vi "TelemetryPRO.vi"() -> ()   [LabVIEW 2017]
uses:
  <vilib>/nican/nican.llb/ncNetAttr.ctl
  <vilib>/Utility/file.llb/Read From Spreadsheet File (string).vi
  <vilib>/Utility/file.llb/Write To Spreadsheet File (string).vi
panel:
  out "Fz Estimation":cluster{i32, i32, i32, i32}(graph)
  out "Array":u8[](array[numeric])
  out "Numeric 2":u8
  out "SlipControl_Enabled":bool
  out "AMK_AV":bool
  out "Torque 2":bool
  out "Offset":i16
  out "Rear Reduction":dbl
  out "BreakPoint":u8
  out "Slope":u16
  out "Damper Travel FR [mm]":dbl
  out "Damper Travel RR [mm]":dbl
  out "Damper Travel FL [mm]":dbl
  in  "Wheel Travel FR":dbl=1000.0
  in  "Wheel Travel FL Offset":dbl=1000.0
  in  "Wheel Travel RR Offset":dbl=1000.0
  out "Damper Travel RL [mm]":dbl
  in  "Wheel Travel RL Offset":dbl=1000.0
  out "HV Cell Voltage":u16(graph)
  out "accY 2":dbl
  out "accZ 2":dbl
  out "TorqRaw 2":u16
  in  "Brake Min 3":dbl=426.0
  out "BPRV":bool
  out "BPFV":bool
  out "BPPS1V":bool
  out "BPPS2V":bool
  out "STA2":bool
  out "STA1":bool
  out "TPS2V":bool
  out "TPS1V":bool
  out "Apps2":dbl
  out "Apps1":dbl
  out "APPS1":u8(slide) scale=0.0..100.0
  out "APPS2":u8(slide) scale=0.0..100.0
  out "brake2":dbl
  out "brake1":dbl
  out "Brake1":u8(slide) scale=0.0..100.0
  out "Brake2":u8(slide) scale=0.0..100.0
  out "Status LEDs Red":bool[](array[boolean])
  out "Status LEDs Green":bool[](array[boolean])
  out "Numeric":dbl
  out "TCU speed":cluster{dbl, "AccelXRaw":dbl, dbl}(graph)
  out "AccelYRaw":dbl
  out "AccelXRaw":dbl
  in  "Acc Y offset":dbl
  in  "Acc X offset 2":dbl
  in  "OffsetFilter":dbl=0.01
  out "IsStopped":bool
  out "Acc Z 2":dbl
  out "Acc X 2":dbl
  out "Roll 2":dbl
  out "Acc Y 2":dbl
  out "Yaw 2":dbl
  in  "Acc Z offset":dbl
  out "Vel_acc":dbl=-0.0098098
  in  "New Lap":bool
  out "Energy":dbl[](array[numeric])
  out "Wheel Travel FL":u16
  out "Wheel Travel FR":u16
  out "Wheel Travel RL":u16
  out "Wheel Travel RR":u16
  out "Acc X":dbl
  out "Roll":dbl
  out "Yaw":dbl
  out "Acc Y":dbl
  out "Acc Z":dbl
  out "accY":dbl
  out "accZ":dbl
  out "Intensity Graph":dbl[][](graph)
  in  "Rollrate offset":dbl
  out "XY Graph 2":cluster{dbl[], dbl[]}(graph)
  out "Derate":bool[](array[boolean])
  out "Torq_sum":dbl
  in  "Play":bool
  in  "Timestep":u32
  in  "stop":bool
  in  "start":bool
  in  "pause":bool
  in  "Progress":i32(slide) min=0 step=60 scale=-1.0..61354011.0 scale format="%.0p"
  out "Time Stamp":string="2\r\n60"
  out "Charge Voltage":dbl
  out "Charge Curr":dbl
  in  "Tab Control":T1(tab)
  in  "Rows to read":i32=60
  in  "Data Path":path=path "D:/__BME-FRT/2016/2016-05-19/2016_05_19_tokol_endurance_00005_00001.csv"
  in  "CAN1 Enable":bool
  in  "CAN0 Enable":bool
  in  "Data Source":u16(ring) items=["Wi-Fi", "CAN-USB", "Log Analysis"]
  in  "Port":u16=8998
  in  "Exit":bool
  in  "Log Path":path=path "D:/__BME-FRT/2016/test.txt"
  in  "Log Enable":bool
  out "WiFi Error":errorcluster
  in  "Length":u16=10
  out "CAN0 Error":errorcluster
  out "CAN1 Error":errorcluster
  out "Log Error":errorcluster
  out "CAN Message":u8[][](array[numeric])=[[2, 1, 128, 63, 0, 0, 129, 162, 129, 155], [2, 17, 23, 61, 0, 1, 0, 0, 0, 0], [3, 64, 252, 0, 0, 0, 27, 55, 27, 0], [2, 16, 115, 16, 37, 0, 203, 0, 0, 0], [4, 17, 23, 61, 0, 1, 0, 0, 0, 0], [2, 0, 128, 44, 0, 0, 136, 1, 7, 207], [2, 1, 128, 63, 0, 0, 129, 162, 129, 155], [2, 17, 23, 61, 0, 1, 0, 0, 0, 0], [4, 34, 0, 33, 0, 30, 0, 0, 0, 0], [4, 80, 148, 60, 128, 0, 0, 0, 0, 0], [1, 116, 84, 128, 0, 0, 190, 127, 8, 37], [2, 16, 116, 15, 111, 0, 203, 0, 0, 0], [1, 120, 211, 127, 0, 0, 193, 158, 8, 215], [1, 180, 84, 128, 0, 0, 223, 126, 2, 100], [1, 124, 0, 0, 0, 0, 189, 126, 8, 75], [1, 184, 62, 128, 2, 15, 59, 127, 2, 219], [4, 17, 23, 61, 0, 1, 0, 0, 0, 0], [1, 188, 0, 0, 0, 0, 136, 158, 2, 110], [2, 0, 128, 44, 0, 0, 136, 1, 7, 207], [2, 1, 128, 63, 0, 0, 129, 162, 129, 155], [2, 17, 23, 61, 0, 1, 0, 0, 0, 0], [3, 64, 252, 0, 0, 0, 27, 55, 27, 0], [4, 48, 10, 15, 219, 0, 96, 0, 0, 0], [3, 49, 128, 255, 0, 0, 0, 0, 0, 0], [2, 16, 117, 0, 0, 0, 203, 0, 0, 0], [4, 17, 23, 61, 0, 1, 0, 0, 0, 0], [2, 0, 128, 44, 0, 0, 136, 1, 7, 207], [2, 1, 128, 63, 0, 0, 129, 162, 129, 155], [2, 17, 23, 61, 0, 1, 0, 0, 0, 0], [3, 32, 112, 255, 0, 0, 0, 0, 0, 0], [4, 34, 0, 30, 0, 31, 0, 0, 0, 0], [1, 116, 87, 128, 0, 0, 184, 127, 9, 218], [1, 120, 203, 127, 1, 37, 194, 158, 9, 222], [2, 16, 118, 0, 0, 0, 205, 0, 0, 0], [1, 124, 0, 0, 0, 0, 176, 126, 9, 211], [1, 180, 90, 128, 0, 0, 215, 126, 3, 116], [1, 184, 50, 128, 3, 19, 44, 127, 3, 114], [4, 17, 23, 61, 0, 1, 0, 0, 0, 0], [1, 188, 0, 0, 0, 0, 147, 158, 3, 235], [2, 0, 128, 43, 0, 0, 136, 1, 7, 207], [2, 1, 128, 63, 0, 0, 129, 162, 129, 155], [2, 17, 23, 61, 0, 1, 0, 0, 0, 0], [3, 64, 252, 0, 0, 0, 38, 55, 38, 0], [2, 16, 119, 0, 0, 0, 202, 0, 0, 0], [4, 17, 23, 61, 0, 1, 0, 0, 0, 0], [2, 0, 128, 43, 0, 0, 136, 2, 7, 207], [2, 1, 128, 63, 0, 0, 129, 162, 129, 155], [2, 17, 23, 61, 0, 1, 0, 0, 0, 0], [4, 34, 0, 20, 0, 26, 0, 0, 0, 0], [1, 116, 78, 128, 0, 0, 179, 127, 10, 75], [1, 120, 206, 127, 2, 57, 194, 158, 10, 132], [2, 16, 120, 16, 37, 0, 200, 0, 210, 0], [1, 180, 90, 128, 0, 0, 206, 126, 4, 188], [1, 124, 0, 0, 0, 0, 157, 126, 10, 65], [1, 184, 39, 128, 4, 3, 33, 127, 4, 7], [4, 17, 23, 61, 0, 1, 0, 0, 0, 0], [1, 188, 0, 0, 0, 0, 153, 158, 4, 183], [2, 0, 128, 43, 0, 0, 136, 2, 7, 207], [2, 1, 128, 63, 0, 0, 129, 162, 129, 155], [2, 17, 23, 61, 0, 1, 0, 0, 0, 0]] format="%02x"
  out "CAN ID":u16[](array[numeric])=[513, 529, 832, 528, 1041, 512, 513, 529, 1058, 1104, 372, 528, 376, 436, 380, 440, 1041, 444, 512, 513, 529, 832, 1072, 817, 528, 1041, 512, 513, 529, 800, 1058, 372, 376, 528, 380, 436, 440, 1041, 444, 512, 513, 529, 832, 528, 1041, 512, 513, 529, 1058, 372, 376, 528, 436, 380, 440, 1041, 444, 512, 513, 529] format="%x"
  out "CAN Message 2":u8[][](array[numeric])=[[2, 1, 128, 63, 0, 0, 129, 162, 129, 155], [2, 17, 23, 61, 0, 1, 0, 0, 0, 0], [3, 64, 252, 0, 0, 0, 27, 55, 27, 0], [2, 16, 115, 16, 37, 0, 203, 0, 0, 0], [4, 17, 23, 61, 0, 1, 0, 0, 0, 0], [2, 0, 128, 44, 0, 0, 136, 1, 7, 207], [2, 1, 128, 63, 0, 0, 129, 162, 129, 155], [2, 17, 23, 61, 0, 1, 0, 0, 0, 0], [4, 34, 0, 33, 0, 30, 0, 0, 0, 0], [4, 80, 148, 60, 128, 0, 0, 0, 0, 0], [1, 116, 84, 128, 0, 0, 190, 127, 8, 37], [2, 16, 116, 15, 111, 0, 203, 0, 0, 0], [1, 120, 211, 127, 0, 0, 193, 158, 8, 215], [1, 180, 84, 128, 0, 0, 223, 126, 2, 100], [1, 124, 0, 0, 0, 0, 189, 126, 8, 75], [1, 184, 62, 128, 2, 15, 59, 127, 2, 219], [4, 17, 23, 61, 0, 1, 0, 0, 0, 0], [1, 188, 0, 0, 0, 0, 136, 158, 2, 110], [2, 0, 128, 44, 0, 0, 136, 1, 7, 207], [2, 1, 128, 63, 0, 0, 129, 162, 129, 155], [2, 17, 23, 61, 0, 1, 0, 0, 0, 0], [3, 64, 252, 0, 0, 0, 27, 55, 27, 0], [4, 48, 10, 15, 219, 0, 96, 0, 0, 0], [3, 49, 128, 255, 0, 0, 0, 0, 0, 0], [2, 16, 117, 0, 0, 0, 203, 0, 0, 0], [4, 17, 23, 61, 0, 1, 0, 0, 0, 0], [2, 0, 128, 44, 0, 0, 136, 1, 7, 207], [2, 1, 128, 63, 0, 0, 129, 162, 129, 155], [2, 17, 23, 61, 0, 1, 0, 0, 0, 0], [3, 32, 112, 255, 0, 0, 0, 0, 0, 0], [4, 34, 0, 30, 0, 31, 0, 0, 0, 0], [1, 116, 87, 128, 0, 0, 184, 127, 9, 218], [1, 120, 203, 127, 1, 37, 194, 158, 9, 222], [2, 16, 118, 0, 0, 0, 205, 0, 0, 0], [1, 124, 0, 0, 0, 0, 176, 126, 9, 211], [1, 180, 90, 128, 0, 0, 215, 126, 3, 116], [1, 184, 50, 128, 3, 19, 44, 127, 3, 114], [4, 17, 23, 61, 0, 1, 0, 0, 0, 0], [1, 188, 0, 0, 0, 0, 147, 158, 3, 235], [2, 0, 128, 43, 0, 0, 136, 1, 7, 207], [2, 1, 128, 63, 0, 0, 129, 162, 129, 155], [2, 17, 23, 61, 0, 1, 0, 0, 0, 0], [3, 64, 252, 0, 0, 0, 38, 55, 38, 0], [2, 16, 119, 0, 0, 0, 202, 0, 0, 0], [4, 17, 23, 61, 0, 1, 0, 0, 0, 0], [2, 0, 128, 43, 0, 0, 136, 2, 7, 207], [2, 1, 128, 63, 0, 0, 129, 162, 129, 155], [2, 17, 23, 61, 0, 1, 0, 0, 0, 0], [4, 34, 0, 20, 0, 26, 0, 0, 0, 0], [1, 116, 78, 128, 0, 0, 179, 127, 10, 75], [1, 120, 206, 127, 2, 57, 194, 158, 10, 132], [2, 16, 120, 16, 37, 0, 200, 0, 210, 0], [1, 180, 90, 128, 0, 0, 206, 126, 4, 188], [1, 124, 0, 0, 0, 0, 157, 126, 10, 65], [1, 184, 39, 128, 4, 3, 33, 127, 4, 7], [4, 17, 23, 61, 0, 1, 0, 0, 0, 0], [1, 188, 0, 0, 0, 0, 153, 158, 4, 183], [2, 0, 128, 43, 0, 0, 136, 2, 7, 207], [2, 1, 128, 63, 0, 0, 129, 162, 129, 155], [2, 17, 23, 61, 0, 1, 0, 0, 0, 0]] format="%02x"
  out "CAN ID 2":u16[](array[numeric])=[513, 529, 832, 528, 1041, 512, 513, 529, 1058, 1104, 372, 528, 376, 436, 380, 440, 1041, 444, 512, 513, 529, 832, 1072, 817, 528, 1041, 512, 513, 529, 800, 1058, 372, 376, 528, 380, 436, 440, 1041, 444, 512, 513, 529, 832, 528, 1041, 512, 513, 529, 1058, 372, 376, 528, 436, 380, 440, 1041, 444, 512, 513, 529] format="%x"
  out "CAN Message 3":u8[][](array[numeric])=[[2, 1, 128, 63, 0, 0, 129, 162, 129, 155], [2, 17, 23, 61, 0, 1, 0, 0, 0, 0], [3, 64, 252, 0, 0, 0, 27, 55, 27, 0], [2, 16, 115, 16, 37, 0, 203, 0, 0, 0], [4, 17, 23, 61, 0, 1, 0, 0, 0, 0], [2, 0, 128, 44, 0, 0, 136, 1, 7, 207], [2, 1, 128, 63, 0, 0, 129, 162, 129, 155], [2, 17, 23, 61, 0, 1, 0, 0, 0, 0], [4, 34, 0, 33, 0, 30, 0, 0, 0, 0], [4, 80, 148, 60, 128, 0, 0, 0, 0, 0], [1, 116, 84, 128, 0, 0, 190, 127, 8, 37], [2, 16, 116, 15, 111, 0, 203, 0, 0, 0], [1, 120, 211, 127, 0, 0, 193, 158, 8, 215], [1, 180, 84, 128, 0, 0, 223, 126, 2, 100], [1, 124, 0, 0, 0, 0, 189, 126, 8, 75], [1, 184, 62, 128, 2, 15, 59, 127, 2, 219], [4, 17, 23, 61, 0, 1, 0, 0, 0, 0], [1, 188, 0, 0, 0, 0, 136, 158, 2, 110], [2, 0, 128, 44, 0, 0, 136, 1, 7, 207], [2, 1, 128, 63, 0, 0, 129, 162, 129, 155], [2, 17, 23, 61, 0, 1, 0, 0, 0, 0], [3, 64, 252, 0, 0, 0, 27, 55, 27, 0], [4, 48, 10, 15, 219, 0, 96, 0, 0, 0], [3, 49, 128, 255, 0, 0, 0, 0, 0, 0], [2, 16, 117, 0, 0, 0, 203, 0, 0, 0], [4, 17, 23, 61, 0, 1, 0, 0, 0, 0], [2, 0, 128, 44, 0, 0, 136, 1, 7, 207], [2, 1, 128, 63, 0, 0, 129, 162, 129, 155], [2, 17, 23, 61, 0, 1, 0, 0, 0, 0], [3, 32, 112, 255, 0, 0, 0, 0, 0, 0], [4, 34, 0, 30, 0, 31, 0, 0, 0, 0], [1, 116, 87, 128, 0, 0, 184, 127, 9, 218], [1, 120, 203, 127, 1, 37, 194, 158, 9, 222], [2, 16, 118, 0, 0, 0, 205, 0, 0, 0], [1, 124, 0, 0, 0, 0, 176, 126, 9, 211], [1, 180, 90, 128, 0, 0, 215, 126, 3, 116], [1, 184, 50, 128, 3, 19, 44, 127, 3, 114], [4, 17, 23, 61, 0, 1, 0, 0, 0, 0], [1, 188, 0, 0, 0, 0, 147, 158, 3, 235], [2, 0, 128, 43, 0, 0, 136, 1, 7, 207], [2, 1, 128, 63, 0, 0, 129, 162, 129, 155], [2, 17, 23, 61, 0, 1, 0, 0, 0, 0], [3, 64, 252, 0, 0, 0, 38, 55, 38, 0], [2, 16, 119, 0, 0, 0, 202, 0, 0, 0], [4, 17, 23, 61, 0, 1, 0, 0, 0, 0], [2, 0, 128, 43, 0, 0, 136, 2, 7, 207], [2, 1, 128, 63, 0, 0, 129, 162, 129, 155], [2, 17, 23, 61, 0, 1, 0, 0, 0, 0], [4, 34, 0, 20, 0, 26, 0, 0, 0, 0], [1, 116, 78, 128, 0, 0, 179, 127, 10, 75], [1, 120, 206, 127, 2, 57, 194, 158, 10, 132], [2, 16, 120, 16, 37, 0, 200, 0, 210, 0], [1, 180, 90, 128, 0, 0, 206, 126, 4, 188], [1, 124, 0, 0, 0, 0, 157, 126, 10, 65], [1, 184, 39, 128, 4, 3, 33, 127, 4, 7], [4, 17, 23, 61, 0, 1, 0, 0, 0, 0], [1, 188, 0, 0, 0, 0, 153, 158, 4, 183], [2, 0, 128, 43, 0, 0, 136, 2, 7, 207], [2, 1, 128, 63, 0, 0, 129, 162, 129, 155], [2, 17, 23, 61, 0, 1, 0, 0, 0, 0]] format="%02x"
  out "CAN ID 3":u16[](array[numeric])=[513, 529, 832, 528, 1041, 512, 513, 529, 1058, 1104, 372, 528, 376, 436, 380, 440, 1041, 444, 512, 513, 529, 832, 1072, 817, 528, 1041, 512, 513, 529, 800, 1058, 372, 376, 528, 380, 436, 440, 1041, 444, 512, 513, 529, 832, 528, 1041, 512, 513, 529, 1058, 372, 376, 528, 436, 380, 440, 1041, 444, 512, 513, 529] format="%x"
  out "STA2":i16
  out "STA1":i16
  out "Max Power":u8
  out "TPS1_Raw":u16
  out "BPS1_Raw":u16
  out "K_Brake":dbl
  out "PD Error Info":u8
  out "Velocity [km/h]":dbl(knob) scale=0.0..120.0
  out "CAN Missing Message":u8[](array[numeric])
  out "Rear 2":dbl
  out "Front 2":dbl
  out "TCU FR":dbl(graph)
  out "TCU RR":dbl(graph)
  out "TCU FL":dbl(graph)
  out "Rear":dbl
  out "Front":dbl
  out "Torque":dbl(slide) scale=0.0..100.0
  out "Brake Encoder":dbl(slide) scale=0.0..100.0
  out "FL":dbl(slide) scale=0.0..2330.0
  in  "Torque Min":dbl
  in  "Torque Max":dbl=1000.0
  in  "Brake Min":dbl
  in  "Brake Max":dbl=1000.0
  out "FL 2":dbl(slide)
  out "FR":dbl(slide) scale=0.0..2330.0
  out "FR 2":dbl(slide)
  out "RL":dbl(slide) scale=0.0..2330.0
  out "RL 2":dbl(slide)
  out "RR":dbl(slide) scale=0.0..2330.0
  out "RR 2":dbl(slide)
  out "Sensor Check":bool[](array[boolean])
  out "Brake Front":dbl(slide)=-0.5082592121982211 scale=0.0..100.0
  out "Brake Rear":dbl(slide)=-0.9529860228716646 scale=0.0..100.0
  in  "Brake Min 2":dbl=350.0
  in  "Brake Max 2":dbl=2000.0
  out "TorqRaw":u16
  out "BrakeRaw":u16
  out "BrakeRaw 2":u16
  out "Boolean":bool
  out "Boolean 2":bool
  out "Boolean 3":bool
  out "Boolean 4":bool
  out "Dial":dbl(knob)=3.0 scale=1.0..12.0
  out "Dial 2":dbl(knob)=11.0 scale=1.0..12.0
  out "Dial 3":dbl(knob)=9.0 scale=1.0..12.0
  out "Dial 4":dbl(knob)=1.0 scale=1.0..12.0
  out "Dial 5":dbl(knob)=1.0 scale=1.0..12.0
  out "Selector":u8
  out "Torque %":u8
  out "Speed RPM":i16
  out "LR Bias":dbl
  out "Regen %":u8
  out "BTC":u8
  out "TCU RR Status":bool[](array[boolean])
  out "TCU RL Status":bool[](array[boolean])
  out "TCU FR Status":bool[](array[boolean])
  out "TCU FL Status":bool[](array[boolean])
  out "Torque [Nm]":dbl(knob) scale=-500.0..1250.0
  out "XY Graph":cluster{dbl[], dbl[]}[](graph)
  out "TCU RL":dbl(graph)
  out "K_Throttle":dbl
  out "BPS2_Raw":u16
  out "BPF_Raw":u16
  out "BPR_Raw":u16
  out "TPS2_Raw":u16
  out "STA2_Raw":u16
  out "STA1_Raw":u16
  out "OFF":bool=TRUE
  out "START":bool
  out "ON":bool
  out "Logging":bool
  in  "Steering Null":dbl=1919.0
  in  "Steering Min":dbl=174.0
  in  "Steering Max":dbl=3565.0
  out "Steering Angle":dbl(slide)=-0.10285714285714287 scale=90.0..-90.0
  out "SteeringRaw":u16
  out "TCU Version":u16
  out "Safety Mode Enabled":bool
  out "Keylock Enable":bool
  out "Slip_TCU":cluster{dbl, dbl, dbl, dbl}(graph)
  out "TCU_acc":cluster{dbl[], dbl[]}[](graph)
  out "Slip":cluster{dbl, dbl, dbl, dbl}(graph)
  out "TCU_ay":dbl
  out "TCU_v":dbl
  out "TCU_ax":dbl
  out "TCU_yaw":dbl
  out "TCU_slipFL":dbl
  out "TCU_slipFR":dbl
  out "TCU_slipRL":dbl
  out "TCU_slipRR":dbl
  out "FL Velocity":dbl
  out "FL Torque Pos":dbl
  out "FL Torque Neg":dbl
  out "FR Velocity":dbl
  out "FR Torque Pos":dbl
  out "FR Torque Neg":dbl
  out "RL Velocity":dbl
  out "RL Torque Pos":dbl
  out "RL Torque Neg":dbl
  out "RR Velocity":dbl
  out "RR Torque Pos":dbl
  out "RR Torque Neg":dbl
  out "MCU RR":cluster{dbl, dbl}(graph)={-0.487060546875, 0.57037353515625}
  out "MCU RL":cluster{dbl, dbl}(graph)={0.743408203125, -0.384521484375}
  out "MCU FR":cluster{dbl, dbl}(graph)={-0.25634765625, -0.205078125}
  out "MCU FL":cluster{dbl, dbl}(graph)={-0.16021728515625, 0.50628662109375}
  out "Actual Velocity\nFL [RPM]":i16
  out "Id FL [A]":dbl
  out "Iq FL [A]":dbl
  out "T Motor FL [°C]":dbl
  out "Error Info FL":u16
  out "Actual Velocity\nFR [RPM]":i16
  out "Id FR [A]":dbl
  out "Iq FR [A]":dbl
  out "Actual Velocity\nRL [RPM]":i16
  out "Id RL [A]":dbl
  out "Iq RL [A]":dbl
  out "Actual Velocity \nRR [RPM]":i16
  out "Id RR [A]":dbl
  out "Iq RR [A]":dbl
  out "Error Info FR":u16
  out "T Motor FR [°C]":dbl
  out "Error Info RL":u16
  out "T Motor RL [°C]":dbl
  out "Error Info RR":u16
  out "T Motor RR [°C]":dbl
  out "Status FL":bool[](array[boolean])
  out "Status FR":bool[](array[boolean])
  out "Status RL":bool[](array[boolean])
  out "Status RR":bool[](array[boolean])
  out "T Inv. FL [°C]":dbl
  out "T Inv. FR [°C]":dbl
  out "T Inv. RR [°C]":dbl
  out "T Inv. RL [°C]":dbl
  out "MCU SC Endline":bool
  out "HVD Interlock":bool
  out "Motor4 Interlock":bool
  out "Motor3 Interlock":bool
  out "Motor2 Interlock":bool
  out "Motor1 Interlock":bool
  out "SC LKS":bool
  out "SC RKS":bool
  out "SC MCU":bool
  out "SC 12V":bool
  out "SC BSPD":bool
  out "SC IMD":bool
  out "SC AMS":bool
  out "SC AIR-":bool
  out "SC AIR+":bool
  out "SC BOTS &\nINS & CKS":bool
  out "SC Motor 3":bool
  out "SC Motor 1":bool
  out "SC Motor 4":bool
  out "SC Motor 2":bool
  out "HVDet":bool
  out "AIR-":bool
  out "AIR+":bool
  out "BOTS & INS & CKS":bool
  out "MCU Interlocks":bool
  out "LKS & RKS":bool
  out "BSPD 5kW":bool
  out "AMS Relay":bool
  out "IMD Relay":bool
  out "BSPD Relay":bool
  out "BSPD Brake":bool
  out "SC Endline":bool
  out "Radiator Cooling":bool
  out "Battery Low":bool
  out "BMS IC Wake":bool
  out "BMS IC Fault":bool
  out "Battery Full":bool
  out "LV Undervoltage":bool
  out "LV Overtemp":bool
  out "SC State":bool
  out "Main Switch":bool
  out "MP Switch":bool
  out "Discharge":bool[](array[boolean])
  out "LV Temp":dbl[](array[numeric])
  out "LV Battery":cluster{"CellSlide":u16, "CellVoltage":u16}[](array[cluster])=[{"CellSlide"=0, "CellVoltage"=0}, {"CellSlide"=0, "CellVoltage"=0}, {"CellSlide"=0, "CellVoltage"=0}, {"CellSlide"=0, "CellVoltage"=0}, {"CellSlide"=0, "CellVoltage"=0}, {"CellSlide"=0, "CellVoltage"=0}, {"CellSlide"=0, "CellVoltage"=0}, {"CellSlide"=0, "CellVoltage"=0}, {"CellSlide"=0, "CellVoltage"=0}, {"CellSlide"=2800, "CellVoltage"=0}, {"CellSlide"=0, "CellVoltage"=0}, {"CellSlide"=0, "CellVoltage"=0}, {"CellSlide"=0, "CellVoltage"=0}, {"CellSlide"=0, "CellVoltage"=0}] {"CellSlide" scale=2800.0..4200.0}
  out "LV Temp":dbl
  out "LV Max":u16
  out "LV Min":u16
  out "LV Cell Voltages":T2(graph)
  out "Overtemp Errors":u16
  out "Undervoltage Errrors":u16
  out "LV Current":cluster{dbl, dbl}(graph)
  out "LV Voltage [V]":dbl format="%#.2g"
  out "12V Current [A]":dbl format="%#.1g"
  out "48V Current [A]":dbl format="%#.1g"
  out "48V system":bool[](array[boolean])
  out "12V system":bool[](array[boolean])
  out "Temp Max 2":dbl
  out "Cell Min 2":u16
  out "BSPD 5kW":bool
  out "BSPD Brake":bool
  out "HVDet":bool
  out "Stack 1":cluster{"CellSlide":u16, "CellVoltage":u16}[](array[cluster]) {"CellSlide" scale=2800.0..4200.0}
  out "Temp 1":dbl[](array[numeric])
  out "Cell Min":u16
  out "Cell Max":u16
  out "Temp Max":dbl
  out "HV Before":dbl
  out "HV After":dbl
  out "HV Current":dbl
  out "SoC [mAh]":dbl
  out "Stack 2":cluster{"CellSlide":u16, "CellVoltage":u16}[](array[cluster]) {"CellSlide" scale=2800.0..4200.0}
  out "Stack 3":cluster{"CellSlide":u16, "CellVoltage":u16}[](array[cluster]) {"CellSlide" scale=2800.0..4200.0}
  out "Stack 4":cluster{"CellSlide":u16, "CellVoltage":u16}[](array[cluster])=[{"CellSlide"=0, "CellVoltage"=0}, {"CellSlide"=0, "CellVoltage"=0}, {"CellSlide"=0, "CellVoltage"=0}, {"CellSlide"=0, "CellVoltage"=0}, {"CellSlide"=0, "CellVoltage"=0}, {"CellSlide"=0, "CellVoltage"=0}, {"CellSlide"=0, "CellVoltage"=0}, {"CellSlide"=0, "CellVoltage"=0}, {"CellSlide"=0, "CellVoltage"=0}, {"CellSlide"=0, "CellVoltage"=0}, {"CellSlide"=0, "CellVoltage"=0}, {"CellSlide"=0, "CellVoltage"=0}, {"CellSlide"=0, "CellVoltage"=0}, {"CellSlide"=0, "CellVoltage"=0}, {"CellSlide"=0, "CellVoltage"=0}, {"CellSlide"=0, "CellVoltage"=0}, {"CellSlide"=0, "CellVoltage"=0}, {"CellSlide"=0, "CellVoltage"=0}, {"CellSlide"=0, "CellVoltage"=0}, {"CellSlide"=0, "CellVoltage"=0}, {"CellSlide"=0, "CellVoltage"=0}, {"CellSlide"=0, "CellVoltage"=0}, {"CellSlide"=2800, "CellVoltage"=0}, {"CellSlide"=2800, "CellVoltage"=0}] {"CellSlide" scale=2800.0..4200.0}
  out "Stack 5":cluster{"CellSlide":u16, "CellVoltage":u16}[](array[cluster])=[{"CellSlide"=2800, "CellVoltage"=0}, {"CellSlide"=0, "CellVoltage"=0}, {"CellSlide"=0, "CellVoltage"=0}, {"CellSlide"=0, "CellVoltage"=0}, {"CellSlide"=0, "CellVoltage"=0}, {"CellSlide"=0, "CellVoltage"=0}, {"CellSlide"=0, "CellVoltage"=0}, {"CellSlide"=0, "CellVoltage"=0}, {"CellSlide"=0, "CellVoltage"=0}, {"CellSlide"=0, "CellVoltage"=0}, {"CellSlide"=0, "CellVoltage"=0}, {"CellSlide"=0, "CellVoltage"=0}, {"CellSlide"=0, "CellVoltage"=0}, {"CellSlide"=0, "CellVoltage"=0}, {"CellSlide"=0, "CellVoltage"=0}, {"CellSlide"=0, "CellVoltage"=0}, {"CellSlide"=0, "CellVoltage"=0}, {"CellSlide"=0, "CellVoltage"=0}, {"CellSlide"=0, "CellVoltage"=0}, {"CellSlide"=0, "CellVoltage"=0}, {"CellSlide"=0, "CellVoltage"=0}, {"CellSlide"=0, "CellVoltage"=0}, {"CellSlide"=0, "CellVoltage"=0}, {"CellSlide"=0, "CellVoltage"=0}] {"CellSlide" scale=2800.0..4200.0}
  out "Stack 6":cluster{"CellSlide":u16, "CellVoltage":u16}[](array[cluster]) {"CellSlide" scale=2800.0..4200.0}
  out "Temp 2":dbl[](array[numeric])
  out "Temp 3":dbl[](array[numeric])
  out "Temp 4":dbl[](array[numeric])
  out "Temp 5":dbl[](array[numeric])
  out "Temp 6":dbl[](array[numeric])
  out "TSAL State":bool
  out "PC State":bool
  out "12V State":bool
  out "AMS error":bool
  out "IMD error":bool
  out "AMS Relay 2":bool
  out "IMD Relay":bool
  out "AIR+":bool
  out "AIR-":bool
  out "BSPD Relay":bool
  out "UV":bool
  out "OV":bool
  out "OT":bool
  out "TS-OV":bool
  out "Place of Error":u16
  out "Value":u16
  out "?":T3(graph)
  out "Angular Speed":T4(graph)
  out "Pedal Signals":cluster{u16, "BrakeRaw":u16}(graph)
  out "Brake Pressure":cluster{dbl, dbl}(graph)={-0.28368794326241137, -0.5319148936170213}
  out "XY Graph 3":cluster{dbl[], dbl[]}[](graph)
  out "HV Cell":cluster{"Cell Max":u16, "Cell Min":u16}(graph)
  out "Current":dbl(graph)
  out "Electric Power":cluster{dbl, dbl}(graph)
  out "HV Voltage":cluster{"HV Before":dbl, "HV After":dbl}(graph)={"HV Before"=594.9, "HV After"=0.1}
  out "HV Cell Temperature":cluster{dbl, dbl}(graph)
  out "Motor Temperature":cluster{dbl, dbl, dbl, dbl}(graph)={1.3, 1.3, 1.6, 1.5}
  out "Inverter Temperature":cluster{dbl, dbl, dbl, dbl}(graph)={1.3, 1.3, 1.6, 1.5}
  out "Radiator Temperature":T5(graph)
  out "S Radiator Left IN":dbl
  out "S Radiator Right OUT":dbl
  out "S Radiator Right IN":dbl
  out "S Radiator Left OUT":dbl
  out "Car standing":bool
  out "SC State":bool
  out "Overvoltage":bool
  out "MODE":bool
  out "XLAT":bool
  out "BLANK":bool
  out "MCU S SC Endl":u16
  out "TSAL":bool
  out "Telemetry":bool
  out "OFF":bool
  out "START":bool
  out "24V rear DC/DC":bool
  out "OFF Button":bool
  out "START Button":bool
  out "ON Button":bool
  out "Power B Current":u32
  out "Power A Current":u32
  out "CAN2 Term.":bool
  out "CAN1 Term.":bool
  out "MCU TSAL":bool
  out "MCU SC Endline 2":bool
  out "MCU FL 4":bool
  out "MCU FL 3":bool
  out "MCU FL 2":bool
  out "Brake Pausability":bool
  out "MCU RF 4":bool
  out "MCU RF 3":bool
  out "MCU RF 2":bool
  out "MCU RF 1":bool
  out "MCU EF2 B":bool
  out "MCU EF2 A":bool
  out "MCU EF B":bool
  out "MCU EF A":bool
  out "24V Power B":bool
  out "Braking":bool
  out "STA2 ADC Null":u16
  out "STA1 ADC Null":u16
  out "Battery Low":bool
  out "BMS IC Awake":bool
  out "BMS IC Error":bool
  out "Battery Full":bool
  out "48V Out 3":bool
  out "LV Undervoltage":bool
  out "LV Overtemp":bool
  out "12V Out 2":bool
  out "12V Out 3":bool
  out "SC State":bool
  out "12V Out 1":bool
  out "Main Switch":bool
  out "MP Switch":bool
  out "12V Out 5":bool
  out "12V Out 4":bool
  out "48V Out 2":bool
  out "48V Out 1":bool
  out "ON":bool
  out "24V front DC/DC":bool
  out "MCU Interlock":bool
  out "TCU Power":bool
  out "RTDS":bool
  out "LKS & RKS":bool
  out "Brake Light":bool
  out "STA2 ADC 90":u16
  out "STA1 ADC 90":u16
  out "BSE2 ADC Max":u16
  out "BSE2 ADC Min":u16
  out "BSE1 ADC Max":u16
  out "BSE1 ADC Min":u16
  out "APPS2 ADC Max":u16
  out "APPS2 ADC Min":u16
  out "APPS1 ADC Max":u16
  out "APPS1 ADC Min":u16
  out "MCU EF":bool
  out "MCU RF":bool
  out "MCU Radiator Left IN":dbl
  out "MCU Radiator Right OUT":dbl
  out "MCU Radiator Right IN":dbl
  out "MCU Radiator Left OUT":dbl
  out "TSAL State 2":bool
  out "PC State 2":bool
  out "Driver Protection":bool
  out "12V Current [mA]":dbl
  out "48V Current [mA]":dbl
  out "Message Arrived 14":bool
  out "Message Arrived 13":bool
  out "Message Arrived 12":bool
  out "Message Arrived 11":bool
  out "Other messages arrived":bool
  out "Message Arrived 2":bool
  out "Message Arrived":bool
  out "RR TargetVelo OverTresh":bool
  out "RR TorqueLimNeg UnderTresh":bool
  out "RR TorqueLimNeg OverTresh":bool
  out "RR TorqueLimPos UnderTresh":bool
  out "RR TorqueLimPos OverTresh":bool
  out "RR TargetVelo UnderTresh":bool
  out "RL TargetVelo OverTresh":bool
  out "RL TorqueLimNeg UnderTresh":bool
  out "RL TorqueLimNeg OverTresh":bool
  out "RL TorqueLimPos UnderTresh":bool
  out "RL TorqueLimPos OverTresh":bool
  out "RL TargetVelo UnderTresh":bool
  out "FR TargetVelo OverTresh":bool
  out "FR TorqueLimNeg UnderTresh":bool
  out "FR TorqueLimNeg OverTresh":bool
  out "FR TorqueLimPos UnderTresh":bool
  out "FR TorqueLimPos OverTresh":bool
  out "FR TargetVelo UnderTresh":bool
  out "FL TargetVelo OverTresh":bool
  out "FL TorqueLimNeg UnderTresh":bool
  out "FL TorqueLimNeg OverTresh":bool
  out "FL TorqueLimPos UnderTresh":bool
  out "FL TorqueLimPos OverTresh":bool
  out "FL TargetVelo UnderTresh":bool
  out "Error Throttle Plausability":bool
  out "Error Throttle Validity 2":bool
  out "Error Throttle Validity 1":bool
  out "Error Throttle Position 2":bool
  out "Error Throttle Position 1":bool
  out "Error Rot Switch 5":bool
  out "Error Rot Switch 4":bool
  out "Error Rot Switch 3":bool
  out "Error Rot Switch 2":bool
  out "Error Rot Switch 1":bool
  out "Error Pedalbox Heartbeat":bool
  out "Error Steering Heartbeat":bool
  out "Error Brake Plausability":bool
  out "Error Brake Validity 2":bool
  out "Error Brake Validity  1":bool
  out "Error Brake Position 2":bool
  out "Error Brake Position 1":bool
  out "Error_Button_4":bool
  out "Error_Button_3":bool
  out "Error_Button_2":bool
  out "Error_Button_1":bool
  out "Error Steering Plausability":bool
  out "Error Steering Validity 2":bool
  out "Error Steering Validity 1":bool
  out "Error Steering Angle 2":bool
  out "Error Steering Angle 1":bool
  out "Error Cell Temperature":bool
  out "Error Cell Voltage Sensor":bool
  out "Error Cell Voltage":bool
  out "Error HV Accu. Current":bool
  out "Error HV Accu. Voltage":bool
  out "Error Actual Velocity RR":bool
  out "Error Actual Velocity RL":bool
  out "Error Actual Velocity FR":bool
  out "Error Actual Velocity FL":bool
  out "Error_SteeringControl_Heartbeat_raw":bool
  out "Error_Pedalbox_Heartbeat_raw":bool
  out "Error_SteeringAngleValidity_2_raw":bool
  out "Error_SteeringAngleValidity_1_raw":bool
  out "Error_ThrottleValidity_2_raw":bool
  out "Error_ThrottleValidity_1_raw":bool
  out "Error_BrakeValidity_2_raw":bool
  out "Error_BrakeValidity_1_raw":bool
  out "Error_LVCellTemperature":bool
  out "Error_LVCellVoltage":bool
  out "Error BrPressure Rear Validity_raw":bool
  out "Error BrPressure Front Validity_raw":bool
  out "Error BrPressure Rear 2":bool
  out "Error BrPressure Front":bool
  out "Error BrPressure Rear Validity":bool
  out "Error BrPressure Front Validity":bool
  out "CriticalHVCell Heartbeat":bool
  out "CriticalHVCell Heartbeat raw":bool
  out "Error_BrakeValidity_1_raw  2":bool
  out "Error_BrakeValidity_2_raw 2":bool
  out "Error_ThrottleValidity_1_raw 2":bool
  out "Error_ThrottleValidity_2_raw 2":bool
  out "Error_SteeringAngleValidity_1_raw 2":bool
  out "Error_SteeringAngleValidity_2_raw 2":bool
  out "SensorBox_Rear_RangeCheck":bool
  out "Sensorbox_Plausibility_Check":bool
  out "SensorBox_Front_RangeCheck":bool
  out "Hardcore Time":dbl
  out "PowerLimiter Approx":dbl
  out "Hardcoremode ON":bool
  out "Smooth_Transition_Enabled":bool
  out "Drop":dbl
  out "Torque_Derate":bool
  out "Torque_Coeff":bool
  out "Throttle_Constant":bool
  out "Power Limiter Enabled":bool
  out "Yaw Rear":dbl(graph)
  out "Yaw Front":dbl(graph)
  out "Slip":dbl(graph)
  out "Characteristics Approx":u8
  out "Tune":dbl
  out "Wheel Travel":cluster{"y_":dbl, "y_":dbl, "y_":dbl, "y_":dbl}(graph)
  out "Fz_FR":i32
  out "Fz_RL":i32
  out "Fz_FL":i32
  out "Fz_RR":i32
  out "YawControlSelector":i32
  out "Weight":i32
  out "Efficiency":dbl
  out "Yaw_Control_ON":bool
  out "Fx_Divide_ON":bool
  out "Eff_PowLim":bool
  out "DesiredSlipRate":dbl format="%.2f"
  out "Voltage Limit":dbl
  out "Current Limit":dbl
  # "SlipControl"
  # "HV    LV BPSD IMD AMS  FL    FR    RL   RR"
  # "SystemReady : 1 ha van 24V és felállt a belsõ rendszer\nError : 1 ha valamilyen error van\nWarn : 1 ha warning van\nQuitDcOn : DcOn visszajelzõje, hogy ténylegesen engedélyezte-e a HV-t, és hogy van is HV\nDcOn : TCU küldi CAN-en, hogy engedélyezze a HV bemenetet, CAN-en beolvasott értéket írja itt ki\nQuitInverterOn : az inverterek tényleges állapota, 1 ha aktívak, azaz a fizikai engedélyezõ jelek is aktívak\nInverterOn : TCU küldi, inverter engedélyezõ jel, azt küldi amit CAN-rõl beolvasott\nDerating : valamilyen derating állapotban van"
  # "Wi-Fi"
  # "CAN-USB"
  # "Log Analysis"
  # "TPS1"
  # "STA1"
  # "TPS2"
  # "STA1"
  # "STA2"
  # "STA2"
  # "BPS1"
  # "Throttle Bias"
  # "STA1 raw"
  # "BPS2"
  # "BPF"
  # "Regen Bias"
  # "STA2 raw"
  # "BPR"
  # "InverterOn"
  # "InverterOn"
  # "InverterOn"
  # "InverterOn"
  # "DcOn"
  # "DcOn"
  # "DcOn"
  # "DcOn"
  # "Enable"
  # "Enable"
  # "Enable"
  # "Enable"
  # "ErrorReset"
  # "ErrorReset"
  # "ErrorReset"
  # "ErrorReset"
  # "SysReady"
  # "SysReady"
  # "SysReady"
  # "SysReady"
  # "Error"
  # "Error"
  # "Error"
  # "Error"
  # "Warn"
  # "Warn"
  # "Warn"
  # "Warn"
  # "QuitDcOn"
  # "QuitDcOn"
  # "QuitDcOn"
  # "QuitDcOn"
  # "DcOn"
  # "DcOn"
  # "DcOn"
  # "DcOn"
  # "QuitInvOn"
  # "QuitInvOn"
  # "QuitInvOn"
  # "QuitInvOn"
  # "InverterOn"
  # "InverterOn"
  # "InverterOn"
  # "InverterOn"
  # "Derating"
  # "Derating"
  # "Derating"
  # "Derating"
  # "HV Accumulator ECU"
  # "Pedalbox"
  # "LV Sys ECU"
  # "MCU Power ECU"
  # "MCU Support ECU"
  # "Dashboard"
  # "APPS Error"
  # "BPPS Error"
  # "Steering Error"
  # "HV Accumulator Error"
  # "Rotary Switch Error"
  # "MCU Error"
  # "Button Error"
  # "Noheartbeat Error"
  # "FR AMK Error"
  # "RL AMK Error"
  # "FL AMK Error"
  # "RR AMK Error"
  # "Sensorbox Error"
  # "LV Accumulator Error"
  # "Brake Pressure Error"
  # "Powerlimiter"
  # "Characteristics Approx"
  # "Smooth Transition"
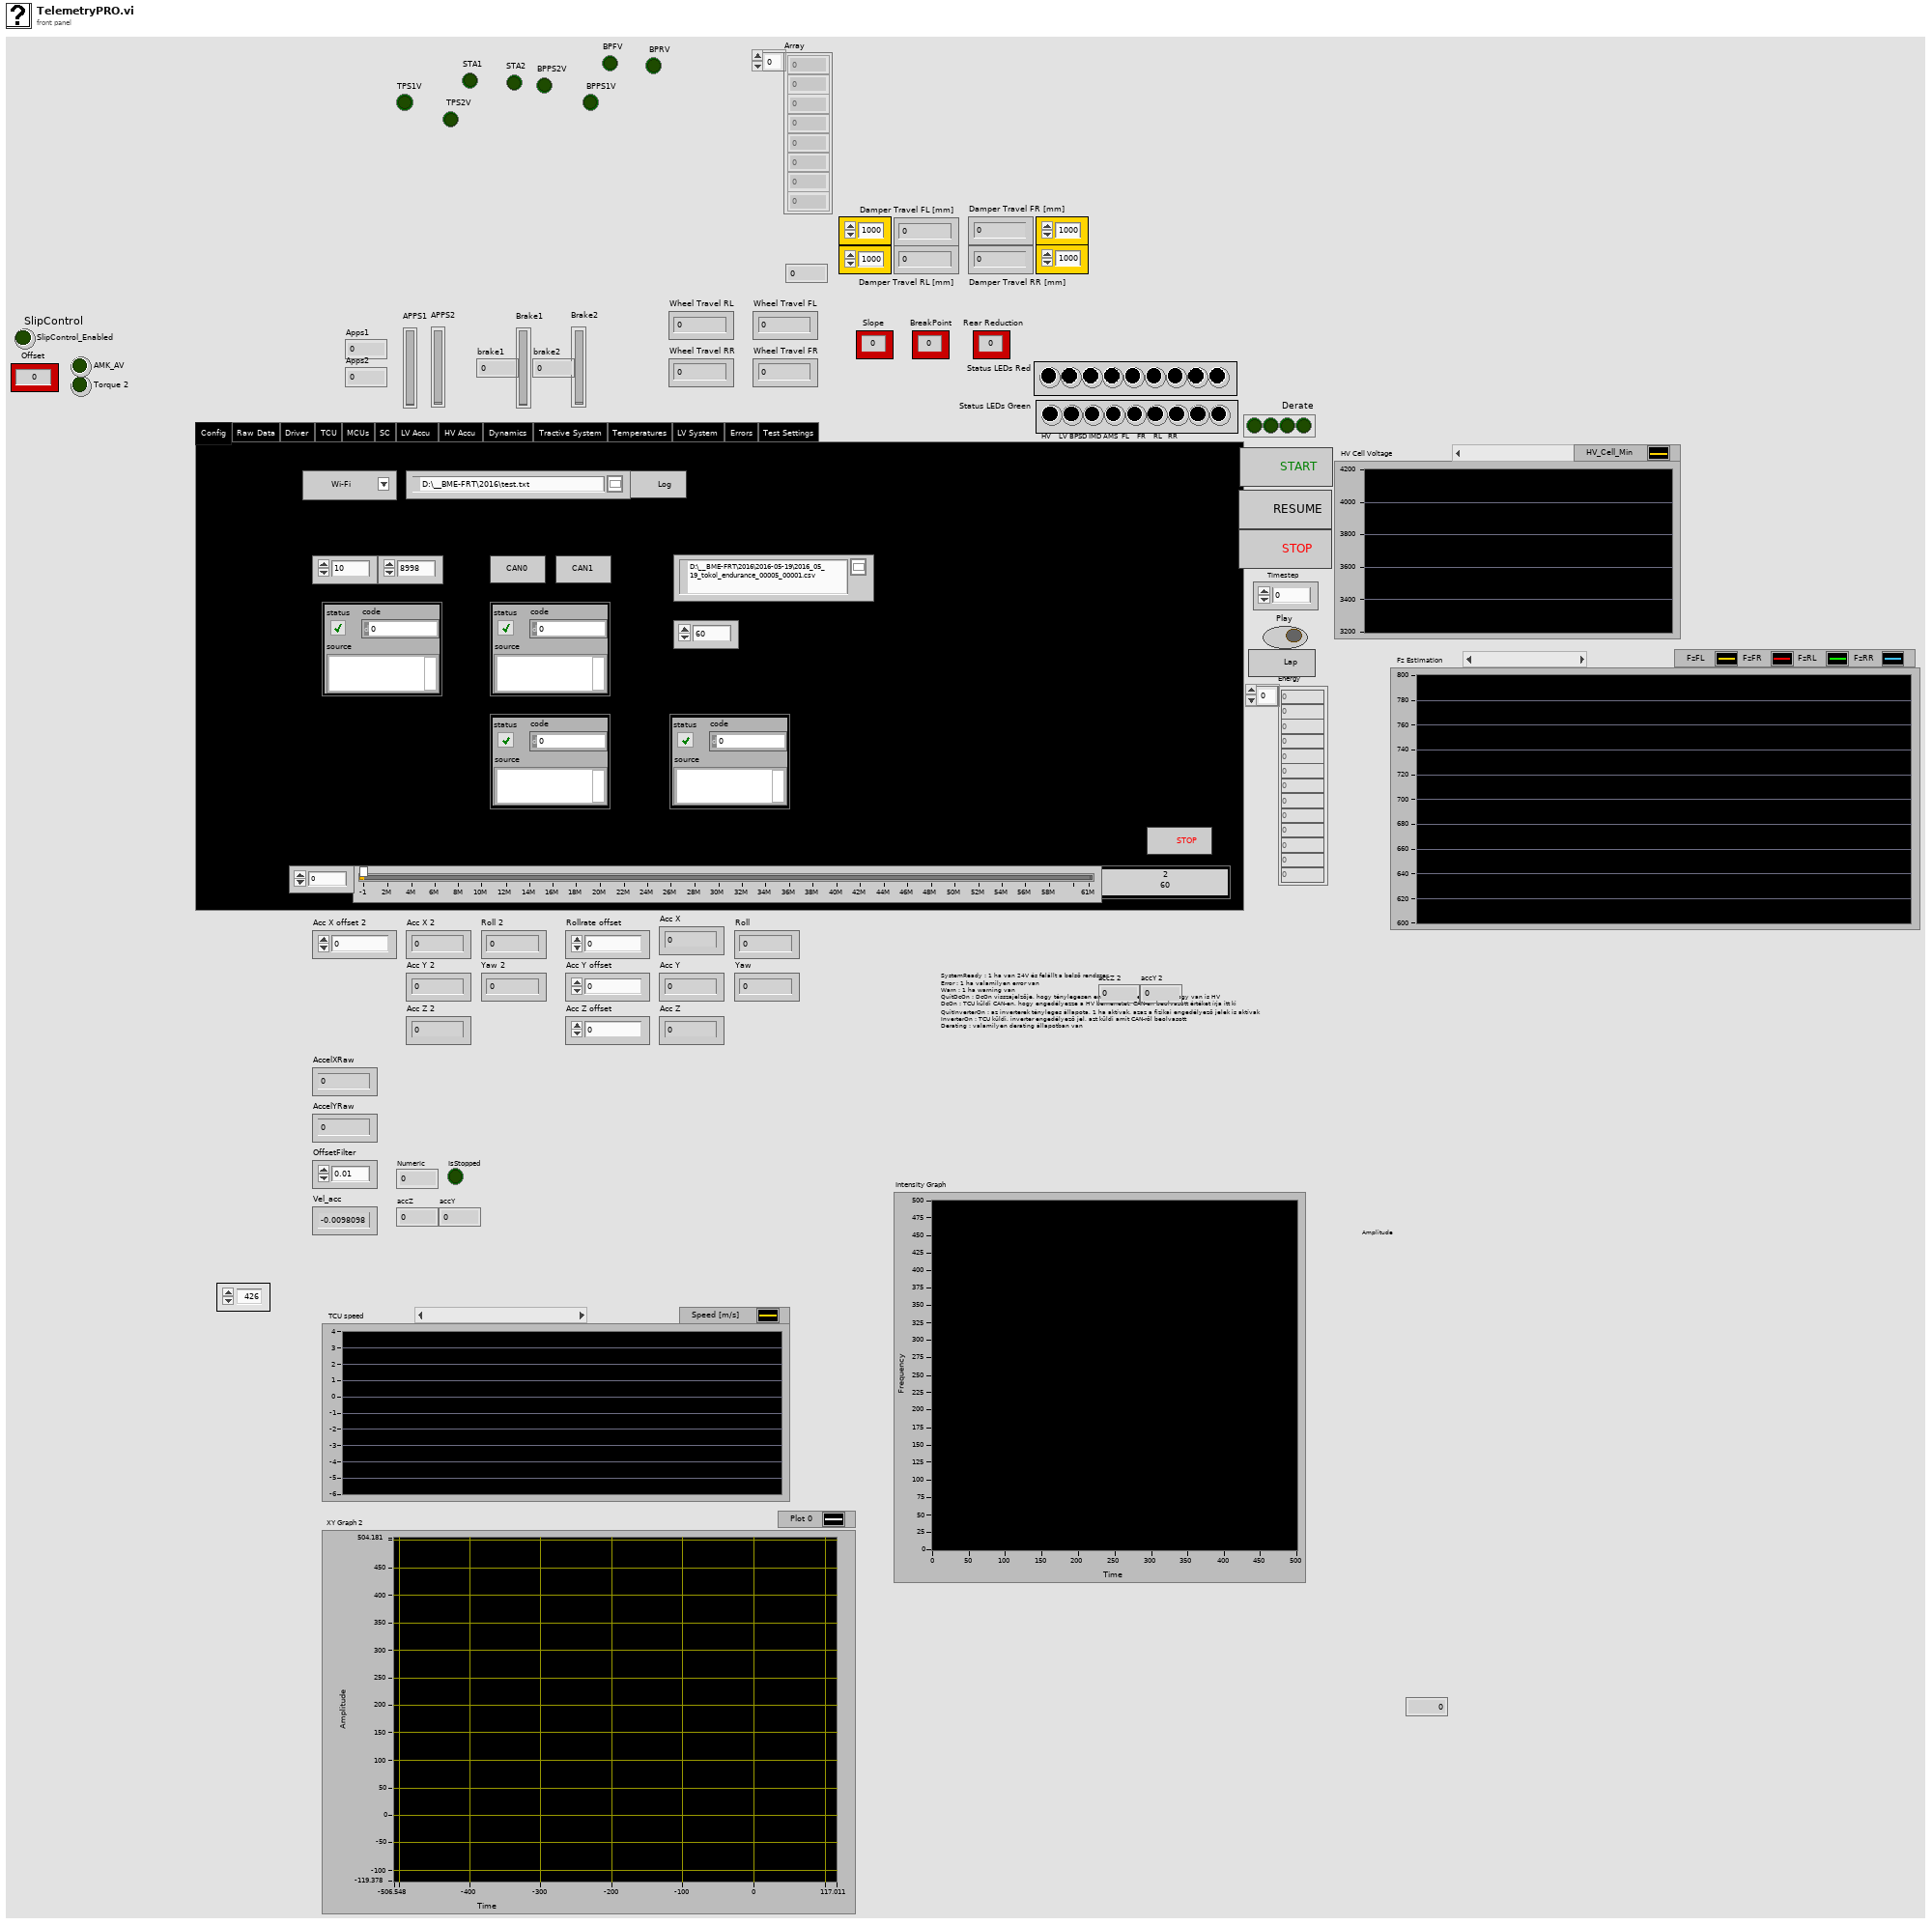
[diagram p1: front panel]
types:
  T1 = enum32{"Config", "Raw Data", "Driver", "TCU", "MCUs", "SC", "LV Accu", "HV Accu", "Dynamics", "Tractive System", "Temperatures", "LV System", "Errors", "Test Settings"}
  T2 = cluster{"[0]":u16, "[1]":u16, "[2]":u16, "[3]":u16, "[4]":u16, "[5]":u16, "[6]":u16, "[7]":u16, "[8]":u16}
  T3 = cluster{"Velocity [km/h]":dbl, "Torque":dbl, dbl, dbl}
  T4 = cluster{"Actual Velocity (RPM)":i16, "Actual Velocity (RPM) 2":i16, "Actual Velocity (RPM) 3":i16, "Actual Velocity (RPM) 4":i16}
  T5 = cluster{"y_":dbl, "y_":dbl, "y_":dbl, "y_":dbl, "y_":dbl, "y_":dbl, "y_":dbl, "y_":dbl}
  T6 = typedef "ncNetAttr.ctl" = cluster{"Start On Open":enum32{"FALSE", "TRUE"}, "Baud Rate":u32, "Read Queue Length":u32, "Write Queue Length":u32, "Standard Comparator":u32, "Standard Mask":u32, "Extended Comparator":u32, "Extended Mask":u32}
  T7 = typedef "xobjhandle.ctl" = u32
  T8 = cluster{"Actual Velocity\nFL [RPM]":i16, "Actual Velocity\nFR [RPM]":i16, "Actual Velocity\nRL [RPM]":i16, "Actual Velocity \nRR [RPM]":i16}
  T9 = cluster{"T Inv. FL [°C]":dbl, "T Inv. FR [°C]":dbl, "T Inv. RL [°C]":dbl, "T Inv. RR [°C]":dbl}
  T10 = cluster{"T Motor FL [°C]":dbl, "T Motor FR [°C]":dbl, "T Motor RL [°C]":dbl, "T Motor RR [°C]":dbl}
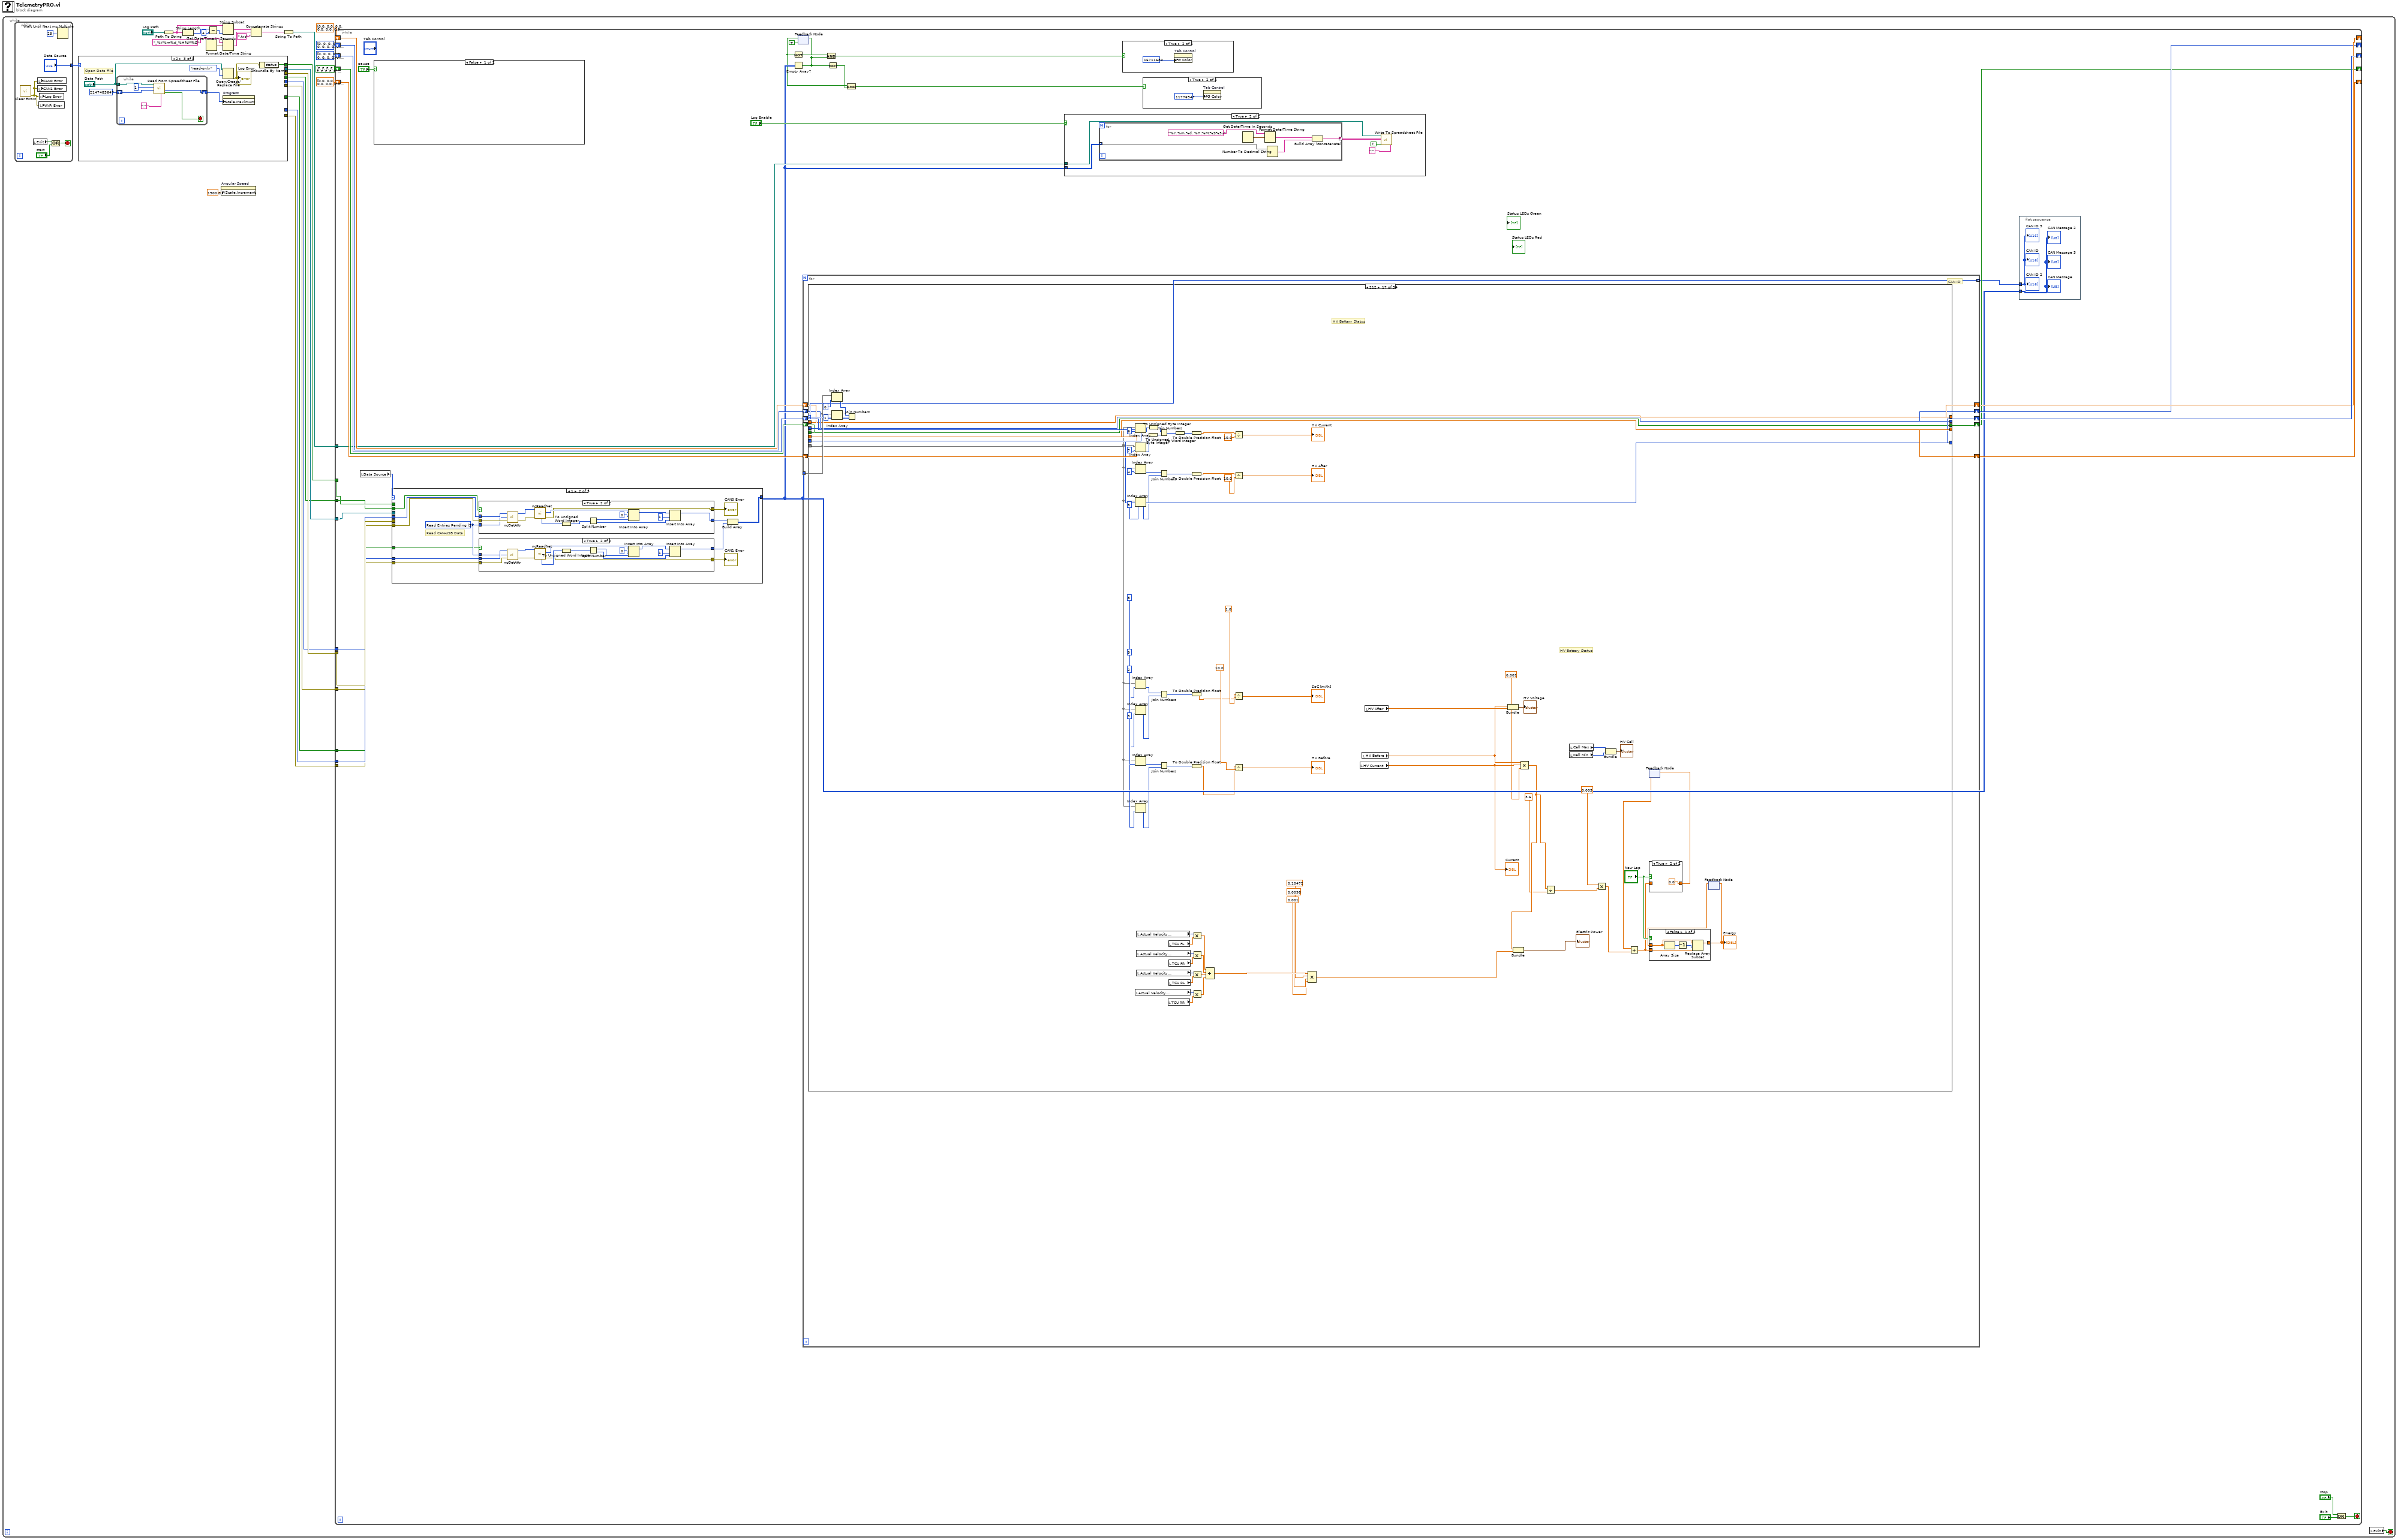
[diagram p0: block diagram]
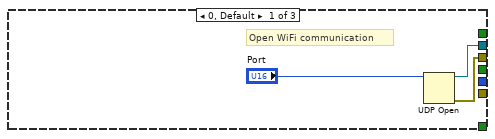
[diagram p2: hidden frame]
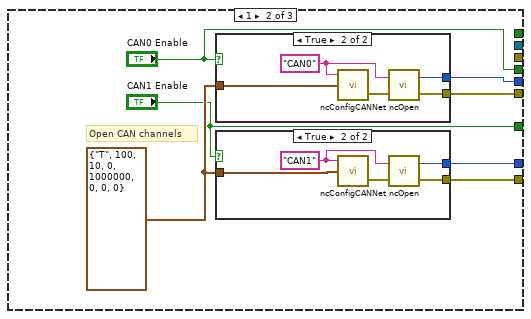
[diagram p3: hidden frame]
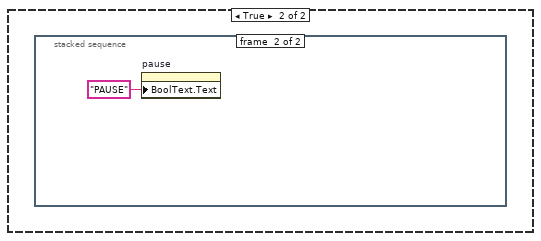
[diagram p6: hidden frame]
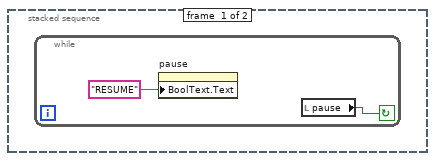
[diagram p7: hidden frame]
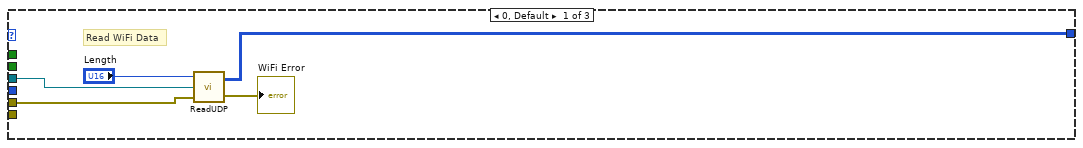
[diagram p10: hidden frame]
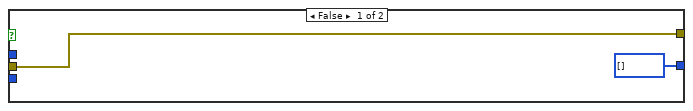
[diagram p11: hidden frame]
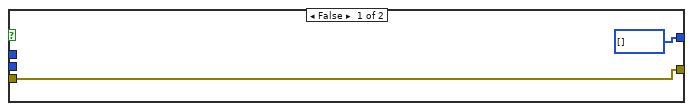
[diagram p12: hidden frame]
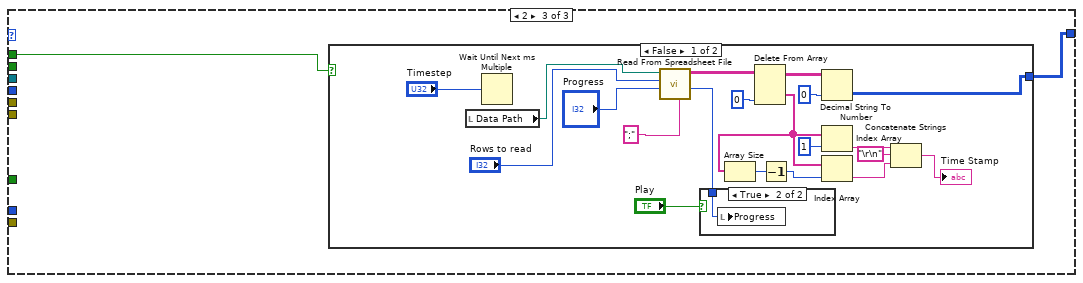
[diagram p13: hidden frame]
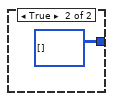
[diagram p15: hidden frame]
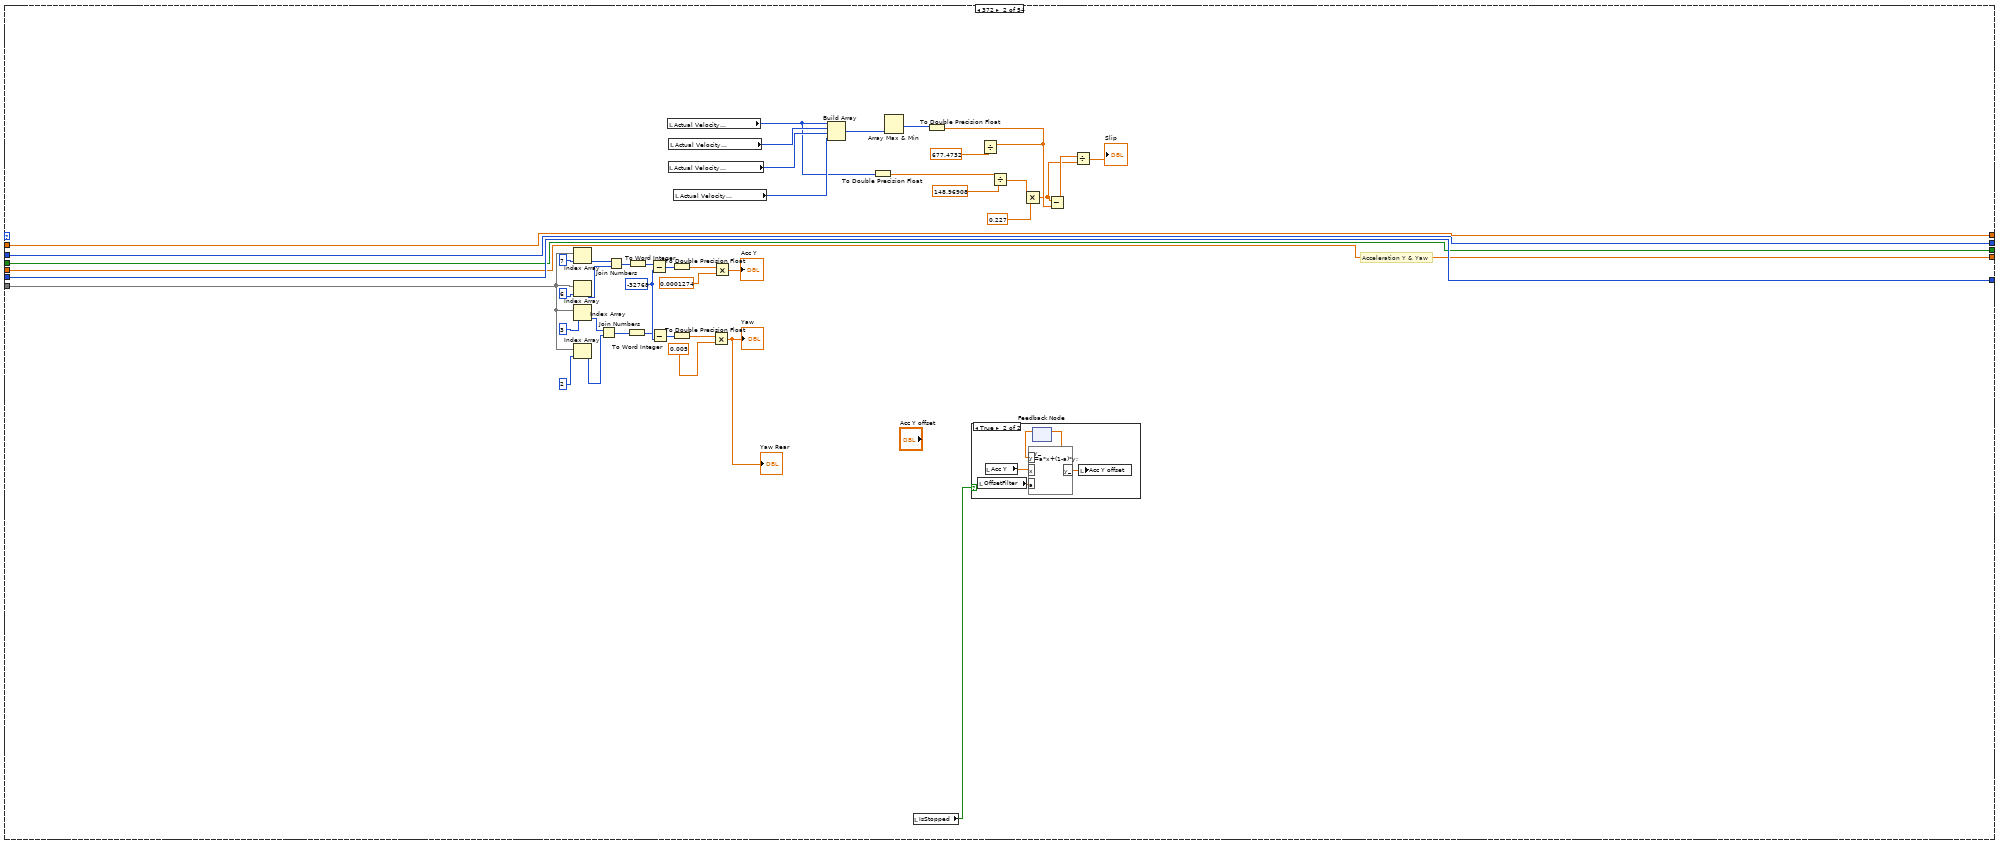
[diagram p18: hidden frame]
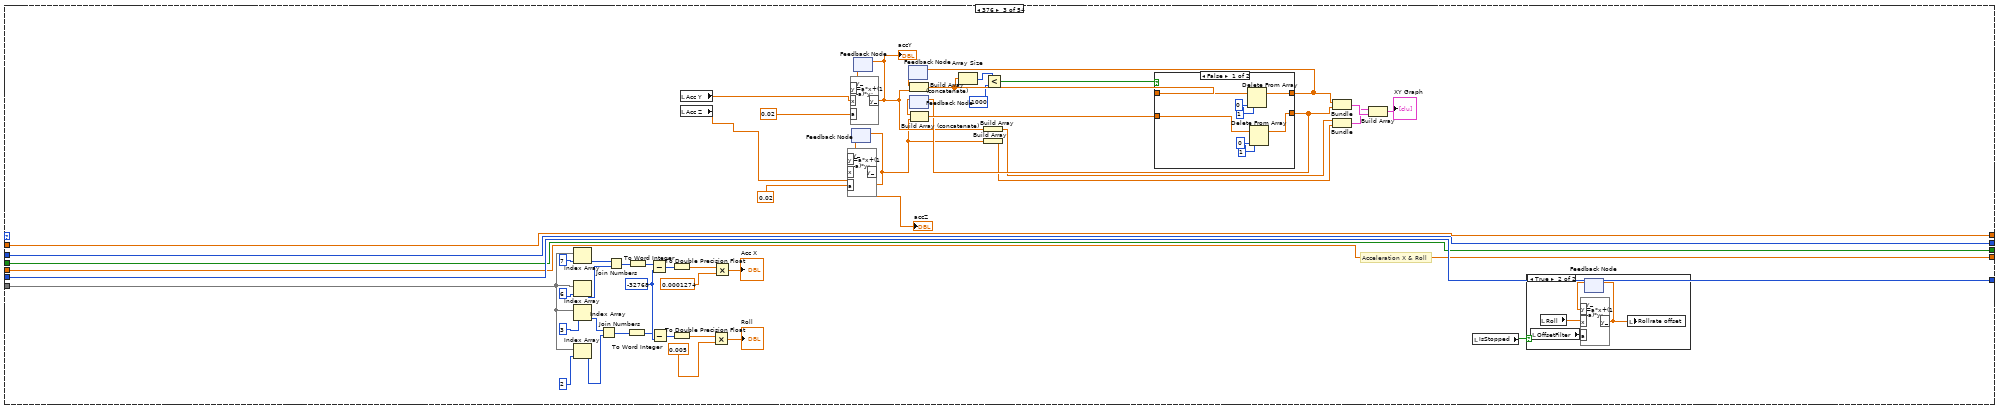
[diagram p20: hidden frame]
diagram:
  n1 = while {
    stop <- w2 stop-if-true
    n2 = while {
      tunnel: ["Data Source"] -> w3
      stop <- w31 stop-if-true
      n3 = call <vilib>:"Clear Errors.vi"() -> ("error out"=w30:errorcluster)  [unwired: 6 in, 1 out]
      n4 = local read "Exit"() -> (w32:bool)
      n5 = local write "CAN0 Error"(w30) -> ()
      n6 = local write "CAN1 Error"(w30) -> ()
      n7 = local write "WiFi Error"(w30) -> ()
      n8 = local write "Log Error"(w30) -> ()
      n9 = Compound Arithmetic op=OR(w32, "start") -> (w31:bool)
      n10 = Wait Until Next ms Multiple(millisecond multiple=u32 25) -> ()  [unwired: 1 out]
    }
    n11 = case shown="2" w3 {
      tunnel: [_ w45 _] -> w7
      tunnel: [_ w44 _] -> w8
      tunnel: [_ w43 _] -> w10
      tunnel: [_ w42 _] -> w9
      tunnel: [w37 _ _] -> w12
      tunnel: [w36 _ _] -> w11
      tunnel: [_ "CAN0 Enable" _] -> w6
      tunnel: [_ "CAN1 Enable" _] -> w5
      tunnel: [_ _ w59] -> w4
      frame 0, Default {
        # "Open WiFi communication"
        n12 = UDP Open(11:"Port") -> (port=w37:refnum<k16>, 0:w36:errorcluster)  [unwired: 4 in, 1 out]
      }
      frame 1 {
        w41 = T6 {"Start On Open"=enum."TRUE", "Baud Rate"=100, "Read Queue Length"=10, "Write Queue Length"=0, "Standard Comparator"=1000000, "Standard Mask"=0, "Extended Comparator"=0, "Extended Mask"=0} ("CAN Network Interface Config")
        # "Open CAN channels"
        n13 = case shown="True" "CAN0 Enable" {
          tunnel: w41 -> [_ w53]
          tunnel: [_ w52] -> w45
          tunnel: [_ w51] -> w44
          frame False {
          }
          frame True {
            w54 = "CAN0" ("ObjName")
            n14 = call <vilib>:"ncConfigCANNet.vi"("CAN Network Interface Config"=w53, "ObjName"=w54) -> ("Error out"=w55:errorcluster)  [unwired: 3 in]
            n15 = call <vilib>:"ncOpen.vi"("Error in"=w55, "ObjName"=w54) -> ("Error out"=w51:errorcluster, "ObjHandle out"=w52:T7)
          }
        }
        n16 = case shown="True" "CAN1 Enable" {
          tunnel: [_ w48] -> w43
          tunnel: [_ w47] -> w42
          tunnel: w41 -> [_ w46]
          frame False {
          }
          frame True {
            w50 = "CAN1" ("ObjName")
            n17 = call <vilib>:"ncConfigCANNet.vi"("CAN Network Interface Config"=w46, "ObjName"=w50) -> ("Error out"=w49:errorcluster)  [unwired: 3 in]
            n18 = call <vilib>:"ncOpen.vi"("Error in"=w49, "ObjName"=w50) -> ("Error out"=w47:errorcluster, "ObjHandle out"=w48:T7)
          }
        }
      }
      frame 2 {
        # "Open Data File"
        n19 = while {
          tunnel: "Data Path" -> [w67]
          shift-right: [w63] -> w57
          shift-left: 2147483647 ("mark after read (chars.)") -> [w64]
          stop <- w65 stop-if-true
          n20 = call-poly <vilib>:"Read From Spreadsheet File.vi"("delimiter (\\t)"=";" ("delimiter (\\t)"), "start of read offset (chars.:0)"=w64, "number of rows (all:-1)"=1, "file path (dialog if empty)"=w67) -> ("EOF?"=w65:bool, "mark after read (chars.)"=w63:i32)  [unwired: 3 in, 3 out]
        }
        n21 = Open/Create/Replace File(file path (use dialog)="Data Path", access (0:read/write)=enum16{"read/write", "read-only", "write-only"}."read-only") -> (error out=w60:errorcluster)  [unwired: 4 in, 2 out]
        "Log Error" <- w60
        n22 = property on="Progress" class="Slide (strict)"("Scale.Maximum"=w57) -> ()  [unwired: 2 in, 2 out]
        n23 = Unbundle By Name(w60) -> ("status"=w59:bool)
      }
    }
    n24 = Path To String(path="Log Path") -> (string=w21:string)
    n25 = String Length(string=w21) -> (length=w20:i32)
    n26 = Get Date/Time In Seconds() -> (seconds since 1Jan1904=w23:timestamp)
    n27 = Subtract(x=w20, y=4) -> (x-y=w18:i32)
    n28 = property on="Angular Speed" class="WFChart (strict)"("YScale.Increment"=1500.0 ("Y Scale.Range:Increment")) -> ()  [unwired: 2 in, 2 out]
    n29 = String Subset(string=w21, length (rest)=w18) -> (substring=w15:string)  [unwired: 1 in]
    n30 = Format Date/Time String(time format string (%c)="_%Y%m%d_%H%M%S", seconds (now)=w23) -> (date/time string=w14:string)  [unwired: 1 in]
    n31 = Concatenate Strings(w15, w14, ".txt" ("string")) -> (w16:string)
    n32 = String To Path(string=w16) -> (path=w24:path)
    n33 = while {
      tunnel: w12 -> [w101]
      tunnel: w11 -> [w102]
      shift-right: [w99] -> _
      shift-left: u16[] [0, 0, 0, 0, 0, 0, 0, 0, 0, 0, 0, 0, 0, 0, 0, 0, 0, 0, 0, 0, 0, 0, 0, 0, 0, 0, 0, 0, 0, 0, 0, 0, 0, 0, 0, 0, 0, 0, 0, 0, 0, 0, 0, 0, 0, 0, 0, 0, 0, 0, 0, 0, 0, 0, 0, 0, 0, 0, 0, 0, 0, 0, 0, 0, 0, 0, 0, 0, 0, 0, 0, 0, 0, 0, 0, 0, 0, 0, 0, 0, 0, 0, 0, 0, 0, 0, 0, 0, 0, 0, 0, 0, 0, 0, 0, 0, 0, 0, 0, 0, 0, 0, 0, 0, 0, 0, 0, 0, 0, 0, 0, 0, 0, 0, 0, 0, 0, 0, 0, 0, 0, 0, 0, 0, 0, 0, 0, 0, 0, 0, 0, 0, 0, 0, 0, 0, 0, 0, 0, 0, 0, 0, 0, 0, 0, 0, 0, 0, 0, 0, 0, 0, 0, 0, 0, 0, 0, 0, 0, 0, 0, 0, 0, 0, 0, 0, 0, 0, 0, 0, 0, 0, 0, 0, 0, 0, 0, 0, 0, 0, 0] -> [w100]
      shift-right: [w98] -> _
      shift-left: dbl[] [0.0, 0.0, 0.0, 0.0, 0.0, 0.0, 0.0, 0.0, 0.0, 0.0, 0.0, 0.0, 0.0, 0.0, 0.0, 0.0, 0.0, 0.0, 0.0, 0.0, 0.0, 0.0, 0.0, 0.0, 0.0, 0.0, 0.0, 0.0, 0.0, 0.0, 0.0, 0.0, 0.0, 0.0, 0.0, 0.0, 0.0, 0.0, 0.0, 0.0, 0.0, 0.0, 0.0, 0.0, 0.0, 0.0, 0.0, 0.0, 0.0, 0.0, 0.0, 0.0, 0.0, 0.0, 0.0, 0.0, 0.0, 0.0, 0.0, 0.0, 0.0, 0.0, 0.0, 0.0, 0.0, 0.0, 0.0, 0.0, 0.0, 0.0, 0.0, 0.0, 0.0, 0.0, 0.0, 0.0, 0.0, 0.0, 0.0, 0.0, 0.0, 0.0, 0.0, 0.0, 0.0, 0.0, 0.0, 0.0, 0.0, 0.0, 0.0, 0.0, 0.0, 0.0, 0.0, 0.0, 0.0, 0.0, 0.0, 0.0, 0.0, 0.0, 0.0, 0.0, 0.0, 0.0, 0.0, 0.0, 0.0, 0.0, 0.0, 0.0, 0.0, 0.0, 0.0, 0.0, 0.0, 0.0, 0.0, 0.0, 0.0, 0.0, 0.0, 0.0, 0.0, 0.0, 0.0, 0.0, 0.0, 0.0, 0.0, 0.0, 0.0, 0.0, 0.0, 0.0, 0.0, 0.0, 0.0, 0.0, 0.0, 0.0, 0.0, 0.0, 0.0, 0.0, 0.0, 0.0, 0.0, 0.0, 0.0, 0.0, 0.0, 0.0, 0.0, 0.0, 0.0, 0.0, 0.0, 0.0, 0.0, 0.0, 0.0, 0.0, 0.0, 0.0, 0.0, 0.0, 0.0, 0.0, 0.0, 0.0, 0.0, 0.0, 0.0, 0.0, 0.0, 0.0, 0.0, 0.0, 0.0] -> [w97]
      shift-right: [w93] -> _
      shift-left: u16[] [0, 0, 0, 0, 0, 0, 0, 0, 0, 0, 0, 0, 0, 0] -> [w94]
      shift-right: [w92] -> _
      shift-left: bool[] [FALSE, FALSE, FALSE, FALSE, FALSE, FALSE, FALSE, FALSE, FALSE, FALSE, FALSE, FALSE, FALSE, FALSE] -> [w95]
      shift-right: [w91] -> _
      shift-left: dbl[] [0.0, 0.0, 0.0, 0.0, 0.0, 0.0, 0.0, 0.0, 0.0, 0.0, 0.0, 0.0, 0.0, 0.0] -> [w96]
      tunnel: w24 -> [w88]
      tunnel: w10 -> [w86]
      tunnel: w9 -> [w85]
      tunnel: w8 -> [w84]
      tunnel: w7 -> [w83]
      tunnel: w6 -> [w68]
      tunnel: w5 -> [w82]
      tunnel: w4 -> [w74]
      stop <- w70 stop-if-true
      n34 = local read "Data Source"() -> (w87:u16)
      n35 = case shown="False" "pause" {
        frame False {
        }
        frame True {
          n36 = stacked-sequence {
            frame #0 {
              n37 = while {
                stop <- w104 continue-if-true
                n38 = property on="pause" class="Bool (strict)"("BoolText.Text"="RESUME" ("Boolean Text.Text")) -> ()  [unwired: 2 in, 2 out]
                n39 = local read "pause"() -> (w104:bool)
              }
            }
            frame #1 {
              n40 = property on="pause" class="Bool (strict)"("BoolText.Text"="PAUSE" ("Boolean Text.Text")) -> ()  [unwired: 2 in, 2 out]
            }
          }
        }
      }
      n41 = case shown="1" w87 {
        tunnel: w102 -> [w110 _ _]
        tunnel: w101 -> [w111 _ _]
        tunnel: [w109 w119 w160] -> w81
        tunnel: w86 -> [_ w124 _]
        tunnel: w85 -> [_ w117 _]
        tunnel: w84 -> [_ w123 _]
        tunnel: w83 -> [_ w122 _]
        tunnel: w68 -> [_ w114 _]
        tunnel: w82 -> [_ w113 _]
        tunnel: w74 -> [_ _ w159]
        frame 0, Default {
          # "Read WiFi Data"
          n42 = call "ReadUDP.vi"("error in (no error)"=w110, "connection ID"=w111, "Message length"="Length") -> ("error out"=→"WiFi Error":errorcluster, "Array"=w109:u8[][])
        }
        frame 1 {
          w116 = u32 5 items=["(reserved)", "Protocol Version", "Software Version", "Object State", "(reserved)", "Read Entries Pending", "Write Entries Pending", "ReadMult Size for Notification", "Listen Only?", "Self Reception?", "Transmit Error Counter", "Receive Error Counter", "Single Shot Transmit?", "Series 2 Filter Mode", "Series 2 Mask", "Series 2 Comparator", "Serial Number", "Form Factor", "Series", "Transceiver Type", "Interface Number", "Series 2 Error/Arb Capture", "Transceiver Mode", "Transceiver External Outputs", "Transceiver External Inputs", "Start Trigger Behavior", "Log Comm Warnings", "User RTSI Frame", "Transmit Mode", "Log Start Trigger?", "Timestamp Format", "Master Timebase Rate", "Virtual Bus Timing", "Write Entries Free", "Timeline Recovery", "Log Bus Errors", "Log Transceiver Faults", "Termination", "LIN Sleep", "LIN Checksum Type", "LIN Response Timeout", "LIN Enable DLC Check", "LIN Log Wakeup", "Baud Rate"] ("AttrId")
          # "Read CAN-USB Data"
          n43 = case shown="True" w114 {
            tunnel: w116 -> [_ w127]
            tunnel: w123 -> [w126 w140]
            tunnel: w122 -> [_ w128]
            tunnel: [u8[] [] ("Data") w130] -> w121
            tunnel: [w126 w129] -> w115
            frame False {
            }
            frame True {
              n44 = call <vilib>:"ncGetAttr.vi"("Error in"=w140, "AttrId"=w127, "ObjHandle in"=w128) -> ("Error out"=w139:errorcluster, "ObjHandle out"=w141:T7)  [unwired: 1 out]
              n45 = call <vilib>:"ncReadNet.vi"("ObjHandle in"=w141, "Error in"=w139) -> ("ArbitrationId"=w132:u32, "Data"=w138:u8[], "Error out"=w129:errorcluster)  [unwired: 2 in, 4 out]
              n46 = To Unsigned Word Integer(number=w132) -> (unsigned 16bit integer=w131:u16)
              n47 = Split Number(x=w131) -> (hi(x)=w134:u8, lo(x)=w133:u8)
              n48 = Insert Into Array(array=w138, index=0, new element=w134) -> (w136:u8[])
              n49 = Insert Into Array(array=w136, index=1, new element=w133) -> (w130:u8[])
            }
          }
          "CAN0 Error" <- w115
          n50 = case shown="True" w113 {
            tunnel: w124 -> [_ w157]
            tunnel: w116 -> [_ w156]
            tunnel: [u8[] [] ("Data") w146] -> w120
            tunnel: [w143 w145] -> w118
            tunnel: w117 -> [w143 w144]
            frame False {
            }
            frame True {
              n51 = call <vilib>:"ncGetAttr.vi"("Error in"=w144, "AttrId"=w156, "ObjHandle in"=w157) -> ("Error out"=w155:errorcluster, "ObjHandle out"=w158:T7)  [unwired: 1 out]
              n52 = call <vilib>:"ncReadNet.vi"("ObjHandle in"=w158, "Error in"=w155) -> ("ArbitrationId"=w154:u32, "Data"=w150:u8[], "Error out"=w145:errorcluster)  [unwired: 2 in, 4 out]
              n53 = To Unsigned Word Integer(number=w154) -> (unsigned 16bit integer=w153:u16)
              n54 = Split Number(x=w153) -> (hi(x)=w149:u8, lo(x)=w147:u8)
              n55 = Insert Into Array(array=w150, index=0, new element=w149) -> (w148:u8[])
              n56 = Insert Into Array(array=w148, index=1, new element=w147) -> (w146:u8[])
            }
          }
          "CAN1 Error" <- w118
          n57 = Build Array(w121, w120) -> (w119:u8[][])
        }
        frame 2 {
          n58 = case shown="False" w159 {
            tunnel: [w174 u8[][] []] -> w160
            frame False {
              n59 = local read "Data Path"() -> (w180:path)
              n60 = Wait Until Next ms Multiple(millisecond multiple="Timestep") -> ()  [unwired: 1 out]
              n61 = call-poly <vilib>:"Read From Spreadsheet File.vi"("delimiter (\\t)"=";" ("delimiter (\\t)"), "start of read offset (chars.:0)"="Progress", "number of rows (all:-1)"="Rows to read", "file path (dialog if empty)"=w180) -> ("mark after read (chars.)"=w171:i32, "all rows"=w178:string[][])  [unwired: 3 in, 3 out]
              n62 = case shown="True" "Play" {
                tunnel: w171 -> [_ w181]
                frame False {
                }
                frame True {
                  n63 = local write "Progress"(w181) -> ()
                }
              }
              n64 = Delete From Array(array=w178, index (col)=0 ("disabled index (col)")) -> (deleted portion=w165:string[], array with subset deleted=w176:string[][])  [unwired: 2 in]
              n65 = Array Size(array=w165) -> (size(s)=w167:i32)
              n66 = Decrement(x=w167) -> (x-1=w166:i32)
              n67 = Decimal String To Number(string=w176, default (0L)=u8 0 ("default (0 I32)")) -> (number=w174:u8[][])  [unwired: 1 in, 1 out]
              n68 = Index Array(array=w165, index=1) -> (element=w164:string)
              n69 = Index Array(array=w165, index=w166) -> (element=w162:string)
              n70 = Concatenate Strings(w164, "\r\n", w162) -> (→"Time Stamp":string)
            }
            frame True {
            }
          }
        }
      }
      n71 = Empty Array?(array=w81) -> (empty?=w75:bool)
      n72 = feedback-in #1(w75) -> ()
      n73 = feedback #1(TRUE ("empty?")) -> (w77:bool)
      n74 = Not(x=w77) -> (.not. x?=w79:bool)
      n75 = for {
        tunnel: w81 -> [w206] mode=indexing
        tunnel: [w207] -> w90 mode=indexing
        shift-right: [w197] -> w99
        shift-left: w100 -> [w205]
        shift-right: [w203] -> w98
        shift-left: w97 -> [w204]
        shift-right: [w201] -> w93
        shift-left: w94 -> [w202]
        shift-right: [w196] -> w92
        shift-left: w95 -> [w200]
        shift-right: [w198] -> w91
        shift-left: w96 -> [w199]
        # "CAN ID"
        n76 = Index Array(array=w206, index=0) -> (element=w209:u8)
        n77 = Index Array(array=w206, index=1) -> (element=w208:u8)
        n78 = Join Numbers(hi=w209, lo=w208) -> ((hi.lo)=w207:u16)
        n79 = case shown="212" w207 {
          tunnel: w206 -> [_ w250 w304 w353 w374 w401 w432 w463 w508 w537 w658 w667 w777 w847 w877 w947 w1027 w1079 w1165 w1193 w1245 w1279 w1324 w1352 w1371 w1452 w1526 w1554 w1611 w1618 w1639 w1715 w1765 w1800 w1883 w1963 w2029 w2065 w2089 w2107 w2131 w2191 w2241 w2255 w2301 w2317 w2334 w2364 w2520 w2538 w2643 w2751 w2849 w2873]
          tunnel: w205 -> [w216 w257 w311 w360 w389 w420 w451 w482 w515 w544 w665 w694 w809 w864 w891 w951 w1042 w1123 w1184 w1234 w1274 w1310 w1338 w1366 w1402 w1483 w1540 w1568 w1610 w1627 w1677 w1746 w1789 w1854 w1899 w2009 w2059 w2082 w2090 w2108 w2132 w2198 w2250 w2274 w2314 w2326 w2335 w2411 w2529 w2623 w2699 w2836 w2855 w2890]
          tunnel: [w216 w257 w311 w360 w389 w420 w451 w482 w515 w544 w665 w694 w809 w864 w891 w921 w1042 w1123 w1184 w1234 w1274 w1310 w1338 w1366 w1402 w1483 w1540 w1568 w1610 w1627 w1677 w1746 w1789 w1854 w1899 w2009 w2059 w2082 w2090 w2108 w2132 w2198 w2250 w2274 w2314 w2326 w2335 w2411 w2529 w2623 w2699 w2836 w2855 w2890] -> w197
          tunnel: w204 -> [w215 w256 w310 w359 w388 w419 w450 w481 w514 w543 w664 w693 w808 w863 w890 w944 w1041 w1122 w1188 w1238 w1273 w1309 w1337 w1365 w1401 w1482 w1539 w1567 w1609 w1631 w1676 w1750 w1793 w1857 w1898 w2008 w2055 w2086 w2102 w2112 w2136 w2202 w2254 w2267 w2313 w2330 w2339 w2415 w2533 w2627 w2702 w2840 w2854 w2889]
          tunnel: [w215 w256 w310 w359 w388 w419 w450 w481 w514 w543 w664 w693 w808 w863 w890 w897 w1041 w1122 w1188 w1238 w1273 w1309 w1337 w1365 w1401 w1482 w1539 w1567 w1609 w1631 w1676 w1750 w1793 w1857 w1898 w2008 w2055 w2086 w2102 w2112 w2136 w2202 w2254 w2267 w2313 w2330 w2339 w2415 w2533 w2627 w2702 w2840 w2854 w2889] -> w203
          tunnel: w202 -> [w214 w255 w309 w358 w387 w418 w449 w478 w513 w542 w663 w690 w807 w862 w889 w931 w1038 w1117 w1187 w1237 w1270 w1306 w1334 w1362 w1398 w1479 w1536 w1564 w1579 w1630 w1669 w1749 w1792 w1856 w1897 w2007 w2058 w2085 w2101 w2111 w2135 w2201 w2253 w2275 w2311 w2329 w2338 w2414 w2532 w2626 w2628 w2839 w2852 w2886]
          tunnel: [w214 w255 w309 w358 w387 w418 w449 w478 w513 w542 w663 w690 w807 w862 w889 w931 w1038 w1117 w1187 w1237 w1270 w1306 w1334 w1362 w1398 w1479 w1536 w1564 w1579 w1630 w1669 w1749 w1792 w1856 w1897 w2007 w2058 w2085 w2101 w2111 w2135 w2201 w2253 w2257 w2311 w2329 w2338 w2414 w2532 w2626 w2628 w2839 w2852 w2886] -> w201
          tunnel: w200 -> [w213 w254 w308 w357 w386 w417 w448 w477 w512 w541 w662 w691 w806 w861 w888 w929 w1039 w1116 w1186 w1236 w1271 w1307 w1335 w1363 w1399 w1480 w1537 w1565 w1578 w1629 w1668 w1748 w1791 w1855 w1896 w2006 w2057 w2084 w2100 w2110 w2134 w2200 w2252 w2271 w2310 w2328 w2337 w2413 w2531 w2625 w2701 w2838 w2851 w2887]
          tunnel: w199 -> [w212 w253 w307 w356 w385 w416 w447 w476 w511 w540 w661 w692 w805 w860 w887 w930 w1040 w1121 w1185 w1235 w1272 w1308 w1336 w1364 w1400 w1481 w1538 w1566 w1608 w1628 w1675 w1747 w1790 w1853 w1895 w2005 w2056 w2083 w2099 w2109 w2133 w2199 w2251 w2268 w2312 w2327 w2336 w2412 w2530 w2624 w2700 w2837 w2853 w2888]
          tunnel: [w212 w253 w307 w356 w385 w416 w447 w476 w511 w540 w661 w692 w805 w860 w887 w930 w1040 w1121 w1185 w1235 w1272 w1308 w1336 w1364 w1400 w1481 w1538 w1566 w1608 w1628 w1675 w1747 w1790 w1853 w1895 w2005 w2056 w2083 w2099 w2109 w2133 w2199 w2251 w2263 w2312 w2327 w2336 w2412 w2530 w2624 w2700 w2837 w2853 w2888] -> w198
          tunnel: [w213 w254 w308 w357 w386 w417 w448 w477 w512 w541 w662 w691 w806 w861 w888 w929 w1039 w1116 w1186 w1236 w1271 w1307 w1335 w1363 w1399 w1480 w1537 w1565 w1578 w1629 w1668 w1748 w1791 w1855 w1896 w2006 w2057 w2084 w2100 w2110 w2134 w2200 w2252 w2269 w2310 w2328 w2337 w2413 w2531 w2625 w2701 w2838 w2851 w2887] -> w196
          frame 0, Default {
          }
          frame 372 {
            w245 = i16 -32768
            # "Acceleration Y & Yaw"
            n80 = Index Array(array=w250, index=7) -> (element=w249:u8)
            n81 = Index Array(array=w250, index=6) -> (element=w246:u8)
            n82 = Index Array(array=w250, index=3) -> (element=w248:u8)
            n83 = Index Array(array=w250, index=2) -> (element=w247:u8)
            n84 = Join Numbers(hi=w248, lo=w247) -> ((hi.lo)=w241:u16)
            n85 = Join Numbers(hi=w249, lo=w246) -> ((hi.lo)=w243:u16)
            n86 = To Word Integer(number=w241) -> (16bit integer=w242:i16)
            n87 = To Word Integer(number=w243) -> (16bit integer=w244:i16)
            n88 = Subtract(x=w244, y=w245) -> (x-y=w240:i16)
            n89 = Subtract(x=w242, y=w245) -> (x-y=w239:i16)
            n90 = local read "Actual Velocity\nFL [RPM]"() -> (w222:i16)
            n91 = local read "Actual Velocity \nRR [RPM]"() -> (w226:i16)
            n92 = local read "Actual Velocity\nFR [RPM]"() -> (w225:i16)
            n93 = To Double Precision Float(number=w240) -> (double precision float=w238:dbl)
            n94 = To Double Precision Float(number=w239) -> (double precision float=w237:dbl)
            n95 = local read "Actual Velocity\nRL [RPM]"() -> (w227:i16)
            n96 = Multiply(x=w237, y=0.005) -> (x*y=→"Yaw" →"Yaw Rear":dbl)
            n97 = Multiply(x=w238, y=0.0001274) -> (x*y=→"Acc Y":dbl)
            n98 = Build Array(w222, w225, w226, w227) -> (w228:i16[])
            n99 = To Double Precision Float(number=w222) -> (double precision float=w223:dbl)
            n100 = Array Max & Min(array=w228) -> (min value=w224:i16)  [unwired: 3 out]
            n101 = local read "IsStopped"() -> (w233:bool)
            n102 = To Double Precision Float(number=w224) -> (double precision float=w220:dbl)
            n103 = case shown="True" w233 {
              frame False {
              }
              frame True {
                n104 = local read "OffsetFilter"() -> (w260:dbl)
                n105 = local read "Acc Y"() -> (w263:dbl)
                n106 = feedback #2() -> (w262:dbl)  [unwired: 1 in]
                n107 = formula code="y_=a*x+(1-a)*y;"("x"=w263, "y"=w262, "a"=w260) -> ("y_"=w261:dbl)
                n108 = feedback-in #2(w261) -> ()
                n109 = local write "Acc Y offset"(w261) -> ()
              }
            }
            n110 = Divide(x=w220, y=677.4732) -> ()  [unwired: 1 out]
            n111 = Divide(x=w223, y=148.96908) -> (x/y=w218:dbl)
            n112 = Multiply(x=w218, y=0.227) -> (x*y=w217:dbl)
            n113 = Subtract(x=w217, y=w220) -> (x-y=w219:dbl)
            n114 = Divide(x=w219, y=w217) -> (x/y=→"Slip":dbl)
          }
          frame 376 {
            w299 = i16 -32768
            # "Acceleration X & Roll"
            n115 = Index Array(array=w304, index=7) -> (element=w303:u8)
            n116 = Index Array(array=w304, index=6) -> (element=w300:u8)
            n117 = Index Array(array=w304, index=3) -> (element=w302:u8)
            n118 = Index Array(array=w304, index=2) -> (element=w301:u8)
            n119 = Join Numbers(hi=w302, lo=w301) -> ((hi.lo)=w295:u16)
            n120 = Join Numbers(hi=w303, lo=w300) -> ((hi.lo)=w297:u16)
            n121 = To Word Integer(number=w295) -> (16bit integer=w296:i16)
            n122 = To Word Integer(number=w297) -> (16bit integer=w298:i16)
            n123 = Subtract(x=w298, y=w299) -> (x-y=w294:i16)
            n124 = Subtract(x=w296, y=w299) -> (x-y=w293:i16)
            n125 = To Double Precision Float(number=w294) -> (double precision float=w292:dbl)
            n126 = To Double Precision Float(number=w293) -> (double precision float=w291:dbl)
            n127 = local read "Acc Y"() -> (w268:dbl)
            n128 = local read "Acc Z"() -> (w272:dbl)
            n129 = Multiply(x=w291, y=0.005) -> (x*y=→"Roll":dbl)
            n130 = Multiply(x=w292, y=0.0001274) -> (x*y=→"Acc X":dbl)
            n131 = feedback #3() -> (w273:dbl)  [unwired: 1 in]
            n132 = formula code="y_=a*x+(1-a)*y;"("x"=w272, "y"=w273, "a"=0.02 ("input variable")) -> ("y_"=w266:dbl)
            "accZ" <- w266
            n133 = feedback-in #3(w266) -> ()
            n134 = feedback #4() -> (w270:dbl)  [unwired: 1 in]
            n135 = formula code="y_=a*x+(1-a)*y;"("x"=w268, "y"=w270, "a"=0.02 ("input variable")) -> ("y_"=w267:dbl)
            "accY" <- w267
            n136 = feedback-in #4(w267) -> ()
            n137 = feedback #5() -> (w287:dbl[])  [unwired: 1 in]
            n138 = Build Array (concatenate)(w287, w267) -> (w285:dbl[])
            n139 = feedback #6() -> (w280:dbl[])  [unwired: 1 in]
            n140 = Build Array (concatenate)(w280, w266) -> (w281:dbl[])
            n141 = Array Size(array=w285) -> (size(s)=w284:i32)
            n142 = Build Array(w267) -> (w278:dbl[])
            n143 = Build Array(w266) -> (w277:dbl[])
            n144 = Less?(x=w284, y=1000) -> (x < y?=w282:bool)
            n145 = case shown="False" w282 {
              tunnel: [w318 w327] -> w279
              tunnel: w281 -> [w319 w327]
              tunnel: [w322 w326] -> w286
              tunnel: w285 -> [w325 w326]
              frame False {
                n146 = Delete From Array(array=w325, length=1, index=0) -> (array with subset deleted=w322:dbl[])  [unwired: 1 out]
                n147 = Delete From Array(array=w319, length=1, index=0) -> (array with subset deleted=w318:dbl[])  [unwired: 1 out]
              }
              frame True {
              }
            }
            n148 = feedback-in #5(w286) -> ()
            n149 = feedback-in #6(w279) -> ()
            n150 = Bundle(w286, w279) -> (w275:cluster{dbl[], dbl[]})  [unwired: 1 in]
            n151 = Bundle(w278, w277) -> (w274:cluster{dbl[], dbl[]})  [unwired: 1 in]
            n152 = Build Array(w274, w275) -> (→"XY Graph":cluster{dbl[], dbl[]}[])
            n153 = local read "IsStopped"() -> (w265:bool)
            n154 = case shown="True" w265 {
              frame False {
              }
              frame True {
                n155 = local read "OffsetFilter"() -> (w314:dbl)
                n156 = local read "Roll"() -> (w317:dbl)
                n157 = feedback #7() -> (w316:dbl)  [unwired: 1 in]
                n158 = formula code="y_=a*x+(1-a)*y;"("x"=w317, "y"=w316, "a"=w314) -> ("y_"=w315:dbl)
                n159 = feedback-in #7(w315) -> ()
                n160 = local write "Rollrate offset"(w315) -> ()
              }
            }
          }
          frame 380 {
            w332 = u16 200 ("y")
            # "Acceleration Z"
            n161 = Index Array(array=w353, index=7) -> (element=w352:u8)
            n162 = Index Array(array=w353, index=6) -> (element=w351:u8)
            n163 = Join Numbers(hi=w352, lo=w351) -> ((hi.lo)=w348:u16)
            n164 = local read "Velocity [km/h]"() -> (w340:dbl)
            n165 = To Word Integer(number=w348) -> (16bit integer=w349:i16)
            n166 = Subtract(x=w349, y=i16 -32768) -> (x-y=w347:i16)
            n167 = local read "AccelXRaw"() -> (w337:dbl)
            n168 = local read "IsStopped"() -> (w338:bool)
            n169 = To Double Precision Float(number=w347) -> (double precision float=w346:dbl)
            n170 = Divide(x=w340, y=3.6) -> (x/y=w328:dbl)
            n171 = Multiply(x=w346, y=0.0001274) -> (x*y=→"Acc Z":dbl)
            n172 = local read "BrakeRaw"() -> (w333:u16)
            n173 = local read "TorqRaw"() -> (w334:u16)
            n174 = case shown="True" w338 {
              frame False {
              }
              frame True {
                n175 = local read "OffsetFilter"() -> (w363:dbl)
                n176 = local read "Acc Z"() -> (w366:dbl)
                n177 = feedback #8() -> (w365:dbl)  [unwired: 1 in]
                n178 = formula code="y_=a*x+(1-a)*y;"("x"=w366, "y"=w365, "a"=w363) -> ("y_"=w364:dbl)
                n179 = feedback-in #8(w364) -> ()
                n180 = local write "Acc Z offset"(w364) -> ()
              }
            }
            n181 = Less?(x=w334, y=w332) -> (x < y?=w330:bool)
            n182 = Less?(x=w333, y=w332) -> (x < y?=w331:bool)
            n183 = Multiply(x=0.01, y=w337) -> (x*y=w343:dbl)
            n184 = And(x=w330, y=w331) -> (x .and. y?=w329:bool)
            n185 = feedback #9(w328) -> (w344:dbl)
            n186 = Add(x=w344, y=w343) -> (x+y=w336:dbl)
            n187 = case shown="False" w329 {
              tunnel: w336 -> [w361 _]
              tunnel: [w361 w362] -> w335
              tunnel: w328 -> [_ w362]
              frame False {
              }
              frame True {
              }
            }
            "Vel_acc" <- w335
            n188 = feedback-in #9(w335) -> ()
          }
          frame 389 {
            # "TCU FL"
            n189 = Index Array(array=w374, index=7) -> (element=w395:u8)
            n190 = Index Array(array=w374, index=6) -> (element=w394:u8)
            n191 = Index Array(array=w374, index=9) -> (element=w391:u8)
            n192 = Index Array(array=w374, index=8) -> (element=w390:u8)
            n193 = Index Array(array=w374, index=3) -> (element=w379:u8)
            n194 = Number To Boolean Array(number=w379) -> (Boolean array=→"TCU FL Status":bool[])
            n195 = Join Numbers(hi=w395, lo=w394) -> ((hi.lo)=w381:u16)
            n196 = Join Numbers(hi=w391, lo=w390) -> ((hi.lo)=w383:u16)
            n197 = Index Array(array=w374, index=5) -> (element=w373:u8)
            n198 = Index Array(array=w374, index=4) -> (element=w372:u8)
            n199 = Join Numbers(hi=w373, lo=w372) -> ((hi.lo)=w371:u16)
            n200 = To Word Integer(number=w371) -> (16bit integer=w370:i16)
            n201 = To Word Integer(number=w381) -> (16bit integer=w384:i16)
            n202 = To Word Integer(number=w383) -> (16bit integer=w382:i16)
            n203 = To Double Precision Float(number=w370) -> (double precision float=→"FL Velocity":dbl)
            n204 = To Double Precision Float(number=w384) -> (double precision float=w368:dbl)
            "FL" <- w368
            "FL Torque Pos" <- w368
            n205 = To Double Precision Float(number=w382) -> (double precision float=w367:dbl)
            "FL 2" <- w367
            "FL Torque Neg" <- w367
            n206 = Add(x=w368, y=w367) -> (x+y=→"TCU FL":dbl)
          }
          frame 390 {
            # "TCU FR"
            n207 = Index Array(array=w401, index=7) -> (element=w426:u8)
            n208 = Index Array(array=w401, index=6) -> (element=w425:u8)
            n209 = Index Array(array=w401, index=9) -> (element=w422:u8)
            n210 = Index Array(array=w401, index=8) -> (element=w421:u8)
            n211 = Index Array(array=w401, index=3) -> (element=w410:u8)
            n212 = Number To Boolean Array(number=w410) -> (Boolean array=→"TCU FR Status":bool[])
            n213 = Index Array(array=w401, index=5) -> (element=w405:u8)
            n214 = Index Array(array=w401, index=4) -> (element=w404:u8)
            n215 = Join Numbers(hi=w426, lo=w425) -> ((hi.lo)=w414:u16)
            n216 = Join Numbers(hi=w422, lo=w421) -> ((hi.lo)=w412:u16)
            n217 = Join Numbers(hi=w405, lo=w404) -> ((hi.lo)=w403:u16)
            n218 = To Word Integer(number=w403) -> (16bit integer=w402:i16)
            n219 = To Word Integer(number=w414) -> (16bit integer=w415:i16)
            n220 = To Word Integer(number=w412) -> (16bit integer=w413:i16)
            n221 = To Double Precision Float(number=w402) -> (double precision float=→"FR Velocity":dbl)
            n222 = To Double Precision Float(number=w415) -> (double precision float=w399:dbl)
            "FR" <- w399
            "FR Torque Pos" <- w399
            n223 = To Double Precision Float(number=w413) -> (double precision float=w398:dbl)
            "FR 2" <- w398
            "FR Torque Neg" <- w398
            n224 = Add(x=w399, y=w398) -> (x+y=→"TCU FR":dbl)
          }
          frame 393 {
            # "TCU RL"
            n225 = Index Array(array=w432, index=7) -> (element=w457:u8)
            n226 = Index Array(array=w432, index=6) -> (element=w456:u8)
            n227 = Index Array(array=w432, index=9) -> (element=w453:u8)
            n228 = Index Array(array=w432, index=8) -> (element=w452:u8)
            n229 = Index Array(array=w432, index=3) -> (element=w441:u8)
            n230 = Index Array(array=w432, index=5) -> (element=w436:u8)
            n231 = Index Array(array=w432, index=4) -> (element=w435:u8)
            n232 = Number To Boolean Array(number=w441) -> (Boolean array=→"TCU RL Status":bool[])
            n233 = Join Numbers(hi=w457, lo=w456) -> ((hi.lo)=w444:u16)
            n234 = Join Numbers(hi=w453, lo=w452) -> ((hi.lo)=w443:u16)
            n235 = Join Numbers(hi=w436, lo=w435) -> ((hi.lo)=w434:u16)
            n236 = To Word Integer(number=w434) -> (16bit integer=w433:i16)
            n237 = To Word Integer(number=w444) -> (16bit integer=w446:i16)
            n238 = To Word Integer(number=w443) -> (16bit integer=w445:i16)
            n239 = To Double Precision Float(number=w433) -> (double precision float=→"RL Velocity":dbl)
            n240 = To Double Precision Float(number=w446) -> (double precision float=w430:dbl)
            "RL" <- w430
            "RL Torque Pos" <- w430
            n241 = To Double Precision Float(number=w445) -> (double precision float=w429:dbl)
            "RL 2" <- w429
            "RL Torque Neg" <- w429
            n242 = Add(x=w430, y=w429) -> (x+y=→"TCU RL":dbl)
          }
          frame 394 {
            # "TCU RR"
            n243 = Index Array(array=w463, index=7) -> (element=w488:u8)
            n244 = Index Array(array=w463, index=6) -> (element=w487:u8)
            n245 = Index Array(array=w463, index=9) -> (element=w484:u8)
            n246 = Index Array(array=w463, index=8) -> (element=w483:u8)
            n247 = Index Array(array=w463, index=3) -> (element=w472:u8)
            n248 = Index Array(array=w463, index=5) -> (element=w467:u8)
            n249 = Index Array(array=w463, index=4) -> (element=w466:u8)
            n250 = Number To Boolean Array(number=w472) -> (Boolean array=→"TCU RR Status":bool[])
            n251 = Join Numbers(hi=w488, lo=w487) -> ((hi.lo)=w474:u16)
            n252 = Join Numbers(hi=w484, lo=w483) -> ((hi.lo)=w480:u16)
            n253 = Join Numbers(hi=w467, lo=w466) -> ((hi.lo)=w465:u16)
            n254 = To Word Integer(number=w465) -> (16bit integer=w464:i16)
            n255 = To Double Precision Float(number=w464) -> (double precision float=→"RR Velocity":dbl)
            n256 = To Word Integer(number=w474) -> (16bit integer=w475:i16)
            n257 = To Word Integer(number=w480) -> (16bit integer=w479:i16)
            n258 = To Double Precision Float(number=w475) -> (double precision float=w461:dbl)
            "RR" <- w461
            "RR Torque Pos" <- w461
            n259 = To Double Precision Float(number=w479) -> (double precision float=w460:dbl)
            "RR 2" <- w460
            "RR Torque Neg" <- w460
            n260 = Add(x=w461, y=w460) -> (x+y=→"TCU RR":dbl)
          }
          frame 436 {
            w503 = i16 -32768
            # "Acceleration Y & Yaw"
            n261 = Index Array(array=w508, index=7) -> (element=w507:u8)
            n262 = Index Array(array=w508, index=6) -> (element=w504:u8)
            n263 = Index Array(array=w508, index=3) -> (element=w506:u8)
            n264 = Index Array(array=w508, index=2) -> (element=w505:u8)
            n265 = Join Numbers(hi=w506, lo=w505) -> ((hi.lo)=w499:u16)
            n266 = Join Numbers(hi=w507, lo=w504) -> ((hi.lo)=w501:u16)
            n267 = To Word Integer(number=w499) -> (16bit integer=w500:i16)
            n268 = To Word Integer(number=w501) -> (16bit integer=w502:i16)
            n269 = Subtract(x=w502, y=w503) -> (x-y=w498:i16)
            n270 = Subtract(x=w500, y=w503) -> (x-y=w497:i16)
            n271 = To Double Precision Float(number=w498) -> (double precision float=w496:dbl)
            n272 = To Double Precision Float(number=w497) -> (double precision float=w495:dbl)
            n273 = Multiply(x=w495, y=0.005) -> (x*y=→"Yaw 2" →"Yaw Front":dbl)
            n274 = Multiply(x=w496, y=0.0001274) -> (x*y=→"Acc Y 2":dbl)
          }
          frame 440 {
            w532 = i16 -32768
            # "Acceleration X & Roll"
            n275 = local read "Data Source"() -> (w519:u16)
            n276 = Index Array(array=w537, index=7) -> (element=w536:u8)
            n277 = Index Array(array=w537, index=6) -> (element=w533:u8)
            n278 = Index Array(array=w537, index=3) -> (element=w535:u8)
            n279 = Index Array(array=w537, index=2) -> (element=w534:u8)
            n280 = Join Numbers(hi=w535, lo=w534) -> ((hi.lo)=w528:u16)
            n281 = Join Numbers(hi=w536, lo=w533) -> ((hi.lo)=w530:u16)
            n282 = case shown="2" w519 {
              frame 0, Default {
              }
              frame 2 {
                (unwired) cluster{dbl, u32}[] [{-1.5, 255}, {0.0, 61192}, {1.5, 16711680}] ("Z Scale.Marker Values[]")
                w550 = 500 ("dimension size")
                n283 = local read "Roll 2"() -> (w578:dbl)
                n284 = feedback #10() -> (w580:dbl)  [unwired: 1 in]
                n285 = formula code="y_=a*x+(1-a)*y;"("x"=w578, "y"=w580, "a"=0.5 ("input variable")) -> ("y_"=w577:dbl)
                n286 = feedback-in #10(w577) -> ()
                n287 = local read "Velocity [km/h]"() -> (w586:dbl)
                n288 = Subtract(x=w577, y="Rollrate offset") -> (x-y=w579:dbl)
                n289 = Divide(x=w579, y=180.0 ("Yaw")) -> (x/y=w585:dbl)
                n290 = Divide(x=w586, y=3.6) -> (x/y=w588:dbl)
                n291 = Multiply(x=3.141592653589793, y=w585) -> (x*y=w583:dbl)
                n292 = feedback #11() -> (w597:dbl)  [unwired: 1 in]
                n293 = feedback #12() -> (w599:dbl)  [unwired: 1 in]
                n294 = feedback #13() -> (w600:dbl)  [unwired: 1 in]
                n295 = formula code="ve=v*cos(phi);\nvn=v*sin(phi);\nse=sx+ve*ts;\nsn=sy+vn*ts;\nphi_=phi+yaw*ts;"("phi"=w597, "yaw"=w583, "ts"=0.01 ("input variable"), "sx"=w600, "sy"=w599, "v"=w588) -> ("se"=w595:dbl, "sn"=w592:dbl, "phi_"=w598:dbl)  [unwired: 4 out]
                n296 = feedback-in #11(w598) -> ()
                n297 = feedback-in #12(w592) -> ()
                n298 = feedback-in #13(w595) -> ()
                n299 = local read "Acc Z 2"() -> (w554:dbl)
                n300 = feedback #14(dbl[] []) -> (w555:dbl[])
                n301 = Build Array (concatenate)(w555, w554) -> (w547:dbl[])
                n302 = feedback-in #14(w547) -> ()
                n303 = feedback #15(dbl[] []) -> (w594:dbl[])
                n304 = Build Array (concatenate)(w594, w595) -> (w570:dbl[])
                n305 = feedback-in #15(w570) -> ()
                n306 = feedback #16(dbl[] []) -> (w593:dbl[])
                n307 = Build Array (concatenate)(w593, w592) -> (w569:dbl[])
                n308 = feedback-in #16(w569) -> ()
                n309 = Bundle(w570, w569) -> (→"XY Graph 2":cluster{dbl[], dbl[]})  [unwired: 1 in]
                n310 = feedback #17() -> (w559:dbl)  [unwired: 1 in]
                n311 = feedback #18(0.0) -> (w572:dbl)
                n312 = Greater?(x=w572, y=200.0) -> (0:w576:bool)
                n313 = feedback #19() -> (w561:dbl)  [unwired: 1 in]
                n314 = feedback #20() -> (w563:dbl)  [unwired: 1 in]
                n315 = case shown="True" w576 {
                  tunnel: w570 -> [_ w644]
                  tunnel: w569 -> [_ w643]
                  tunnel: [w609 0.0] -> w574
                  tunnel: w572 -> [w610 _]
                  tunnel: [w608 w624] -> w564
                  tunnel: [w606 w623] -> w560
                  tunnel: [w607 w622] -> w562
                  tunnel: w563 -> [w608 _]
                  tunnel: w561 -> [w607 _]
                  tunnel: w559 -> [w606 _]
                  tunnel: w547 -> [_ w611]
                  frame False {
                    n316 = Increment(x=w610) -> (x+1=w609:dbl)
                  }
                  frame True {
                    n317 = Array Max & Min(array=w611) -> (max value=w621:dbl, min value=w620:dbl)  [unwired: 2 out]
                    n318 = Array Max & Min(array=w644) -> (max value=w638:dbl, min value=w639:dbl)  [unwired: 2 out]
                    n319 = Array Max & Min(array=w643) -> (max value=w630:dbl, min value=w629:dbl)  [unwired: 2 out]
                    n320 = Bundle(w620, u32 255) -> (w617:cluster{dbl, u32})  [unwired: 1 in]
                    n321 = Bundle("y"=0.0, u32 6618880) -> (w618:cluster{"y":dbl, u32})  [unwired: 1 in]
                    n322 = Bundle(w621, u32 16711680) -> (w619:cluster{dbl, u32})  [unwired: 1 in]
                    n323 = Add(x=w638, y=w639) -> (x+y=w637:dbl)
                    n324 = Subtract(x=w638, y=w639) -> (x-y=w642:dbl)
                    n325 = Subtract(x=w630, y=w629) -> (x-y=w641:dbl)
                    n326 = Add(x=w630, y=w629) -> (x+y=w631:dbl)
                    n327 = Build Array(w617, w618, w619) -> (w612:cluster{"y":dbl, u32}[])
                    n328 = Divide(x=w637, y=2.0) -> (x/y=w634:dbl)
                    n329 = Build Array(w642, w641) -> (w640:dbl[])
                    n330 = property on="Intensity Graph" class="IntGraph (strict)"("ZScale.MarkerVals[]"=w612) -> ()  [unwired: 2 in, 2 out]
                    n331 = Divide(x=w631, y=2.0) -> (x/y=w627:dbl)
                    n332 = Array Max & Min(array=w640) -> (max value=w622:dbl)  [unwired: 3 out]
                    n333 = Divide(x=w622, y=2.0) -> (x/y=w626:dbl)
                    n334 = Subtract(x=w634, y=w626) -> (x-y=w624:dbl)
                    n335 = Subtract(x=w627, y=w626) -> (x-y=w623:dbl)
                    n336 = Add(x=w634, y=w626) -> (x+y=w633:dbl)
                    n337 = Add(x=w627, y=w626) -> (x+y=w628:dbl)
                    n338 = property on="XY Graph 2" class="XYGraph (strict)"("XScale.Minimum"=w624) -> ()  [unwired: 2 in, 2 out]
                    n339 = property on="XY Graph 2" class="XYGraph (strict)"("XScale.Maximum"=w633) -> ()  [unwired: 2 in, 2 out]
                    n340 = property on="XY Graph 2" class="XYGraph (strict)"("YScale.Minimum"=w623) -> ()  [unwired: 2 in, 2 out]
                    n341 = property on="XY Graph 2" class="XYGraph (strict)"("YScale.Maximum"=w628) -> ()  [unwired: 2 in, 2 out]
                  }
                }
                n342 = feedback-in #17(w560) -> ()
                n343 = feedback-in #18(w574) -> ()
                n344 = feedback-in #19(w562) -> ()
                n345 = feedback-in #20(w564) -> ()
                n346 = Divide(x=w562, y=500.0) -> (x/y=w565:dbl)
                n347 = Subtract(x=w569, y=w560) -> (x-y=w567:dbl[])
                n348 = Subtract(x=w570, y=w564) -> (x-y=w568:dbl[])
                n349 = Divide(x=w568, y=w565) -> (x/y=w558:dbl[])
                n350 = Divide(x=w567, y=w565) -> (x/y=w557:dbl[])
                n351 = Round To Nearest(number=w558) -> (nearest integer value=w553:dbl[])
                n352 = Round To Nearest(number=w557) -> (nearest integer value=w552:dbl[])
                n353 = Initialize Array(-100.0 ("element"), w550, w550) -> (w549:dbl[][])
                n354 = for {
                  tunnel: w553 -> [w605] mode=indexing
                  tunnel: w552 -> [w604] mode=indexing
                  tunnel: w547 -> [w603] mode=indexing
                  shift-right: [w601] -> w548
                  shift-left: w549 -> [w602]
                  n355 = Replace Array Subset(array=w602, new element=w603, index (row)=w605, index (col)=w604) -> (w601:dbl[][])
                }
                "Intensity Graph" <- w548
              }
            }
            n356 = To Word Integer(number=w528) -> (16bit integer=w529:i16)
            n357 = To Word Integer(number=w530) -> (16bit integer=w531:i16)
            n358 = Subtract(x=w531, y=w532) -> (x-y=w527:i16)
            n359 = Subtract(x=w529, y=w532) -> (x-y=w526:i16)
            n360 = To Double Precision Float(number=w527) -> (double precision float=w525:dbl)
            n361 = To Double Precision Float(number=w526) -> (double precision float=w524:dbl)
            n362 = Multiply(x=w524, y=0.005) -> (x*y=→"Roll 2":dbl)
            n363 = Multiply(x=w525, y=0.0001274) -> (x*y=→"Acc X 2":dbl)
            n364 = local read "IsStopped"() -> (w520:bool)
            n365 = case shown="True" w520 {
              frame False {
              }
              frame True {
                n366 = local read "OffsetFilter"() -> (w645:dbl)
                n367 = local read "Acc X 2"() -> (w648:dbl)
                n368 = feedback #21() -> (w647:dbl)  [unwired: 1 in]
                n369 = formula code="y_=a*x+(1-a)*y;"("x"=w648, "y"=w647, "a"=w645) -> ("y_"=w646:dbl)
                n370 = feedback-in #21(w646) -> ()
                n371 = local write "Acc X offset 2"(w646) -> ()
              }
            }
          }
          frame 444 {
            # "Acceleration Z"
            n372 = Index Array(array=w658, index=7) -> (element=w657:u8)
            n373 = Index Array(array=w658, index=6) -> (element=w656:u8)
            n374 = Join Numbers(hi=w657, lo=w656) -> ((hi.lo)=w653:u16)
            n375 = To Word Integer(number=w653) -> (16bit integer=w654:i16)
            n376 = Subtract(x=w654, y=i16 -32768) -> (x-y=w652:i16)
            n377 = To Double Precision Float(number=w652) -> (double precision float=w651:dbl)
            n378 = Multiply(x=w651, y=0.0001274) -> (x*y=→"Acc Z 2":dbl)
          }
          frame 512 {
            # "Torque signal"
            # "Pedalbox Throttle Steering"
            n379 = Index Array(array=w667, index=2) -> (element=w680:u8)
            n380 = Index Array(array=w667, index=3) -> (element=w679:u8)
            n381 = local read "TCU Version"() -> (w686:u16)
            n382 = Index Array(array=w667, index=4) -> (element=w688:u8)
            n383 = Index Array(array=w667, index=5) -> (element=w687:u8)
            n384 = Join Numbers(hi=w688, lo=w687) -> ((hi.lo)=w689:u16)
            n385 = Subtract(x=w686, y=u16 2016) -> (x-y=w684:u16)
            n386 = Subtract(x=w689, y="Torque Min") -> (x-y=w700:dbl)
            n387 = Subtract(x="Torque Max", y="Torque Min") -> (x-y=w699:dbl)
            n388 = case shown="1" w684 {
              tunnel: w667 -> [w707 w730]
              tunnel: [i16 0 ("STA1") w725] -> _
              tunnel: [i16 0 ("STA1") w720] -> _
              tunnel: [w704 w721] -> _
              tunnel: [w703 i16 0 ("STA1")] -> w683
              frame 0, Default {
                # "TCU 2016"
                n389 = Index Array(array=w707, index=8) -> (element=w710:u8)
                n390 = Index Array(array=w707, index=9) -> (element=w711:u8)
                n391 = Join Numbers(hi=w710, lo=w711) -> ((hi.lo)=w703:u16)
                n392 = Subtract(x=w703, y="Steering Null") -> (x-y=w712:dbl)
                n393 = Subtract(x="Steering Max", y="Steering Min") -> (x-y=w717:dbl)
                n394 = Divide(x=w712, y=w717) -> (x/y=w713:dbl)
                n395 = Multiply(x=360.0, y=w713) -> (x*y=w704:dbl)
              }
              frame 1 {
                # "TCU 2017"
                n396 = Index Array(array=w730, index=6) -> (element=w736:u8)
                n397 = Index Array(array=w730, index=7) -> (element=w733:u8)
                n398 = Index Array(array=w730, index=8) -> (element=w729:u8)
                n399 = Index Array(array=w730, index=9) -> (element=w728:u8)
                n400 = And(x=w736, y=u8 127) -> (x .and. y?=w735:u8)
                n401 = Join Numbers(hi=w729, lo=w728) -> ((hi.lo)=w726:u16)
                n402 = Join Numbers(hi=w735, lo=w733) -> ((hi.lo)=w734:u16)
                n403 = Subtract(x=w734, y=i16 3600) -> (x-y=w725:u16)
                n404 = Subtract(x=w726, y=i16 3600) -> (x-y=w720:u16)
                n405 = To Word Integer(number=w720) -> (16bit integer=w723:i16)
                n406 = To Double Precision Float(number=w723) -> (double precision float=w722:dbl)
                n407 = Divide(x=w722, y=10.0) -> (x/y=w721:dbl)
              }
            }
            "SteeringRaw" <- w683
            n408 = formula code="out = (in1 << 8) | in2;"("in1"=w688, "in2"=w687) -> ("out"=→"TPS2_Raw":dbl)
            n409 = formula code="out = (in1 << 8) | in2;"("in1"=w680, "in2"=w679) -> ("out"=→"TorqRaw 2" →"TPS1_Raw":dbl)
            n410 = Divide(x=w700, y=w699) -> (x/y=w696:dbl)
            n411 = Index Array(array=w667, index=6) -> (element=w674:u8)
            n412 = Index Array(array=w667, index=7) -> (element=w673:u8)
            n413 = Index Array(array=w667, index=8) -> (element=w669:u8)
            n414 = Index Array(array=w667, index=9) -> (element=w668:u8)
            n415 = formula code="out = (in1 << 8) | in2;"("in1"=w674, "in2"=w673) -> ("out"=→"STA1":dbl)
            n416 = formula code="out = (in1 << 8) | in2;"("in1"=w669, "in2"=w668) -> ("out"=→"STA2":dbl)
            n417 = Multiply(x=100.0, y=w696) -> ()  [unwired: 1 out]
          }
          frame 513 {
            w782 = 18.6 ("y")
            # "Pedalbox Brake"
            n418 = Index Array(array=w777, index=2) -> (element=w772:u8)
            n419 = Index Array(array=w777, index=3) -> (element=w770:u8)
            n420 = And(x=w772, y=u8 15) -> (x .and. y?=w771:u8)
            n421 = Join Numbers(hi=w771, lo=w770) -> ((hi.lo)=→"BPS1_Raw":u16)
            n422 = Index Array(array=w777, index=4) -> (element=w776:u8)
            n423 = Index Array(array=w777, index=8) -> (element=w793:u8)
            n424 = Index Array(array=w777, index=6) -> (element=w803:u8)
            n425 = And(x=w776, y=u8 15) -> (x .and. y?=w775:u8)
            n426 = Index Array(array=w777, index=5) -> (element=w816:u8)
            n427 = Join Numbers(hi=w775, lo=w816) -> ((hi.lo)=w768:u16)
            "BPS2_Raw" <- w768
            n428 = Index Array(array=w777, index=9) -> (element=w786:u8)
            n429 = Index Array(array=w777, index=7) -> (element=w796:u8)
            n430 = And(x=w793, y=u8 15) -> (x .and. y?=w787:u8)
            n431 = And(x=w803, y=u8 15) -> (x .and. y?=w797:u8)
            n432 = Join Numbers(hi=w797, lo=w796) -> ((hi.lo)=w766:u16)
            "BPR_Raw" <- w766
            n433 = Join Numbers(hi=w787, lo=w786) -> ((hi.lo)=w765:u16)
            "BrakeRaw 2" <- w765
            "BPF_Raw" <- w765
            n434 = Subtract(x=w765, y="Brake Min 2") -> (x-y=w767:dbl)
            n435 = Subtract(x="Brake Max 2", y="Brake Min 2") -> (x-y=w791:dbl)
            n436 = Subtract(x=w766, y="Brake Min 2") -> (x-y=w781:dbl)
            n437 = Subtract(x="Brake Max 2", y="Brake Min 2") -> (x-y=w801:dbl)
            n438 = Subtract(x=w768, y="Brake Min") -> (x-y=w813:dbl)
            n439 = Subtract(x="Brake Max", y="Brake Min") -> (x-y=w812:dbl)
            n440 = Divide(x=w767, y=w791) -> (x/y=w790:dbl)
            n441 = Divide(x=w781, y=w801) -> (x/y=w800:dbl)
            n442 = Divide(x=w813, y=w812) -> (x/y=w811:dbl)
            n443 = feedback #22() -> (w749:dbl)  [unwired: 1 in]
            n444 = feedback #23() -> (w747:dbl)  [unwired: 1 in]
            n445 = Divide(x=w767, y=w782) -> (x/y=w742:dbl)
            n446 = formula code="y_=a*x+(1-a)*y;"("x"=w742, "y"=w749, "a"=0.02 ("input variable")) -> ("y_"=w744:dbl)
            "accZ 2" <- w744
            n447 = feedback-in #22(w744) -> ()
            n448 = Divide(x=w781, y=w782) -> (x/y=w743:dbl)
            n449 = formula code="y_=a*x+(1-a)*y;"("x"=w743, "y"=w747, "a"=0.02 ("input variable")) -> ("y_"=w745:dbl)
            n450 = feedback-in #23(w745) -> ()
            n451 = Multiply(x=100.0, y=w790) -> (x*y=→"Brake Rear":dbl)
            n452 = Multiply(x=100.0, y=w800) -> (x*y=→"Brake Front":dbl)
            n453 = Multiply(x=100.0, y=w811) -> ()  [unwired: 1 out]
            n454 = feedback #24() -> (w762:dbl[])  [unwired: 1 in]
            n455 = Build Array (concatenate)(w762, w745) -> (w760:dbl[])
            n456 = feedback #25() -> (w755:dbl[])  [unwired: 1 in]
            n457 = Build Array (concatenate)(w755, w744) -> (w756:dbl[])
            n458 = Build Array(w743) -> (w764:dbl[])
            n459 = Build Array(w742) -> (w763:dbl[])
            n460 = Bundle(w743, w742) -> (→"Brake Pressure":cluster{dbl, dbl})  [unwired: 1 in]
            n461 = Bundle(w764, w763) -> ()  [unwired: 1 in, 1 out]
            n462 = Array Size(array=w760) -> (size(s)=w759:i32)
            n463 = Build Array(w745) -> (w753:dbl[])
            n464 = Build Array(w744) -> (w752:dbl[])
            n465 = Less?(x=w759, y=1000) -> (x < y?=w757:bool)
            n466 = case shown="False" w757 {
              tunnel: [w819 w828] -> w754
              tunnel: w756 -> [w820 w828]
              tunnel: [w823 w827] -> w761
              tunnel: w760 -> [w826 w827]
              frame False {
                n467 = Delete From Array(array=w826, length=1, index=0) -> (array with subset deleted=w823:dbl[])  [unwired: 1 out]
                n468 = Delete From Array(array=w820, length=1, index=0) -> (array with subset deleted=w819:dbl[])  [unwired: 1 out]
              }
              frame True {
              }
            }
            n469 = feedback-in #24(w761) -> ()
            n470 = feedback-in #25(w754) -> ()
            n471 = Bundle(w761, w754) -> (w751:cluster{dbl[], dbl[]})  [unwired: 1 in]
            n472 = Bundle(w753, w752) -> (w750:cluster{dbl[], dbl[]})  [unwired: 1 in]
            n473 = Build Array(w750, w751) -> (→"XY Graph 3":cluster{dbl[], dbl[]}[])
          }
          frame 1026 {
            # "Pedalbox Brake"
            n474 = Index Array(array=w847, index=8) -> (element=w836:u8)
            n475 = Index Array(array=w847, index=9) -> (element=w856:u8)
            n476 = And(x=w836, y=u8 15) -> (x .and. y?=w835:u8)
            n477 = Index Array(array=w847, index=6) -> (element=w830:u8)
            n478 = Index Array(array=w847, index=7) -> (element=w853:u8)
            n479 = Index Array(array=w847, index=4) -> (element=w833:u8)
            n480 = Index Array(array=w847, index=5) -> (element=w850:u8)
            n481 = Index Array(array=w847, index=2) -> (element=w839:u8)
            n482 = Index Array(array=w847, index=3) -> (element=w857:u8)
            n483 = Join Numbers(hi=w835, lo=w856) -> ((hi.lo)=w844:u16)
            n484 = And(x=w833, y=u8 15) -> (x .and. y?=w832:u8)
            n485 = And(x=w839, y=u8 15) -> (x .and. y?=w838:u8)
            n486 = Join Numbers(hi=w838, lo=w857) -> ((hi.lo)=w846:u16)
            n487 = And(x=w830, y=u8 15) -> (x .and. y?=w829:u8)
            n488 = Join Numbers(hi=w832, lo=w850) -> ((hi.lo)=w845:u16)
            n489 = Join Numbers(hi=w829, lo=w853) -> ((hi.lo)=w841:u16)
            n490 = local read "BPS2_Raw"() -> (w842:u16)
            n491 = local read "BPS1_Raw"() -> (w843:u16)
            n492 = Bundle(w846, w845, "BPS1_Raw"=w843, "BPS2_Raw"=w842, w841, w844) -> ()  [unwired: 1 in, 1 out]
          }
          frame 1027 {
            # "Pedalbox Brake"
            n493 = Index Array(array=w877, index=6) -> (element=w875:u8)
            n494 = Index Array(array=w877, index=7) -> (element=w884:u8)
            n495 = Index Array(array=w877, index=4) -> (element=w872:u8)
            n496 = Index Array(array=w877, index=5) -> (element=w892:u8)
            n497 = Index Array(array=w877, index=8) -> (element=w869:u8)
            n498 = Index Array(array=w877, index=9) -> (element=w881:u8)
            n499 = Index Array(array=w877, index=2) -> (element=w866:u8)
            n500 = Index Array(array=w877, index=3) -> (element=w880:u8)
            n501 = And(x=w872, y=u8 15) -> (x .and. y?=w871:u8)
            n502 = And(x=w875, y=u8 15) -> (x .and. y?=w874:u8)
            n503 = And(x=w866, y=u8 15) -> (x .and. y?=w865:u8)
            n504 = Join Numbers(hi=w865, lo=w880) -> ()  [unwired: 1 out]
            n505 = And(x=w869, y=u8 15) -> (x .and. y?=w868:u8)
            n506 = Join Numbers(hi=w871, lo=w892) -> ()  [unwired: 1 out]
            n507 = Join Numbers(hi=w868, lo=w881) -> ()  [unwired: 1 out]
            n508 = Join Numbers(hi=w874, lo=w884) -> ()  [unwired: 1 out]
          }
          frame 528 {
            # "HV Cell Values"
            # "HV Accumulator"
            n509 = Index Array(array=w947, index=3) -> (element=w927:u8)
            n510 = Index Array(array=w947, index=5) -> (element=w946:u8)
            n511 = Index Array(array=w947, index=6) -> (element=w945:u8)
            n512 = Join Numbers(hi=w946, lo=w945) -> ((hi.lo)=w923:u16)
            n513 = Index Array(array=w947, index=4) -> (element=w953:u8)
            n514 = And(x=w927, y=u8 127) -> (x .and. y?=w925:u8)
            n515 = Join Numbers(hi=w925, lo=w953) -> ((hi.lo)=w952:u16)
            n516 = Index Array(array=w947, index=2) -> (element=w928:u8)
            n517 = Divide(x=w923, y=10.0) -> (x/y=w924:dbl)
            n518 = Replace Array Subset(array=w951, new element=w952, index=w928) -> (w921:u16[])
            n519 = Replace Array Subset(array=w944, new element=w924, index=w928) -> (w897:dbl[])
            n520 = Array Subset(array=w897, index=0, length=180) -> (w900:dbl[])
            n521 = call "Stack.vi"("Array"=w921) -> ("Min"=→"Cell Min" →"HV Cell Voltage":u16, "Max"=→"Cell Max":u16, "appended array"=w920:u16[], "appended array 2"=w917:u16[], "appended array 3"=w916:u16[], "appended array 4"=w915:u16[], "appended array 5"=w918:u16[], "appended array 6"=w919:u16[])  [unwired: 11 in]
            n522 = Array Max & Min(array=w900) -> (max value=w902:dbl, min value=w903:dbl)  [unwired: 2 out]
            "Temp Max" <- w902
            n523 = Array Subset(array=w897, index=56, length=28) -> (→"Temp 3":dbl[])
            n524 = Array Subset(array=w897, index=0, length=28) -> (→"Temp 1":dbl[])
            n525 = Array Subset(array=w897, index=28, length=28) -> (→"Temp 2":dbl[])
            n526 = Array Subset(array=w897, index=84, length=28) -> (→"Temp 4":dbl[])
            n527 = Array Subset(array=w897, index=112, length=28) -> (→"Temp 5":dbl[])
            n528 = Array Subset(array=w897, index=140, length=28) -> (→"Temp 6":dbl[])
            n529 = Bundle(w902, w903) -> (→"HV Cell Temperature":cluster{dbl, dbl})  [unwired: 1 in]
            n530 = for {
              tunnel: [w968] -> w950 mode=indexing
              tunnel: w920 -> [w967] mode=indexing
              tunnel: w917 -> [w965] mode=indexing
              tunnel: [w966] -> w913 mode=indexing
              tunnel: w916 -> [w964] mode=indexing
              tunnel: [w963] -> w912 mode=indexing
              tunnel: w915 -> [w962] mode=indexing
              tunnel: w918 -> [w961] mode=indexing
              tunnel: w919 -> [w960] mode=indexing
              tunnel: [w959] -> w911 mode=indexing
              tunnel: [w958] -> w910 mode=indexing
              tunnel: [w957] -> w909 mode=indexing
              n531 = Bundle(w960, w960) -> (w957:cluster{u16, u16})  [unwired: 1 in]
              n532 = Bundle(w967, w967) -> (w968:cluster{u16, u16})  [unwired: 1 in]
              n533 = Bundle(w965, w965) -> (w966:cluster{u16, u16})  [unwired: 1 in]
              n534 = Bundle(w964, w964) -> (w963:cluster{u16, u16})  [unwired: 1 in]
              n535 = Bundle(w962, w962) -> (w959:cluster{u16, u16})  [unwired: 1 in]
              n536 = Bundle(w961, w961) -> (w958:cluster{u16, u16})  [unwired: 1 in]
            }
            "Stack 1" <- w950
            "Stack 2" <- w913
            "Stack 3" <- w912
            "Stack 4" <- w911
            "Stack 5" <- w910
            "Stack 6" <- w909
          }
          frame 530 {
            # "HV Battery Status"
            # "HV Battery Status"
            n537 = Index Array(array=w1027, index=6) -> (element=w1009:u8)
            n538 = Index Array(array=w1027, index=7) -> (element=w1008:u8)
            n539 = Index Array(array=w1027, index=4) -> (element=w1035:u8)
            n540 = Index Array(array=w1027, index=5) -> (element=w1034:u8)
            n541 = Index Array(array=w1027, index=8) -> (element=w1029:u8)
            n542 = Index Array(array=w1027, index=9) -> (element=w1028:u8)
            n543 = Index Array(array=w1027, index=2) -> (element=w1044:u8)
            n544 = Index Array(array=w1027, index=3) -> (element=w1043:u8)
            n545 = local read "Actual Velocity \nRR [RPM]"() -> (w987:i16)
            n546 = local read "Actual Velocity\nFL [RPM]"() -> (w992:i16)
            n547 = local read "Actual Velocity\nFR [RPM]"() -> (w991:i16)
            n548 = local read "Actual Velocity\nRL [RPM]"() -> (w989:i16)
            n549 = To Unsigned Byte Integer(number=w1008) -> (unsigned 8bit integer=w1011:u8)
            n550 = To Unsigned Byte Integer(number=w1009) -> (unsigned 8bit integer=w1010:u8)
            n551 = Join Numbers(hi=w1010, lo=w1011) -> ((hi.lo)=w1007:u16)
            n552 = Join Numbers(hi=w1035, lo=w1034) -> ((hi.lo)=w1021:u16)
            n553 = Join Numbers(hi=w1029, lo=w1028) -> ((hi.lo)=w1016:u16)
            n554 = Join Numbers(hi=w1044, lo=w1043) -> ((hi.lo)=w1024:u16)
            n555 = local read "TCU RR"() -> (w986:dbl)
            n556 = local read "TCU FL"() -> (w993:dbl)
            n557 = local read "TCU FR"() -> (w990:dbl)
            n558 = local read "TCU RL"() -> (w988:dbl)
            n559 = To Word Integer(number=w1007) -> (16bit integer=w1006:i16)
            n560 = To Double Precision Float(number=w1006) -> (double precision float=w1019:dbl)
            n561 = To Double Precision Float(number=w1021) -> (double precision float=w1022:dbl)
            n562 = To Double Precision Float(number=w1016) -> (double precision float=w1017:dbl)
            n563 = To Double Precision Float(number=w1024) -> (double precision float=w1025:dbl)
            n564 = Multiply(x=w992, y=w993) -> (x*y=w997:dbl)
            n565 = Multiply(x=w991, y=w990) -> (x*y=w996:dbl)
            n566 = Multiply(x=w989, y=w988) -> (x*y=w995:dbl)
            n567 = Multiply(x=w987, y=w986) -> (x*y=w994:dbl)
            n568 = Compound Arithmetic op=ADD(w997, w996, w995, w994) -> (w985:dbl)
            n569 = Divide(x=w1019, y=10.0) -> (x/y=→"HV Current":dbl)
            n570 = Divide(x=w1022, y=10.0) -> (x/y=→"HV After":dbl)
            n571 = Divide(x=w1017, y=1.0) -> (x/y=→"SoC [mAh]":dbl)
            n572 = Divide(x=w1025, y=10.0) -> (x/y=→"HV Before":dbl)
            n573 = Compound Arithmetic op=MULTIPLY(w985, 0.10472 ("x"), 0.0098 ("y"), 0.001 ("value")) -> (w969:dbl)
            n574 = local read "HV Current"() -> (w1002:dbl)
            "Current" <- w1002
            n575 = local read "HV Before"() -> (w1003:dbl)
            n576 = local read "HV After"() -> (w1004:dbl)
            n577 = Bundle("HV Before"=w1003, "HV After"=w1004) -> (→"HV Voltage":cluster{"HV Before":dbl, "HV After":dbl})  [unwired: 1 in]
            n578 = Compound Arithmetic op=MULTIPLY(w1003, w1002, 0.001 ("value")) -> (w979:dbl)
            n579 = Bundle(w979, w969) -> (→"Electric Power":cluster{dbl, dbl})  [unwired: 1 in]
            n580 = Divide(x=w979, y=3.6) -> (x/y=w971:dbl)
            n581 = local read "Cell Max"() -> (w999:u16)
            n582 = local read "Cell Min"() -> (w998:u16)
            n583 = Multiply(x=0.005, y=w971) -> (x*y=w980:dbl)
            n584 = Bundle("Cell Max"=w999, "Cell Min"=w998) -> (→"HV Cell":cluster{"Cell Max":u16, "Cell Min":u16})  [unwired: 1 in]
            n585 = feedback #26() -> (w975:dbl)  [unwired: 1 in]
            n586 = Add(x=w975, y=w980) -> (x+y=w973:dbl)
            n587 = case shown="True" "New Lap" {
              tunnel: w973 -> [w1047 _]
              tunnel: [w1047 0.0] -> w972
              frame False {
              }
              frame True {
              }
            }
            n588 = feedback-in #26(w972) -> ()
            n589 = feedback #27() -> (w976:dbl[])  [unwired: 1 in]
            n590 = case shown="False" "New Lap" {
              tunnel: w973 -> [w1051 w1056]
              tunnel: [w1050 w1055] -> w977
              tunnel: w976 -> [w1049 w1054]
              frame False {
                n591 = Array Size(array=w1049) -> (size(s)=w1053:i32)
                n592 = Decrement(x=w1053) -> (x-1=w1052:i32)
                n593 = Replace Array Subset(array=w1049, new element=w1051, index=w1052) -> (w1050:dbl[])
              }
              frame True {
                n594 = Build Array (concatenate)(w1054, w1056) -> (w1055:dbl[])
              }
            }
            "Energy" <- w977
            n595 = feedback-in #27(w977) -> ()
          }
          frame 531 {
            # "ilyen nincs 18ban"
            # "ilyen nincs 18ban"
            # "ilyen nincs 18-ban"
            # "HV Accumulator Status"
            # "Accumulator Status"
            n596 = Index Array(array=w1079, index=6) -> (element=→"Place of Error":u8)
            n597 = Index Array(array=w1079, index=7) -> (element=w1095:u8)
            n598 = Index Array(array=w1079, index=8) -> (element=w1094:u8)
            n599 = Index Array(array=w1079, index=4) -> (element=w1105:u8)
            n600 = Join Numbers(hi=w1095, lo=w1094) -> ((hi.lo)=→"Value":u16)
            n601 = Number To Boolean Array(number=w1105) -> (Boolean array=w1104:bool[])
            n602 = Index Array(array=w1079, index=3) -> (element=w1115:u8)
            n603 = Index Array(array=w1079, index=5) -> (element=w1111:u8)
            n604 = Number To Boolean Array(number=w1115) -> (Boolean array=w1120:bool[])
            n605 = Number To Boolean Array(number=w1111) -> (Boolean array=w1110:bool[])
            n606 = Index Array(array=w1104, index #1=7 ("index"), index #2=6 ("index"), index #3=5 ("index"), index #4=4 ("index"), index #5=3 ("index"), index #6=2 ("index"), index #7=1 ("index"), index #8=0 ("index")) -> (element #1=→"12V State" →"Driver Protection" →"SC 12V":bool, element #2=w1063:bool, element #3=w1061:bool, element #4=→"AMS Relay" →"SC AMS" →"AMS Relay 2":bool, element #5=→"IMD Relay" →"SC IMD" →"IMD Relay":bool, element #6=w1058:bool)  [unwired: 2 out]
            n607 = Not(x=w1058) -> (.not. x?=→"BSPD Relay" →"SC BSPD" →"BSPD Relay":bool)
            n608 = Index Array(array=w1120, index #1=7 ("index"), index #2=6 ("index"), index #3=5 ("index"), index #4=4 ("index"), index #5=3 ("index"), index #6=2 ("index"), index #7=1 ("index"), index #8=0 ("index")) -> (element #1=→"AMS error":bool, element #2=→"IMD error":bool, element #3=→"HVDet" →"HVDet":bool, element #4=→"AIR+" →"SC AIR+" →"AIR+":bool, element #5=→"AIR-" →"SC AIR-" →"AIR-":bool, element #6=→"SC Endline":bool, element #7=w1059:bool, element #8=→"TSAL State" →"TSAL State 2":bool)
            n609 = Index Array(array=w1110, index #1=7 ("index"), index #2=6 ("index"), index #3=5 ("index"), index #4=4 ("index"), index #5=3 ("index"), index #6=2 ("index"), index #7=1 ("index"), index #8=0 ("index")) -> (element #5=→"TS-OV":bool, element #6=→"OT":bool, element #7=→"OV":bool, element #8=→"UV":bool)  [unwired: 4 out]
            n610 = Not(x=w1063) -> (.not. x?=→"BSPD 5kW" →"BSPD 5kW":bool)
            n611 = Not(x=w1059) -> (.not. x?=→"PC State" →"PC State 2":bool)
            n612 = Not(x=w1061) -> (.not. x?=→"BSPD Brake" →"BSPD Brake":bool)
          }
          frame 560 {
            n613 = Index Array(array=w1165, index=9) -> (element=w1164:u8)
            n614 = Index Array(array=w1165, index=7) -> (element=w1169:u8)
            n615 = Index Array(array=w1165, index=8) -> (element=w1144:u8)
            n616 = Index Array(array=w1165, index=6) -> (element=w1156:u8)
            n617 = Index Array(array=w1165, index=5) -> (element=w1174:u8)
            n618 = Index Array(array=w1165, index=4) -> (element=w1134:u8)
            n619 = Index Array(array=w1165, index=3) -> (element=w1181:u8)
            n620 = Index Array(array=w1165, index=2) -> (element=w1150:u8)
            n621 = And(x=w1156, y=u8 15) -> (x .and. y?=w1155:u8)
            n622 = And(x=w1144, y=u8 15) -> (x .and. y?=w1143:u8)
            n623 = And(x=w1134, y=u8 15) -> (x .and. y?=w1135:u8)
            n624 = To Unsigned Byte Integer(number=w1155) -> (unsigned 8bit integer=w1170:u8)
            n625 = And(x=w1150, y=u8 240) -> (x .and. y?=w1151:u8)
            n626 = Join Numbers(hi=w1143, lo=w1164) -> ((hi.lo)=→"STA2_Raw":u16)
            n627 = And(x=w1150, y=u8 15) -> (x .and. y?=w1153:u8)
            n628 = And(x=w1134, y=u8 240) -> (x .and. y?=w1137:u8)
            n629 = Join Numbers(hi=w1170, lo=w1169) -> ((hi.lo)=w1140:u16)
            n630 = To Unsigned Byte Integer(number=w1135) -> (unsigned 8bit integer=w1175:u8)
            n631 = To Unsigned Byte Integer(number=w1153) -> (unsigned 8bit integer=w1180:u8)
            n632 = To Double Precision Float(number=w1140) -> (double precision float=w1139:dbl)
            "STA1_Raw" <- w1139
            n633 = Join Numbers(hi=w1175, lo=w1174) -> ((hi.lo)=→"APPS2" →"Apps2":u16)
            n634 = Join Numbers(hi=w1180, lo=w1181) -> ((hi.lo)=w1147:u16)
            "APPS1" <- w1147
            "Apps1" <- w1147
            "TorqRaw" <- w1147
            n635 = Subtract(x=w1139, y=u16 90) -> (x-y=→"Steering Angle":dbl)
            n636 = local read "BrakeRaw"() -> (w1146:u16)
            n637 = To Double Precision Float(number=w1147) -> (double precision float=w1178:dbl)
            n638 = Multiply(x=0.1, y=w1178) -> (x*y=→"Torque":dbl)
            n639 = Bundle(w1147, "BrakeRaw"=w1146) -> (→"Pedal Signals":cluster{u16, "BrakeRaw":u16})  [unwired: 1 in]
            n640 = Number To Boolean Array(number=w1151) -> (Boolean array=w1163:bool[])
            n641 = Number To Boolean Array(number=w1137) -> (Boolean array=w1158:bool[])
            n642 = Index Array(array=w1163, index #1=6, index #2=7) -> (element #1=w1132:bool, element #2=w1131:bool)
            "TPS1V" <- w1132
            "TPS2V" <- w1131
            n643 = Index Array(array=w1158, index #1=7, index #2=6) -> (element #1=w1130:bool, element #2=w1129:bool)
            "STA1" <- w1130
            "STA2" <- w1129
            n644 = local read "BPPS1V"() -> (w1128:bool)
            n645 = local read "BPPS2V"() -> (w1127:bool)
            n646 = local read "BPRV"() -> (w1126:bool)
            n647 = local read "BPFV"() -> (w1125:bool)
            n648 = Build Array(w1132, w1131, w1130, w1129, w1128, w1127, w1126, w1125) -> (→"Sensor Check":bool[])
          }
          frame 561 {
            w1221 = 0.1
            w1226 = 0
            w1229 = 4
            w1215 = 5
            w1214 = 6
            w1210 = 7
            n649 = Index Array(array=w1193, index=8) -> (element=w1198:u8)
            n650 = Index Array(array=w1193, index=6) -> (element=w1204:u8)
            n651 = Index Array(array=w1193, index=3) -> (element=w1232:u8)
            n652 = Index Array(array=w1193, index=w1214) -> (element=w1217:u8)
            n653 = Index Array(array=w1193, index=w1210) -> (element=w1212:u8)
            n654 = Index Array(array=w1193, index=2) -> (element=w1207:u8)
            n655 = Number To Boolean Array(number=w1217) -> (Boolean array=w1216:bool[])
            n656 = Number To Boolean Array(number=w1207) -> (Boolean array=w1241:bool[])
            n657 = Index Array(array=w1193, index=w1215) -> (element=w1223:u8)
            n658 = Index Array(array=w1193, index=w1229) -> (element=w1228:u8)
            n659 = Index Array(array=w1193, index=9) -> (element=w1194:u8)
            n660 = Index Array(array=w1193, index=7) -> (element=w1200:u8)
            n661 = And(x=w1198, y=u8 15) -> (x .and. y?=w1195:u8)
            n662 = And(x=w1204, y=u8 15) -> (x .and. y?=w1201:u8)
            n663 = Index Array(array=w1216, index=w1210) -> (element=→"BPFV":bool)
            n664 = Number To Boolean Array(number=w1212) -> (Boolean array=w1211:bool[])
            n665 = Split Number(x=w1207) -> (lo(x)=w1231:u8)  [unwired: 1 out]
            n666 = Split Number(x=w1228) -> (lo(x)=w1227:u8)  [unwired: 1 out]
            n667 = Index Array(array=w1211, index=w1210) -> (element=→"BPRV":bool)
            n668 = Join Numbers(hi=w1201, lo=w1200) -> ((hi.lo)=w1192:u16)
            n669 = Join Numbers(hi=w1195, lo=w1194) -> ((hi.lo)=w1191:u16)
            n670 = Index Array(array=w1241, index #1=w1210, index #2=w1214, index #3=w1215, index #4=w1229) -> (element #1=→"Brake Pausability":bool, element #2=→"BPPS1V":bool, element #3=→"BPPS2V":bool, element #4=→"Braking":bool)
            n671 = Join Numbers(hi=w1226, lo=w1227) -> ((hi.lo)=w1225:u64)
            n672 = Join Numbers(hi=w1226, lo=w1231) -> ((hi.lo)=w1230:u64)
            n673 = To Unsigned Byte Integer(number=w1225) -> (unsigned 8bit integer=w1224:u8)
            n674 = To Unsigned Byte Integer(number=w1230) -> ()  [unwired: 1 out]
            n675 = Join Numbers(hi=w1224, lo=w1223) -> ((hi.lo)=w1222:u16)
            "brake2" <- w1222
            n676 = And(x=w1207, y=u8 15) -> (x .and. y?=w1206:u8)
            n677 = Join Numbers(hi=w1206, lo=w1232) -> ((hi.lo)=w1189:u16)
            "brake1" <- w1189
            "BrakeRaw" <- w1189
            n678 = Multiply(x=w1221, y=w1222) -> (x*y=→"Brake2":dbl)
            n679 = Multiply(x=w1221, y=w1189) -> (x*y=→"Brake Encoder" →"Brake1":dbl)
            n680 = Bundle(w1192, w1191) -> ()  [unwired: 1 in, 1 out]
          }
          frame 644 {
            # "MCU FL"
            n681 = Index Array(array=w1245, index=3) -> (element=w1244:u8)
            n682 = Index Array(array=w1245, index=5) -> (element=w1276:u8)
            n683 = Index Array(array=w1245, index=4) -> (element=w1275:u8)
            n684 = Index Array(array=w1245, index=7) -> (element=w1261:u8)
            n685 = Index Array(array=w1245, index=6) -> (element=w1260:u8)
            n686 = Index Array(array=w1245, index=9) -> (element=w1267:u8)
            n687 = Index Array(array=w1245, index=8) -> (element=w1266:u8)
            n688 = Number To Boolean Array(number=w1244) -> (Boolean array=→"Status FL":bool[])
            n689 = Join Numbers(hi=w1276, lo=w1275) -> ((hi.lo)=w1265:u16)
            n690 = Join Numbers(hi=w1261, lo=w1260) -> ((hi.lo)=w1253:u16)
            n691 = Join Numbers(hi=w1267, lo=w1266) -> ((hi.lo)=w1251:u16)
            n692 = To Word Integer(number=w1265) -> (16bit integer=→"Actual Velocity\nFL [RPM]":i16)
            n693 = To Word Integer(number=w1253) -> (16bit integer=w1252:i16)
            n694 = To Word Integer(number=w1251) -> (16bit integer=w1250:i16)
            n695 = Multiply(x=w1252, y=105.0) -> (x*y=w1259:dbl)
            n696 = Multiply(x=w1250, y=105.0) -> (x*y=w1254:dbl)
            n697 = Divide(x=w1259, y=16384.0) -> (x/y=w1249:dbl)
            "Id FL [A]" <- w1249
            n698 = Divide(x=w1254, y=16384.0) -> (x/y=w1248:dbl)
            "Iq FL [A]" <- w1248
            n699 = Bundle(w1249, w1248) -> (→"MCU FL":cluster{dbl, dbl})  [unwired: 1 in]
          }
          frame 645 {
            # "MCU FR"
            n700 = Index Array(array=w1279, index=9) -> (element=w1303:u8)
            n701 = Index Array(array=w1279, index=8) -> (element=w1302:u8)
            n702 = Index Array(array=w1279, index=5) -> (element=w1312:u8)
            n703 = Index Array(array=w1279, index=4) -> (element=w1311:u8)
            n704 = Index Array(array=w1279, index=7) -> (element=w1297:u8)
            n705 = Index Array(array=w1279, index=6) -> (element=w1296:u8)
            n706 = Index Array(array=w1279, index=3) -> (element=w1281:u8)
            n707 = Number To Boolean Array(number=w1281) -> (Boolean array=→"Status FR":bool[])
            n708 = Join Numbers(hi=w1303, lo=w1302) -> ((hi.lo)=w1287:u16)
            n709 = Join Numbers(hi=w1312, lo=w1311) -> ((hi.lo)=w1301:u16)
            n710 = Join Numbers(hi=w1297, lo=w1296) -> ((hi.lo)=w1289:u16)
            n711 = To Word Integer(number=w1287) -> (16bit integer=w1286:i16)
            n712 = To Word Integer(number=w1301) -> (16bit integer=→"Actual Velocity\nFR [RPM]":i16)
            n713 = To Word Integer(number=w1289) -> (16bit integer=w1288:i16)
            n714 = Multiply(x=w1286, y=105.0) -> (x*y=w1290:dbl)
            n715 = Multiply(x=w1288, y=105.0) -> (x*y=w1295:dbl)
            n716 = Divide(x=w1290, y=16384.0) -> (x/y=w1284:dbl)
            "Iq FR [A]" <- w1284
            n717 = Divide(x=w1295, y=16384.0) -> (x/y=w1285:dbl)
            "Id FR [A]" <- w1285
            n718 = Bundle(w1285, w1284) -> (→"MCU FR":cluster{dbl, dbl})  [unwired: 1 in]
          }
          frame 646 {
            # "MCU FL"
            n719 = Index Array(array=w1324, index=5) -> (element=w1326:u8)
            n720 = Index Array(array=w1324, index=4) -> (element=w1325:u8)
            n721 = Index Array(array=w1324, index=7) -> (element=w1331:u8)
            n722 = Index Array(array=w1324, index=6) -> (element=w1330:u8)
            n723 = Index Array(array=w1324, index=3) -> (element=w1340:u8)
            n724 = Index Array(array=w1324, index=2) -> (element=w1339:u8)
            n725 = Join Numbers(hi=w1326, lo=w1325) -> ((hi.lo)=w1323:u16)
            n726 = Join Numbers(hi=w1331, lo=w1330) -> ((hi.lo)=w1316:u16)
            n727 = Join Numbers(hi=w1340, lo=w1339) -> ((hi.lo)=w1329:u16)
            n728 = To Word Integer(number=w1323) -> (16bit integer=w1318:i16)
            n729 = To Unsigned Word Integer(number=w1316) -> (unsigned 16bit integer=→"Error Info FL":u16)
            n730 = To Word Integer(number=w1329) -> (16bit integer=w1321:i16)
            n731 = Divide(x=w1318, y=10.0) -> (x/y=→"T Inv. FL [°C]":dbl)
            n732 = Divide(x=w1321, y=10.0) -> (x/y=→"T Motor FL [°C]":dbl)
          }
          frame 647 {
            # "MCU FR"
            n733 = Index Array(array=w1352, index=5) -> (element=w1354:u8)
            n734 = Index Array(array=w1352, index=4) -> (element=w1353:u8)
            n735 = Index Array(array=w1352, index=7) -> (element=w1359:u8)
            n736 = Index Array(array=w1352, index=6) -> (element=w1358:u8)
            n737 = Index Array(array=w1352, index=3) -> (element=w1368:u8)
            n738 = Index Array(array=w1352, index=2) -> (element=w1367:u8)
            n739 = Join Numbers(hi=w1354, lo=w1353) -> ((hi.lo)=w1351:u16)
            n740 = Join Numbers(hi=w1359, lo=w1358) -> ((hi.lo)=w1344:u16)
            n741 = Join Numbers(hi=w1368, lo=w1367) -> ((hi.lo)=w1357:u16)
            n742 = To Word Integer(number=w1351) -> (16bit integer=w1346:i16)
            n743 = To Unsigned Word Integer(number=w1344) -> (unsigned 16bit integer=→"Error Info FR":u16)
            n744 = To Word Integer(number=w1357) -> (16bit integer=w1349:i16)
            n745 = Divide(x=w1346, y=10.0) -> (x/y=→"T Inv. FR [°C]":dbl)
            n746 = Divide(x=w1349, y=10.0) -> (x/y=→"T Motor FR [°C]":dbl)
          }
          frame 648 {
            # "MCU RL"
            n747 = Index Array(array=w1371, index=9) -> (element=w1395:u8)
            n748 = Index Array(array=w1371, index=8) -> (element=w1394:u8)
            n749 = Index Array(array=w1371, index=5) -> (element=w1404:u8)
            n750 = Index Array(array=w1371, index=4) -> (element=w1403:u8)
            n751 = Index Array(array=w1371, index=7) -> (element=w1389:u8)
            n752 = Index Array(array=w1371, index=6) -> (element=w1388:u8)
            n753 = Index Array(array=w1371, index=3) -> (element=w1373:u8)
            n754 = Number To Boolean Array(number=w1373) -> (Boolean array=→"Status RL":bool[])
            n755 = Join Numbers(hi=w1395, lo=w1394) -> ((hi.lo)=w1379:u16)
            n756 = Join Numbers(hi=w1404, lo=w1403) -> ((hi.lo)=w1393:u16)
            n757 = Join Numbers(hi=w1389, lo=w1388) -> ((hi.lo)=w1381:u16)
            n758 = To Word Integer(number=w1379) -> (16bit integer=w1378:i16)
            n759 = To Word Integer(number=w1393) -> (16bit integer=→"Actual Velocity\nRL [RPM]":i16)
            n760 = To Word Integer(number=w1381) -> (16bit integer=w1380:i16)
            n761 = Multiply(x=w1378, y=105.0) -> (x*y=w1382:dbl)
            n762 = Multiply(x=w1380, y=105.0) -> (x*y=w1387:dbl)
            n763 = Divide(x=w1382, y=16384.0) -> (x/y=w1375:dbl)
            "Iq RL [A]" <- w1375
            n764 = Divide(x=w1387, y=16384.0) -> (x/y=w1376:dbl)
            "Id RL [A]" <- w1376
            n765 = Bundle(w1376, w1375) -> (→"MCU RL":cluster{dbl, dbl})  [unwired: 1 in]
          }
          frame 649 {
            w1408 = 3.6 ("y")
            # "MCU RR"
            n766 = Index Array(array=w1452, index=9) -> (element=w1476:u8)
            n767 = Index Array(array=w1452, index=8) -> (element=w1475:u8)
            n768 = Index Array(array=w1452, index=5) -> (element=w1485:u8)
            n769 = Index Array(array=w1452, index=4) -> (element=w1484:u8)
            n770 = Index Array(array=w1452, index=7) -> (element=w1470:u8)
            n771 = Index Array(array=w1452, index=6) -> (element=w1469:u8)
            n772 = Index Array(array=w1452, index=3) -> (element=w1454:u8)
            n773 = Number To Boolean Array(number=w1454) -> (Boolean array=→"Status RR":bool[])
            n774 = flat-sequence {
              frame #0 {
                w1490 = i16 10 ("y")
                w1512 = 15.6 ("y")
                n775 = local read "Actual Velocity \nRR [RPM]"() -> (w1491:i16)
                n776 = local read "Actual Velocity\nFL [RPM]"() -> (w1494:i16)
                n777 = local read "Actual Velocity\nFR [RPM]"() -> (w1493:i16)
                n778 = local read "Actual Velocity\nRL [RPM]"() -> (w1492:i16)
                n779 = Less?(x=w1494, y=w1490) -> (x < y?=w1498:bool)
                n780 = Less?(x=w1493, y=w1490) -> (x < y?=w1497:bool)
                n781 = Less?(x=w1492, y=w1490) -> (x < y?=w1496:bool)
                n782 = To Double Precision Float(number=w1492) -> (double precision float=w1505:dbl)
                n783 = To Double Precision Float(number=w1491) -> (double precision float=w1504:dbl)
                n784 = Less?(x=w1491, y=w1490) -> (x < y?=w1495:bool)
                n785 = Add(x=w1505, y=w1504) -> (x+y=w1507:dbl)
                n786 = local read "START"() -> (w1488:bool)
                n787 = Compound Arithmetic op=AND(w1488, w1498, w1497, w1496, w1495) -> (→"IsStopped":bool)
                n788 = Divide(x=w1507, y=2.0) -> (x/y=w1501:dbl)
                n789 = feedback #28() -> (w1502:dbl)  [unwired: 1 in]
                n790 = formula code="y_=a*x+(1-a)*y;"("x"=w1501, "y"=w1502, "a"=0.1 ("input variable")) -> ("y_"=w1500:dbl)
                n791 = feedback-in #28(w1500) -> ()
                n792 = Multiply(x=w1500, y=0.104719755) -> (x*y=w1515:dbl)
                n793 = local read "Torq_sum"() -> (w1510:dbl)
                n794 = Multiply(x=w1515, y=0.227) -> (x*y=w1509:dbl)
                n795 = Divide(x=w1509, y=w1512) -> (x/y=w1508:dbl)
                n796 = Multiply(x=w1510, y=w1512) -> (x*y=→"Torque [Nm]":dbl)
                n797 = Multiply(x=w1508, y=3.6) -> (x*y=→"Velocity [km/h]":dbl)
              }
            }
            n798 = Join Numbers(hi=w1476, lo=w1475) -> ((hi.lo)=w1460:u16)
            n799 = Join Numbers(hi=w1485, lo=w1484) -> ((hi.lo)=w1474:u16)
            n800 = Join Numbers(hi=w1470, lo=w1469) -> ((hi.lo)=w1462:u16)
            n801 = To Word Integer(number=w1460) -> (16bit integer=w1459:i16)
            n802 = To Word Integer(number=w1474) -> (16bit integer=→"Actual Velocity \nRR [RPM]":i16)
            n803 = To Word Integer(number=w1462) -> (16bit integer=w1461:i16)
            n804 = Multiply(x=w1459, y=105.0) -> (x*y=w1463:dbl)
            n805 = Multiply(x=w1461, y=105.0) -> (x*y=w1468:dbl)
            n806 = Divide(x=w1463, y=16384.0) -> (x/y=w1457:dbl)
            "Iq RR [A]" <- w1457
            n807 = Divide(x=w1468, y=16384.0) -> (x/y=w1458:dbl)
            "Id RR [A]" <- w1458
            n808 = local read "Actual Velocity \nRR [RPM]"() -> (w1435:i16)
            n809 = local read "Actual Velocity\nFL [RPM]"() -> (w1432:i16)
            n810 = local read "Actual Velocity\nFR [RPM]"() -> (w1433:i16)
            n811 = local read "Actual Velocity\nRL [RPM]"() -> (w1434:i16)
            n812 = local read "Vel_acc"() -> (w1427:dbl)
            n813 = Bundle(w1458, w1457) -> (→"MCU RR":cluster{dbl, dbl})  [unwired: 1 in]
            n814 = Divide(x=w1427, y=0.227) -> (x/y=w1425:dbl)
            n815 = Multiply(x=15.6, y=w1425) -> (x*y=w1411:dbl)
            n816 = To Double Precision Float(number=w1432) -> (double precision float=w1431:dbl)
            n817 = To Double Precision Float(number=w1433) -> (double precision float=w1430:dbl)
            n818 = To Double Precision Float(number=w1434) -> (double precision float=w1429:dbl)
            n819 = To Double Precision Float(number=w1435) -> (double precision float=w1428:dbl)
            n820 = Multiply(x=30.0, y=w1411) -> (x*y=w1423:dbl)
            n821 = Divide(x=w1423, y=3.141592653589793) -> (x/y=w1417:dbl)
            n822 = Subtract(x=w1431, y=w1417) -> (x-y=w1421:dbl)
            n823 = Subtract(x=w1430, y=w1417) -> (x-y=w1420:dbl)
            n824 = Subtract(x=w1429, y=w1417) -> (x-y=w1419:dbl)
            n825 = Subtract(x=w1428, y=w1417) -> (x-y=w1418:dbl)
            n826 = Divide(x=w1421, y=w1417) -> (x/y=w1416:dbl)
            n827 = Divide(x=w1420, y=w1417) -> (x/y=w1415:dbl)
            n828 = Divide(x=w1419, y=w1417) -> (x/y=w1414:dbl)
            n829 = Divide(x=w1418, y=w1417) -> (x/y=w1413:dbl)
            n830 = local read "Id FR [A]"() -> (w1445:dbl)
            n831 = local read "Id RL [A]"() -> (w1444:dbl)
            n832 = local read "Id RR [A]"() -> (w1443:dbl)
            n833 = local read "Id FL [A]"() -> (w1446:dbl)
            n834 = Bundle(w1416, w1415, w1414, w1413) -> (→"Slip":cluster{dbl, dbl, dbl, dbl})  [unwired: 1 in]
            n835 = Build Array(w1446, w1445, w1444, w1443) -> (w1442:dbl[])
            n836 = local read "Velocity [km/h]"() -> (w1439:dbl)
            n837 = local read "Vel_acc"() -> (w1436:dbl)
            n838 = local read "TCU_v"() -> (w1409:dbl)
            n839 = call "Curr2Torq.vi"("Current"=w1442) -> ("Torque"=w1441:dbl[])
            n840 = Add Array Elements(numeric array=w1441) -> (sum=w1440:dbl)
            "Torq_sum" <- w1440
            n841 = Multiply(x=w1436, y=w1408) -> (x*y=w1437:dbl)
            n842 = Multiply(x=w1408, y=w1409) -> (x*y=w1407:dbl)
            n843 = Bundle("Velocity [km/h]"=w1439, "Torque"=w1440, w1437, w1407) -> (→"?":T3)  [unwired: 1 in]
            n844 = local read "Actual Velocity \nRR [RPM]"() -> (w1448:i16)
            n845 = local read "Actual Velocity\nFL [RPM]"() -> (w1451:i16)
            n846 = local read "Actual Velocity\nFR [RPM]"() -> (w1450:i16)
            n847 = local read "Actual Velocity\nRL [RPM]"() -> (w1449:i16)
            n848 = Bundle("Actual Velocity\nFL [RPM]"=w1451, "Actual Velocity\nFR [RPM]"=w1450, "Actual Velocity\nRL [RPM]"=w1449, "Actual Velocity \nRR [RPM]"=w1448) -> (→"Angular Speed":T8)  [unwired: 1 in]
          }
          frame 650 {
            # "MCU RL"
            n849 = Index Array(array=w1526, index=5) -> (element=w1528:u8)
            n850 = Index Array(array=w1526, index=4) -> (element=w1527:u8)
            n851 = Index Array(array=w1526, index=7) -> (element=w1533:u8)
            n852 = Index Array(array=w1526, index=6) -> (element=w1532:u8)
            n853 = Index Array(array=w1526, index=3) -> (element=w1542:u8)
            n854 = Index Array(array=w1526, index=2) -> (element=w1541:u8)
            n855 = Join Numbers(hi=w1528, lo=w1527) -> ((hi.lo)=w1525:u16)
            n856 = Join Numbers(hi=w1533, lo=w1532) -> ((hi.lo)=w1518:u16)
            n857 = Join Numbers(hi=w1542, lo=w1541) -> ((hi.lo)=w1531:u16)
            n858 = To Word Integer(number=w1525) -> (16bit integer=w1520:i16)
            n859 = To Unsigned Word Integer(number=w1518) -> (unsigned 16bit integer=→"Error Info RL":u16)
            n860 = To Word Integer(number=w1531) -> (16bit integer=w1523:i16)
            n861 = Divide(x=w1520, y=10.0) -> (x/y=→"T Inv. RL [°C]":dbl)
            n862 = Divide(x=w1523, y=10.0) -> (x/y=→"T Motor RL [°C]":dbl)
          }
          frame 651 {
            # "MCU RR"
            n863 = Index Array(array=w1554, index=5) -> (element=w1556:u8)
            n864 = Index Array(array=w1554, index=4) -> (element=w1555:u8)
            n865 = Index Array(array=w1554, index=7) -> (element=w1561:u8)
            n866 = Index Array(array=w1554, index=6) -> (element=w1560:u8)
            n867 = Index Array(array=w1554, index=3) -> (element=w1570:u8)
            n868 = Index Array(array=w1554, index=2) -> (element=w1569:u8)
            n869 = Join Numbers(hi=w1556, lo=w1555) -> ((hi.lo)=w1553:u16)
            n870 = Join Numbers(hi=w1561, lo=w1560) -> ((hi.lo)=w1546:u16)
            n871 = Join Numbers(hi=w1570, lo=w1569) -> ((hi.lo)=w1559:u16)
            n872 = To Word Integer(number=w1553) -> (16bit integer=w1548:i16)
            n873 = To Unsigned Word Integer(number=w1546) -> (unsigned 16bit integer=→"Error Info RR":u16)
            n874 = To Word Integer(number=w1559) -> (16bit integer=w1551:i16)
            n875 = Divide(x=w1548, y=10.0) -> (x/y=→"T Inv. RR [°C]":dbl)
            n876 = Divide(x=w1551, y=10.0) -> (x/y=→"T Motor RR [°C]":dbl)
          }
          frame 656 {
            n877 = Index Array(array=w1611, index=5) -> (element=w1604:u8)
            n878 = Index Array(array=w1611, index=4) -> (element=w1602:u8)
            n879 = Index Array(array=w1611, index=3) -> (element=w1595:u8)
            n880 = And(x=w1604, y=u8 15) -> (x .and. y?=→"Dial 5":u8)
            n881 = And(x=w1602, y=u8 15) -> (x .and. y?=w1577:u8)
            "Dial 3" <- w1577
            n882 = And(x=w1595, y=u8 15) -> (x .and. y?=→"Dial":u8)
            n883 = And(x=w1604, y=u8 240) -> (x .and. y?=w1599:u8)
            n884 = And(x=w1602, y=u8 240) -> (x .and. y?=w1601:u8)
            n885 = And(x=w1595, y=u8 240) -> (x .and. y?=w1594:u8)
            n886 = Logical Shift(y=i16 -4, x=w1599) -> (x << y=→"Dial 4":u8)
            n887 = Logical Shift(y=i16 -4, x=w1601) -> (x << y=w1574:u8)
            "Dial 2" <- w1574
            n888 = Logical Shift(y=i16 -4, x=w1594) -> (x << y=w1589:u8)
            n889 = formula code="if(in1==1) out1=1;\nif(in1==2) out1=0.95;\nif(in1==3) out1=0.9;\nif(in1==4) out1=0.85;\nif(in1==5) out1=0.8;\nif(in1==6) out1=0.75;\nif(in1==7) out1=0.7;\nif(in1==8) out1=0.65;\nif(in1==9) out1=0.6;\nif(in1==10) out1=0.55;\nif(in1==11) out1=0.5;\nif(in1==12) out1=0.4;"("in1"=w1574) -> ("out1"=→"Rear Reduction":dbl)
            n890 = Number To Boolean Array(number=w1589) -> (Boolean array=w1588:bool[])
            n891 = Multiply(x=4.16666, y=w1577) -> (x*y=→"Slope":dbl)
            n892 = Index Array(array=w1588, index #1=0 ("index"), index #2=1 ("index"), index #3=2 ("index"), index #4=3 ("index")) -> (element #1=→"Boolean":bool, element #2=→"Boolean 2":bool, element #3=→"Boolean 3":bool, element #4=→"Boolean 4":bool)
          }
          frame 787 {
            # "HV Critical Cell Values"
            n893 = Index Array(array=w1618, index=5) -> (element=w1617:u8)
            n894 = Index Array(array=w1618, index=6) -> (element=w1616:u8)
            n895 = Index Array(array=w1618, index=3) -> (element=w1621:u8)
            n896 = Index Array(array=w1618, index=4) -> (element=w1622:u8)
            n897 = Join Numbers(hi=w1617, lo=w1616) -> ((hi.lo)=→"Temp Max 2":u16)
            n898 = Join Numbers(hi=w1622, lo=w1621) -> ((hi.lo)=w1623:u16)
            n899 = To Unsigned Word Integer(number=w1623) -> (unsigned 16bit integer=→"Cell Min 2":u16)
          }
          frame 800 {
            # "MCU Support Status kesz"
            n900 = Index Array(array=w1639, index=3) -> (element=w1665:u8)
            n901 = Number To Boolean Array(number=w1665) -> (Boolean array=w1674:bool[])
            n902 = Index Array(array=w1639, index=4) -> (element=w1652:u8)
            n903 = Number To Boolean Array(number=w1652) -> (Boolean array=w1653:bool[])
            n904 = Index Array(array=w1674, index #1=7 ("index"), index #2=6 ("index"), index #3=5 ("index"), index #4=4 ("index"), index #5=3 ("index"), index #6=2 ("index"), index #7=1 ("index"), index #8=0 ("index")) -> (element #1=→"Brake Light":bool, element #2=→"MCU EF":bool, element #3=→"MCU RF":bool, element #4=→"RTDS":bool, element #5=→"TCU Power":bool, element #6=→"24V front DC/DC":bool, element #7=→"24V rear DC/DC":bool, element #8=→"LKS & RKS" →"LKS & RKS" →"SC RKS" →"SC LKS":bool)
            n905 = Index Array(array=w1653, index #1=7 ("index"), index #2=6 ("index"), index #3=5 ("index"), index #4=4 ("index"), index #5=3 ("index"), index #6=2 ("index"), index #7=1 ("index"), index #8=0 ("index")) -> (element #1=→"MCU Interlocks" →"MCU Interlock" →"SC Motor 4" →"SC Motor 1" →"SC Motor 3" →"SC MCU" →"SC Motor 2" →"Motor1 Interlock" →"Motor2 Interlock" →"Motor3 Interlock" →"Motor4 Interlock" →"HVD Interlock":bool, element #2=→"ON" →"ON":bool, element #3=→"START" →"START":bool, element #4=→"OFF" →"OFF":bool, element #5=→"Logging" →"Telemetry":bool, element #6=→"TSAL":bool, element #7=→"SC State":bool, element #8=→"Car standing":bool)
            n906 = Index Array(array=w1639, index=5) -> (element=w1632:u8)
            n907 = To Unsigned Word Integer(number=w1632) -> (unsigned 16bit integer=→"MCU S SC Endl":u16)
          }
          frame 816 {
            # "5db 12V"
            # "3db 48V"
            # "LV Sys Status"
            n908 = Index Array(array=w1715, index=3) -> (element=w1744:u8)
            n909 = Index Array(array=w1715, index=4) -> (element=w1716:u8)
            n910 = Number To Boolean Array(number=w1744) -> (Boolean array=w1743:bool[])
            n911 = Number To Boolean Array(number=w1716) -> (Boolean array=w1734:bool[])
            n912 = Index Array(array=w1743, index #1=7 ("index"), index #2=6 ("index"), index #3=5 ("index"), index #4=4 ("index"), index #5=3 ("index"), index #6=2 ("index"), index #7=1 ("index"), index #8=0 ("index")) -> (element #1=→"Main Switch" →"Main Switch":bool, element #2=→"MP Switch" →"MP Switch":bool, element #3=→"SC BOTS &\nINS & CKS" →"SC State" →"SC State":bool, element #4=w1712:bool, element #5=w1708:bool, element #6=w1709:bool, element #7=w1710:bool, element #8=w1711:bool)
            n913 = Index Array(array=w1734, index #1=7 ("index"), index #2=6 ("index"), index #3=5 ("index")) -> (element #1=w1700:bool, element #2=w1699:bool, element #3=w1698:bool)
            n914 = Bundle(w1700, w1699, w1698) -> (w1696:cluster{bool, bool, bool})  [unwired: 1 in]
            n915 = Bundle(w1712, w1708, w1709, w1710, w1711) -> (w1706:cluster{bool, bool, bool, bool, bool})  [unwired: 1 in]
            n916 = Cluster To Array(cluster=w1706) -> (array=→"12V system":bool[])
            n917 = Unbundle(w1696) -> (→"48V Out 1":bool, →"48V Out 2":bool, →"48V Out 3":bool)
            n918 = Cluster To Array(cluster=w1696) -> (array=→"48V system":bool[])
            n919 = Unbundle(w1706) -> (→"12V Out 1":bool, →"12V Out 2" →"Radiator Cooling":bool, →"12V Out 3":bool, →"12V Out 4":bool, →"12V Out 5":bool)
            n920 = Index Array(array=w1715, index=5) -> (element=w1687:u8)
            n921 = Index Array(array=w1715, index=6) -> (element=w1729:u8)
            n922 = And(x=w1687, y=u8 15) -> (x .and. y?=→"Undervoltage Errrors":u8)
            n923 = Number To Boolean Array(number=w1729) -> (Boolean array=w1728:bool[])
            n924 = And(x=240, y=w1687) -> (x .and. y?=w1688:i32)
            n925 = Index Array(array=w1728, index #1=7 ("index"), index #2=6 ("index"), index #3=5 ("index"), index #4=4 ("index"), index #5=3 ("index"), index #6=2 ("index"), index #7=1 ("index"), index #8=0 ("index")) -> (element #1=→"Battery Full" →"Battery Full":bool, element #2=→"LV Overtemp" →"LV Overtemp":bool, element #3=→"LV Undervoltage" →"LV Undervoltage":bool, element #4=→"Battery Low" →"Battery Low":bool, element #5=→"BMS IC Wake" →"BMS IC Awake":bool, element #6=→"BMS IC Fault" →"BMS IC Error":bool, element #7=→"Overvoltage":bool)  [unwired: 1 out]
            n926 = Logical Shift(y=i16 -4, x=w1688) -> (x << y=→"Overtemp Errors":i32)
          }
          frame 817 {
            # "Offset error"
            # "PDM Status"
            n927 = Index Array(array=w1765, index=4) -> (element=w1785:u8)
            n928 = Index Array(array=w1765, index=5) -> (element=w1786:u8)
            n929 = Index Array(array=w1765, index=6) -> (element=w1781:u8)
            n930 = Index Array(array=w1765, index=2) -> (element=w1777:u8)
            n931 = Index Array(array=w1765, index=7) -> (element=w1782:u8)
            n932 = Index Array(array=w1765, index=3) -> (element=w1778:u8)
            n933 = Join Numbers(hi=w1785, lo=w1786) -> ((hi.lo)=w1762:u16)
            n934 = Join Numbers(hi=w1781, lo=w1782) -> ((hi.lo)=w1754:u16)
            n935 = Join Numbers(hi=w1777, lo=w1778) -> ((hi.lo)=w1755:u16)
            n936 = To Word Integer(number=w1762) -> (16bit integer=w1761:i16)
            n937 = To Unsigned Word Integer(number=w1754) -> (unsigned 16bit integer=w1753:u16)
            n938 = To Unsigned Word Integer(number=w1755) -> (unsigned 16bit integer=w1756:u16)
            n939 = To Double Precision Float(number=w1756) -> (double precision float=w1763:dbl)
            n940 = To Double Precision Float(number=w1753) -> (double precision float=w1772:dbl)
            n941 = To Double Precision Float(number=w1761) -> (double precision float=w1760:dbl)
            n942 = feedback #29() -> (w1764:dbl)  [unwired: 1 in]
            n943 = formula code="y_=a*x+(1-a)*y;"("x"=w1763, "y"=w1764, "a"=0.1 ("input variable")) -> ("y_"=w1757:dbl)
            n944 = feedback-in #29(w1757) -> ()
            n945 = Divide(x=w1757, y=1000.0) -> (x/y=→"LV Voltage [V]":dbl)
            n946 = feedback #30() -> (w1776:dbl)  [unwired: 1 in]
            n947 = formula code="y_=a*x+(1-a)*y;"("x"=w1760, "y"=w1776, "a"=0.1 ("input variable")) -> ("y_"=w1752:dbl)
            "48V Current [mA]" <- w1752
            n948 = feedback-in #30(w1752) -> ()
            n949 = feedback #31() -> (w1774:dbl)  [unwired: 1 in]
            n950 = formula code="y_=a*x+(1-a)*y;"("x"=w1772, "y"=w1774, "a"=0.1 ("input variable")) -> ("y_"=w1751:dbl)
            "12V Current [mA]" <- w1751
            n951 = feedback-in #31(w1751) -> ()
            n952 = Bundle("y_"=w1752, "y_"=w1751) -> (→"LV Current":cluster{"y_":dbl, "y_":dbl})  [unwired: 1 in]
            n953 = Divide(x=w1752, y=1000.0) -> (x/y=→"48V Current [A]":dbl)
            n954 = Divide(x=w1751, y=1000.0) -> (x/y=→"12V Current [A]":dbl)
          }
          frame 832 {
            # "MCU Power ECU Status"
            n955 = Index Array(array=w1800, index=3) -> (element=w1852:u8)
            n956 = Index Array(array=w1800, index=4) -> (element=w1841:u8)
            n957 = Number To Boolean Array(number=w1841) -> (Boolean array=w1840:bool[])
            n958 = Number To Boolean Array(number=w1852) -> (Boolean array=w1851:bool[])
            n959 = Index Array(array=w1851, index #1=7 ("index"), index #2=6 ("index"), index #3=5 ("index"), index #4=4 ("index"), index #5=3 ("index"), index #6=2 ("index"), index #7=1 ("index")) -> (element #7=→"24V Power B":bool)  [unwired: 6 out]
            n960 = Index Array(array=w1840, index #1=7 ("index"), index #2=6 ("index"), index #3=5 ("index"), index #4=4 ("index"), index #5=3 ("index"), index #6=2 ("index"), index #7=1 ("index"), index #8=0 ("index")) -> (element #1=→"MCU EF A":bool, element #2=→"MCU EF B":bool, element #3=→"MCU EF2 A":bool, element #4=→"MCU EF2 B":bool, element #5=→"MCU RF 1":bool, element #6=→"MCU RF 2":bool, element #7=→"MCU RF 3":bool, element #8=→"MCU RF 4":bool)
            n961 = Index Array(array=w1800, index=8) -> (element=w1797:u8)
            n962 = Index Array(array=w1800, index=9) -> (element=w1796:u8)
            n963 = Index Array(array=w1800, index=6) -> (element=w1799:u8)
            n964 = Index Array(array=w1800, index=7) -> (element=w1798:u8)
            n965 = Index Array(array=w1800, index=5) -> (element=w1822:u8)
            n966 = Number To Boolean Array(number=w1822) -> (Boolean array=w1821:bool[])
            n967 = Join Numbers(hi=w1797, lo=w1796) -> ((hi.lo)=→"Power B Current":u16)
            n968 = Join Numbers(hi=w1799, lo=w1798) -> ((hi.lo)=→"Power A Current":u16)
            n969 = Index Array(array=w1821, index #1=7 ("index"), index #2=6 ("index"), index #3=5 ("index"), index #4=4 ("index"), index #5=3 ("index"), index #6=2 ("index"), index #7=1 ("index"), index #8=0 ("index")) -> (element #2=→"MCU FL 2":bool, element #3=→"MCU FL 3":bool, element #4=→"MCU FL 4":bool, element #5=→"MCU SC Endline" →"MCU SC Endline 2":bool, element #6=→"MCU TSAL":bool, element #7=→"CAN1 Term.":bool, element #8=→"CAN2 Term.":bool)  [unwired: 1 out]
          }
          frame 896 {
            w1880 = 4 ("index")
            w1864 = u8 128 ("y")
            # "TCU Status"
            n970 = Index Array(array=w1883, index=2) -> (element=w1863:u8)
            n971 = Index Array(array=w1883, index=6) -> (element=w1891:u8)
            n972 = Index Array(array=w1883, index=9) -> (element=w1860:u8)
            n973 = Index Array(array=w1883, index=4) -> (element=w1874:u8)
            n974 = Index Array(array=w1883, index=5) -> (element=w1900:u8)
            n975 = Index Array(array=w1883, index=8) -> (element=w1859:u8)
            "Regen %" <- w1859
            n976 = Index Array(array=w1883, index=3) -> (element=→"Torque %":u8)
            n977 = Index Array(array=w1883, index=7) -> (element=w1888:u8)
            n978 = To Unsigned Byte Integer(number=w1863) -> (unsigned 8bit integer=w1881:u8)
            n979 = Join Numbers(hi=w1874, lo=w1900) -> ((hi.lo)=w1871:u16)
            n980 = And(x=w1863, y=u8 15) -> (x .and. y?=→"Selector":u8)
            n981 = Divide(x=w1888, y=u8 100) -> (x/y=→"LR Bias":dbl)
            n982 = Number To Boolean Array(number=w1881) -> (Boolean array=w1882:bool[])
            n983 = And(x=w1871, y=u16 32767) -> (x .and. y?=w1870:u16)
            n984 = And(x=w1874, y=w1864) -> (x .and. y?=w1868:u8)
            n985 = To Word Integer(number=w1870) -> (16bit integer=→"Speed RPM":i16)
            n986 = Divide(x=w1868, y=w1864) -> (x/y=→"BTC":dbl)
            n987 = Array Subset(array=w1882, index=w1880, length=w1880) -> (w1879:bool[])
            n988 = formula code="if(in1==0) out1=0;\nif(in1==244) out1=5;\nif(in1==232) out1=10;\nif(in1==220) out1=15;\nif(in1==208) out1=20;\nif(in1==196) out1=25;\nif(in1==184) out1=30;\nif(in1==172) out1=35;\nif(in1==160) out1=40;\nif(in1==148) out1=45;\nif(in1==136) out1=50;\nif(in1==124) out1=55;"("in1"=w1859) -> ("out1"=→"BreakPoint":dbl)
            n989 = Reverse 1D Array(array=w1879) -> (reversed array=→"Derate":bool[])
            n990 = Divide(x=w1891, y=u8 2) -> (x/y=w1875:dbl)
            "Front" <- w1875
            n991 = Divide(x=w1860, y=u8 2) -> (x/y=w1866:dbl)
            "Rear 2" <- w1866
            n992 = Subtract(x=100.0, y=w1875) -> (x-y=→"Rear":dbl)
            n993 = Subtract(x=100.0, y=w1866) -> (x-y=→"Front 2":dbl)
          }
          frame 897 {
            w1917 = 0.6 ("x")
            w1918 = 0.6 ("y")
            # "Acceleration X & Roll"
            n994 = Index Array(array=w1963, index=9) -> (element=w1964:u8)
            n995 = Index Array(array=w1963, index=8) -> (element=w1966:u8)
            n996 = Index Array(array=w1963, index=2) -> (element=w1975:u8)
            n997 = Index Array(array=w1963, index=3) -> (element=w1974:u8)
            n998 = Index Array(array=w1963, index=4) -> (element=w1973:u8)
            n999 = Index Array(array=w1963, index=5) -> (element=w1972:u8)
            n1000 = Index Array(array=w1963, index=7) -> (element=w1968:u8)
            n1001 = Index Array(array=w1963, index=6) -> (element=w1970:u8)
            n1002 = To Byte Integer(number=w1964) -> (8bit integer=w1943:i8)
            n1003 = To Byte Integer(number=w1966) -> (8bit integer=w1944:i8)
            n1004 = To Byte Integer(number=w1972) -> (8bit integer=w1955:i8)
            n1005 = To Byte Integer(number=w1968) -> (8bit integer=w1945:i8)
            n1006 = To Byte Integer(number=w1973) -> (8bit integer=w1959:i8)
            n1007 = To Byte Integer(number=w1970) -> (8bit integer=w1946:i8)
            n1008 = To Byte Integer(number=w1974) -> (8bit integer=w1960:i8)
            n1009 = To Double Precision Float(number=w1945) -> (double precision float=w1951:dbl)
            n1010 = To Double Precision Float(number=w1943) -> (double precision float=w1947:dbl)
            n1011 = To Double Precision Float(number=w1946) -> (double precision float=w1954:dbl)
            n1012 = To Double Precision Float(number=w1944) -> (double precision float=w1950:dbl)
            n1013 = To Double Precision Float(number=w1960) -> (double precision float=w1961:dbl)
            n1014 = local read "AccelYRaw"() -> (w1978:dbl)
            n1015 = local read "AccelXRaw"() -> (w1982:dbl)
            n1016 = To Double Precision Float(number=w1975) -> (double precision float=w2002:dbl)
            n1017 = To Double Precision Float(number=w1959) -> (double precision float=w2001:dbl)
            n1018 = Divide(x=w1951, y=127.0) -> (x/y=w1941:dbl)
            "TCU_slipFR" <- w1941
            n1019 = Divide(x=w1947, y=127.0) -> (x/y=w1939:dbl)
            "TCU_slipRR" <- w1939
            n1020 = Divide(x=w1954, y=127.0) -> (x/y=w1942:dbl)
            "TCU_slipFL" <- w1942
            n1021 = Divide(x=w1950, y=127.0) -> (x/y=w1940:dbl)
            "TCU_slipRL" <- w1940
            n1022 = Divide(x=w1961, y=50.0) -> (x/y=w1908:dbl)
            "TCU_ax" <- w1908
            n1023 = Divide(x=w2001, y=50.0) -> (x/y=→"TCU_ay":dbl)
            n1024 = Divide(x=w2002, y=2.0) -> (x/y=→"TCU_v":dbl)
            n1025 = To Double Precision Float(number=w1955) -> (double precision float=w1956:dbl)
            n1026 = Divide(x=w1956, y=20.0) -> (x/y=→"TCU_yaw":dbl)
            n1027 = local read "AccelXRaw"() -> (w1907:dbl)
            n1028 = feedback #32() -> (w1983:dbl)  [unwired: 1 in]
            n1029 = formula code="y_=a*x+(1-a)*y;"("x"=w1982, "y"=w1983, "a"=0.1 ("input variable")) -> ("y_"=w1976:dbl)
            n1030 = feedback-in #32(w1976) -> ()
            n1031 = feedback #33() -> (w1980:dbl)  [unwired: 1 in]
            n1032 = formula code="y_=a*x+(1-a)*y;"("x"=w1978, "y"=w1980, "a"=0.1 ("input variable")) -> ("y_"=w1977:dbl)
            n1033 = feedback-in #33(w1977) -> ()
            n1034 = Subtract(x=w1908, y=w1907) -> (x-y=w1906:dbl)
            "Numeric" <- w1906
            n1035 = feedback #34() -> (w1997:dbl[])  [unwired: 1 in]
            n1036 = Build Array (concatenate)(w1997, w1977) -> (w1995:dbl[])
            n1037 = feedback #35() -> (w1990:dbl[])  [unwired: 1 in]
            n1038 = Build Array (concatenate)(w1990, w1976) -> (w1991:dbl[])
            n1039 = Bundle(w1908, "AccelXRaw"=w1907, w1906) -> (→"TCU speed":cluster{dbl, "AccelXRaw":dbl, dbl})  [unwired: 1 in]
            n1040 = Bundle(w1942, w1941, w1940, w1939) -> (→"Slip_TCU":cluster{dbl, dbl, dbl, dbl})  [unwired: 1 in]
            n1041 = Array Size(array=w1995) -> (size(s)=w1994:i32)
            n1042 = Build Array(w1977) -> (w1988:dbl[])
            n1043 = Build Array(w1976) -> (w1987:dbl[])
            n1044 = Less?(x=w1994, y=1000) -> (x < y?=w1992:bool)
            n1045 = local read "Acc Z offset"() -> (w1936:dbl)
            n1046 = local read "Acc Z"() -> (w1937:dbl)
            n1047 = local read "Acc X offset 2"() -> (w1935:dbl)
            n1048 = local read "Acc X 2"() -> (w1934:dbl)
            n1049 = local read "Acc Y offset"() -> (w1905:dbl)
            n1050 = local read "Acc Y"() -> (w1923:dbl)
            n1051 = local read "Acc Y 2"() -> (w1924:dbl)
            n1052 = Subtract(x=w1937, y=w1936) -> (x-y=w1933:dbl)
            n1053 = Subtract(x=w1934, y=w1935) -> (x-y=w1932:dbl)
            n1054 = Negate(x=w1933) -> (-x=w1911:dbl)
            n1055 = Subtract(x=w1923, y=w1905) -> (x-y=w1925:dbl)
            n1056 = Subtract(x=w1924, y=w1905) -> (x-y=w1926:dbl)
            n1057 = Add(x=w1911, y=w1932) -> (x+y=w1931:dbl)
            n1058 = Multiply(x=w1925, y=w1918) -> (x*y=w1922:dbl)
            n1059 = Multiply(x=w1917, y=w1926) -> (x*y=w1921:dbl)
            n1060 = Negate(x=w1931) -> (-x=w1930:dbl)
            n1061 = Add(x=w1922, y=w1921) -> (x+y=w1920:dbl)
            n1062 = Add(x=w1918, y=w1917) -> (x+y=w1919:dbl)
            n1063 = Divide(x=w1930, y=2.0) -> (x/y=w1928:dbl)
            n1064 = Negate(x=w1920) -> (-x=w1927:dbl)
            n1065 = Divide(x=w1927, y=w1919) -> (x/y=w1916:dbl)
            n1066 = Multiply(x=9.81, y=w1928) -> (x*y=→"AccelXRaw":dbl)
            n1067 = case shown="True" w1992 {
              tunnel: [w2012 w2021] -> w1989
              tunnel: w1991 -> [w2013 w2021]
              tunnel: [w2016 w2020] -> w1996
              tunnel: w1995 -> [w2019 w2020]
              frame False {
                n1068 = Delete From Array(array=w2019, length=1, index=0) -> (array with subset deleted=w2016:dbl[])  [unwired: 1 out]
                n1069 = Delete From Array(array=w2013, length=1, index=0) -> (array with subset deleted=w2012:dbl[])  [unwired: 1 out]
              }
              frame True {
              }
            }
            n1070 = feedback-in #34(w1996) -> ()
            n1071 = feedback-in #35(w1989) -> ()
            n1072 = Multiply(x=w1916, y=9.81) -> (x*y=→"AccelYRaw":dbl)
            n1073 = Bundle(w1996, w1989) -> (w1985:cluster{dbl[], dbl[]})  [unwired: 1 in]
            n1074 = Bundle(w1988, w1987) -> (w1984:cluster{dbl[], dbl[]})  [unwired: 1 in]
            n1075 = Build Array(w1984, w1985) -> (→"TCU_acc":cluster{dbl[], dbl[]}[])
          }
          frame 1028 {
            # "Pedalbox Status"
            # "Pedalbox Sensor Check"
            n1076 = Index Array(array=w2029, index=3) -> (element=w2033:u8)
            n1077 = Index Array(array=w2029, index=3) -> (element=w2041:u8)
            n1078 = Index Array(array=w2029, index=4) -> (element=w2040:u8)
            n1079 = Index Array(array=w2029, index=4) -> (element=→"PD Error Info":u8)
            n1080 = Index Array(array=w2029, index=5) -> (element=w2048:u8)
            n1081 = Index Array(array=w2029, index=6) -> (element=w2044:u8)
            n1082 = Number To Boolean Array(number=w2033) -> (Boolean array=w2032:bool[])
            n1083 = Index Array(array=w2029, index=4) -> (element=w2024:u8)
            n1084 = Join Numbers(hi=w2041, lo=w2040) -> ((hi.lo)=w2039:u16)
            n1085 = Divide(x=w2048, y=10.0) -> (x/y=→"K_Throttle":dbl)
            n1086 = Divide(x=w2044, y=10.0) -> (x/y=→"K_Brake":dbl)
            n1087 = Logical Shift(y=i16 -6, x=w2024) -> (x << y=w2023:u8)
            n1088 = Logical Shift(y=i16 -7, x=w2039) -> (x << y=w2037:u16)
            n1089 = Index Array(array=w2032, index=7) -> (element=→"BOTS & INS & CKS":bool)
            n1090 = And(x=w2037, y=u8 255) -> (x .and. y?=w2035:u16)
            n1091 = And(x=w2023, y=u8 1) -> (x .and. y?=w2022:u8)
            n1092 = To Unsigned Byte Integer(number=w2035) -> (unsigned 8bit integer=w2034:u8)
            n1093 = Number To Boolean Array(number=w2034) -> ()  [unwired: 1 out]
            n1094 = Add(x=w2022, y=u16 2016) -> (x+y=→"TCU Version":u16)
          }
          frame 1029 {
            # "Throttle EEPROM"
            n1095 = Index Array(array=w2065, index=2) -> (element=w2077:u8)
            n1096 = Index Array(array=w2065, index=3) -> (element=w2076:u8)
            n1097 = Index Array(array=w2065, index=4) -> (element=w2075:u8)
            n1098 = Index Array(array=w2065, index=5) -> (element=w2074:u8)
            n1099 = Index Array(array=w2065, index=6) -> (element=w2069:u8)
            n1100 = Index Array(array=w2065, index=7) -> (element=w2068:u8)
            n1101 = Index Array(array=w2065, index=8) -> (element=w2067:u8)
            n1102 = Index Array(array=w2065, index=9) -> (element=w2066:u8)
            n1103 = Join Numbers(hi=w2077, lo=w2076) -> ((hi.lo)=→"APPS1 ADC Min":u16)
            n1104 = Join Numbers(hi=w2075, lo=w2074) -> ((hi.lo)=→"APPS1 ADC Max":u16)
            n1105 = Join Numbers(hi=w2069, lo=w2068) -> ((hi.lo)=→"APPS2 ADC Min":u16)
            n1106 = Join Numbers(hi=w2067, lo=w2066) -> ((hi.lo)=→"APPS2 ADC Max":u16)
          }
          frame 1030 {
            # "Steering EEPROM"
            n1107 = Index Array(array=w2089, index=2) -> (element=w2096:u8)
            n1108 = Index Array(array=w2089, index=3) -> (element=w2095:u8)
            n1109 = Index Array(array=w2089, index=6) -> (element=w2092:u8)
            n1110 = Index Array(array=w2089, index=7) -> (element=w2091:u8)
            n1111 = Join Numbers(hi=w2096, lo=w2095) -> ((hi.lo)=→"STA1 ADC 90":u16)
            n1112 = Join Numbers(hi=w2092, lo=w2091) -> ((hi.lo)=→"STA2 ADC 90":u16)
          }
          frame 1031 {
            # "Brake EEPROM"
            n1113 = Index Array(array=w2107, index=2) -> (element=w2124:u8)
            n1114 = Index Array(array=w2107, index=3) -> (element=w2123:u8)
            n1115 = Index Array(array=w2107, index=4) -> (element=w2122:u8)
            n1116 = Index Array(array=w2107, index=5) -> (element=w2121:u8)
            n1117 = Index Array(array=w2107, index=6) -> (element=w2116:u8)
            n1118 = Index Array(array=w2107, index=7) -> (element=w2115:u8)
            n1119 = Index Array(array=w2107, index=8) -> (element=w2114:u8)
            n1120 = Index Array(array=w2107, index=9) -> (element=w2113:u8)
            n1121 = Join Numbers(hi=w2124, lo=w2123) -> ((hi.lo)=→"BSE1 ADC Min":u16)
            n1122 = Join Numbers(hi=w2122, lo=w2121) -> ((hi.lo)=→"BSE1 ADC Max":u16)
            n1123 = Join Numbers(hi=w2116, lo=w2115) -> ((hi.lo)=→"BSE2 ADC Max":u16)
            n1124 = Join Numbers(hi=w2114, lo=w2113) -> ((hi.lo)=→"BSE2 ADC Min":u16)
          }
          frame 1032 {
            # "Steering Middle EEPROM"
            n1125 = Index Array(array=w2131, index=2) -> (element=w2140:u8)
            n1126 = Index Array(array=w2131, index=3) -> (element=w2139:u8)
            n1127 = Index Array(array=w2131, index=4) -> (element=w2138:u8)
            n1128 = Index Array(array=w2131, index=5) -> (element=w2137:u8)
            n1129 = Join Numbers(hi=w2140, lo=w2139) -> ((hi.lo)=→"STA1 ADC Null":u16)
            n1130 = Join Numbers(hi=w2138, lo=w2137) -> ((hi.lo)=→"STA2 ADC Null":u16)
          }
          frame 1057 {
            w2145 = 0.1 ("input variable")
            n1131 = Index Array(array=w2191, index=8) -> (element=w2151:u8)
            n1132 = Index Array(array=w2191, index=9) -> (element=w2150:u8)
            n1133 = Index Array(array=w2191, index=7) -> (element=w2162:u8)
            n1134 = Index Array(array=w2191, index=6) -> (element=w2161:u8)
            n1135 = To Double Precision Float(number=w2151) -> (double precision float=w2147:dbl)
            "S Radiator Right IN" <- w2147
            n1136 = Index Array(array=w2191, index=4) -> (element=w2169:u8)
            n1137 = Index Array(array=w2191, index=5) -> (element=w2170:u8)
            n1138 = To Double Precision Float(number=w2150) -> (double precision float=w2146:dbl)
            "S Radiator Right OUT" <- w2146
            n1139 = Index Array(array=w2191, index=2) -> (element=w2177:u8)
            n1140 = Index Array(array=w2191, index=3) -> (element=w2174:u8)
            n1141 = To Double Precision Float(number=w2162) -> (double precision float=w2148:dbl)
            "S Radiator Left OUT" <- w2148
            n1142 = To Double Precision Float(number=w2161) -> (double precision float=w2149:dbl)
            "S Radiator Left IN" <- w2149
            n1143 = To Double Precision Float(number=w2169) -> (double precision float=w2167:dbl)
            "MCU Radiator Right IN" <- w2167
            n1144 = To Double Precision Float(number=w2170) -> (double precision float=w2165:dbl)
            "MCU Radiator Right OUT" <- w2165
            n1145 = To Double Precision Float(number=w2174) -> (double precision float=w2172:dbl)
            "MCU Radiator Left OUT" <- w2172
            n1146 = To Double Precision Float(number=w2177) -> (double precision float=w2176:dbl)
            "MCU Radiator Left IN" <- w2176
            n1147 = feedback #36() -> (w2155:dbl)  [unwired: 1 in]
            n1148 = formula code="y_=a*x+(1-a)*y;"("x"=w2146, "y"=w2155, "a"=w2145) -> ("y_"=w2153:dbl)
            n1149 = feedback-in #36(w2153) -> ()
            n1150 = feedback #37() -> (w2156:dbl)  [unwired: 1 in]
            n1151 = formula code="y_=a*x+(1-a)*y;"("x"=w2147, "y"=w2156, "a"=w2145) -> ("y_"=w2154:dbl)
            n1152 = feedback-in #37(w2154) -> ()
            n1153 = feedback #38() -> (w2168:dbl)  [unwired: 1 in]
            n1154 = formula code="y_=a*x+(1-a)*y;"("x"=w2167, "y"=w2168, "a"=w2145) -> ("y_"=w2164:dbl)
            n1155 = feedback-in #38(w2164) -> ()
            n1156 = feedback #39() -> (w2166:dbl)  [unwired: 1 in]
            n1157 = formula code="y_=a*x+(1-a)*y;"("x"=w2165, "y"=w2166, "a"=w2145) -> ("y_"=w2163:dbl)
            n1158 = feedback-in #39(w2163) -> ()
            n1159 = feedback #40() -> (w2159:dbl)  [unwired: 1 in]
            n1160 = formula code="y_=a*x+(1-a)*y;"("x"=w2148, "y"=w2159, "a"=w2145) -> ("y_"=w2157:dbl)
            n1161 = feedback-in #40(w2157) -> ()
            n1162 = feedback #41() -> (w2160:dbl)  [unwired: 1 in]
            n1163 = formula code="y_=a*x+(1-a)*y;"("x"=w2149, "y"=w2160, "a"=w2145) -> ("y_"=w2158:dbl)
            n1164 = feedback-in #41(w2158) -> ()
            n1165 = feedback #42() -> (w2173:dbl)  [unwired: 1 in]
            n1166 = formula code="y_=a*x+(1-a)*y;"("x"=w2172, "y"=w2173, "a"=w2145) -> ("y_"=w2171:dbl)
            n1167 = feedback-in #42(w2171) -> ()
            n1168 = feedback #43() -> (w2178:dbl)  [unwired: 1 in]
            n1169 = formula code="y_=a*x+(1-a)*y;"("x"=w2176, "y"=w2178, "a"=w2145) -> ("y_"=w2175:dbl)
            n1170 = feedback-in #43(w2175) -> ()
            n1171 = Bundle("y_"=w2175, "y_"=w2171, "y_"=w2164, "y_"=w2163, "y_"=w2158, "y_"=w2157, "y_"=w2154, "y_"=w2153) -> (→"Radiator Temperature":T5)  [unwired: 1 in]
            n1172 = local read "T Inv. RR [°C]"() -> (w2183:dbl)
            n1173 = local read "T Inv. FL [°C]"() -> (w2180:dbl)
            n1174 = local read "T Inv. FR [°C]"() -> (w2181:dbl)
            n1175 = local read "T Inv. RL [°C]"() -> (w2182:dbl)
            n1176 = local read "T Motor RR [°C]"() -> (w2184:dbl)
            n1177 = local read "T Motor FL [°C]"() -> (w2187:dbl)
            n1178 = local read "T Motor FR [°C]"() -> (w2186:dbl)
            n1179 = local read "T Motor RL [°C]"() -> (w2185:dbl)
            n1180 = Bundle("T Inv. FL [°C]"=w2180, "T Inv. FR [°C]"=w2181, "T Inv. RL [°C]"=w2182, "T Inv. RR [°C]"=w2183) -> (→"Inverter Temperature":T9)  [unwired: 1 in]
            n1181 = Bundle("T Motor FL [°C]"=w2187, "T Motor FR [°C]"=w2186, "T Motor RL [°C]"=w2185, "T Motor RR [°C]"=w2184) -> (→"Motor Temperature":T10)  [unwired: 1 in]
          }
          frame 1058 {
            w2236 = 0.1 ("input variable")
            n1182 = Index Array(array=w2241, index=4) -> (element=w2244:u8)
            n1183 = Index Array(array=w2241, index=5) -> (element=w2245:u8)
            n1184 = Index Array(array=w2241, index=2) -> (element=w2247:u8)
            n1185 = Index Array(array=w2241, index=3) -> (element=w2246:u8)
            n1186 = Join Numbers(hi=w2244, lo=w2245) -> ((hi.lo)=w2203:u16)
            "Wheel Travel RR" <- w2203
            n1187 = Join Numbers(hi=w2247, lo=w2246) -> ((hi.lo)=w2230:u16)
            "Wheel Travel RL" <- w2230
            n1188 = local read "Wheel Travel FL"() -> (w2204:u16)
            n1189 = local read "Wheel Travel FR"() -> (w2208:u16)
            n1190 = Subtract(x=w2230, y="Wheel Travel RL Offset") -> (x-y=w2228:dbl)
            n1191 = Subtract(x=w2204, y="Wheel Travel FL Offset") -> (x-y=w2217:dbl)
            n1192 = Subtract(x=w2203, y="Wheel Travel RR Offset") -> (x-y=w2222:dbl)
            n1193 = Subtract(x=w2208, y="Wheel Travel FR") -> (x-y=w2212:dbl)
            n1194 = Multiply(x=w2228, y=75.0) -> (x*y=w2226:dbl)
            n1195 = Multiply(x=w2217, y=75.0) -> (x*y=w2215:dbl)
            n1196 = Multiply(x=w2222, y=75.0) -> (x*y=w2220:dbl)
            n1197 = Divide(x=w2226, y=4095.0) -> (x/y=→"Damper Travel RL [mm]":dbl)
            n1198 = Divide(x=w2215, y=4095.0) -> (x/y=→"Damper Travel FL [mm]":dbl)
            n1199 = Divide(x=w2220, y=4095.0) -> (x/y=→"Damper Travel RR [mm]":dbl)
            n1200 = Multiply(x=w2212, y=75.0) -> (x*y=w2210:dbl)
            n1201 = Divide(x=w2210, y=4095.0) -> (x/y=→"Damper Travel FR [mm]":dbl)
            n1202 = feedback #44() -> (w2240:dbl)  [unwired: 1 in]
            n1203 = formula code="y_=a*x+(1-a)*y;"("x"=w2230, "y"=w2240, "a"=w2236) -> ("y_"=w2233:dbl)
            n1204 = feedback-in #44(w2233) -> ()
            n1205 = feedback #45() -> (w2239:dbl)  [unwired: 1 in]
            n1206 = formula code="y_=a*x+(1-a)*y;"("x"=w2203, "y"=w2239, "a"=w2236) -> ("y_"=w2232:dbl)
            n1207 = feedback-in #45(w2232) -> ()
            n1208 = feedback #46() -> (w2238:dbl)  [unwired: 1 in]
            n1209 = formula code="y_=a*x+(1-a)*y;"("x"=w2204, "y"=w2238, "a"=w2236) -> ("y_"=w2235:dbl)
            n1210 = feedback-in #46(w2235) -> ()
            n1211 = feedback #47() -> (w2237:dbl)  [unwired: 1 in]
            n1212 = formula code="y_=a*x+(1-a)*y;"("x"=w2208, "y"=w2237, "a"=w2236) -> ("y_"=w2234:dbl)
            n1213 = feedback-in #47(w2234) -> ()
            n1214 = Bundle("y_"=w2235, "y_"=w2234, "y_"=w2233, "y_"=w2232) -> (→"Wheel Travel":cluster{"y_":dbl, "y_":dbl, "y_":dbl, "y_":dbl})  [unwired: 1 in]
          }
          frame 1074 {
            w2276 = u8 127 ("y")
            # "PDM LV Cell Values"
            n1215 = Index Array(array=w2255, index=2) -> (element=w2285:u8)
            n1216 = Index Array(array=w2255, index=3) -> (element=w2277:u8)
            n1217 = Index Array(array=w2255, index=5) -> (element=w2281:u8)
            n1218 = Index Array(array=w2255, index=6) -> (element=w2280:u8)
            n1219 = Greater?(x=w2277, y=w2276) -> (0:w2273:bool)
            n1220 = Join Numbers(hi=w2281, lo=w2280) -> ((hi.lo)=w2279:u16)
            n1221 = And(x=w2277, y=w2276) -> (x .and. y?=w2278:u8)
            n1222 = Decrement(x=w2285) -> (x-1=w2272:u8)
            n1223 = Index Array(array=w2255, index=4) -> (element=w2286:u8)
            n1224 = Join Numbers(hi=w2278, lo=w2286) -> ((hi.lo)=w2284:u16)
            n1225 = Replace Array Subset(array=w2271, new element=w2273, index=w2272) -> (w2269:bool[])
            "Discharge" <- w2269
            n1226 = Replace Array Subset(array=w2268, new element=w2279, index=w2272) -> (w2263:dbl[])
            n1227 = Replace Array Subset(array=w2275, new element=w2284, index=w2272) -> (w2257:u16[])
            n1228 = Divide(x=w2263, y=10.0) -> (x/y=w2261:dbl[])
            "LV Temp" <- w2261
            n1229 = Array To Cluster(array=w2257) -> (cluster=→"LV Cell Voltages":T2)
            n1230 = for {
              tunnel: [w2291] -> w2270 mode=indexing
              tunnel: w2257 -> [w2290] mode=indexing
              n1231 = Bundle(w2290, w2290) -> (w2291:cluster{u16, u16})  [unwired: 1 in]
            }
            "LV Battery" <- w2270
            n1232 = Array Subset(array=w2257, index=0, length=12) -> (w2260:u16[])
            n1233 = Array Max & Min(array=w2261) -> (max value=→"LV Temp":dbl)  [unwired: 3 out]
            n1234 = Array Max & Min(array=w2260) -> (max value=→"LV Max":u16, min value=→"LV Min":u16)  [unwired: 2 out]
          }
          frame 1378 {
            # "Dashboard GPIO States"
            n1235 = Index Array(array=w2301, index=4) -> (element=w2308:u8)
            n1236 = Number To Boolean Array(number=w2308) -> (Boolean array=w2307:bool[])
            n1237 = Index Array(array=w2307, index #1=7 ("index"), index #2=6 ("index"), index #3=5 ("index"), index #4=4 ("index"), index #5=3 ("index"), index #6=2 ("index"), index #7=1 ("index"), index #8=0 ("index")) -> (element #3=→"OFF Button":bool, element #4=→"START Button":bool, element #5=→"ON Button":bool, element #6=→"BLANK":bool, element #7=→"XLAT":bool, element #8=→"MODE":bool)  [unwired: 2 out]
          }
          frame 1105 {
            n1238 = Index Array(array=w2317, index=4) -> (element=w2320:u8)
            n1239 = Index Array(array=w2317, index=5) -> (element=w2321:u8)
            n1240 = Index Array(array=w2317, index=2) -> (element=w2323:u8)
            n1241 = Index Array(array=w2317, index=3) -> (element=w2322:u8)
            n1242 = Join Numbers(hi=w2320, lo=w2321) -> ((hi.lo)=→"Wheel Travel FR":u16)
            n1243 = Join Numbers(hi=w2323, lo=w2322) -> ((hi.lo)=→"Wheel Travel FL":u16)
          }
          frame 1152 {
            n1244 = Array Subset(array=w2334, index=2, length=8) -> (→"CAN Missing Message":u8[])
          }
          frame 1153 {
            # "TCU Status 2"
            n1245 = Index Array(array=w2364, index=3) -> (element=w2390:u8)
            n1246 = Number To Boolean Array(number=w2390) -> (Boolean array=w2407:bool[])
            n1247 = Index Array(array=w2364, index=2) -> (element=→"Max Power":u8)
            n1248 = Index Array(array=w2407, index #1=7 ("index"), index #2=6 ("index"), index #3=5 ("index"), index #4=4 ("index"), index #5=3 ("index"), index #6=2 ("index"), index #7=1 ("index"), index #8=0 ("index")) -> (element #1=→"Safety Mode Enabled":bool, element #2=→"Power Limiter Enabled":bool, element #3=→"Keylock Enable":bool, element #4=→"Throttle_Constant":bool, element #5=→"SlipControl_Enabled":bool, element #6=→"Torque_Coeff":bool, element #7=→"Torque_Derate":bool, element #8=→"Smooth_Transition_Enabled":bool)
            n1249 = Index Array(array=w2364, index=7) -> (element=w2378:u8)
            n1250 = Index Array(array=w2364, index=6) -> (element=w2340:u8)
            n1251 = Index Array(array=w2364, index=8) -> (element=w2358:u8)
            n1252 = Index Array(array=w2364, index=9) -> (element=w2361:u8)
            n1253 = Join Numbers(hi=w2340, lo=w2378) -> ((hi.lo)=w2376:u16)
            n1254 = Join Numbers(hi=w2358, lo=w2361) -> ((hi.lo)=w2360:u16)
            n1255 = And(x=w2376, y=u16 2047) -> (x .and. y?=w2375:u16)
            n1256 = And(x=w2360, y=u16 511) -> (x .and. y?=w2346:u16)
            n1257 = To Double Precision Float(number=100 ("index")) -> (double precision float=w2343:dbl)
            n1258 = To Word Integer(number=w2375) -> (16bit integer=→"Offset":i16)
            n1259 = To Double Precision Float(number=w2346) -> (double precision float=w2345:dbl)
            n1260 = And(x=w2358, y=u8 248) -> (x .and. y?=w2356:u8)
            n1261 = Index Array(array=w2364, index=4) -> (element=w2386:u8)
            n1262 = Index Array(array=w2364, index=5) -> (element=w2372:u8)
            n1263 = To Double Precision Float(number=w2356) -> (double precision float=w2355:dbl)
            n1264 = Divide(x=w2345, y=1000.0) -> (x/y=w2350:dbl)
            n1265 = To Double Precision Float(number=w2340) -> (double precision float=w2341:dbl)
            n1266 = Divide(x=w2355, y=8.0) -> (x/y=w2353:dbl)
            n1267 = Divide(x=w2386, y=10 ("index")) -> (x/y=→"Drop":dbl)
            n1268 = Multiply(x=w2350, y=5.0) -> (x*y=→"Hardcore Time":dbl)
            n1269 = Divide(x=w2341, y=w2343) -> (x/y=→"DesiredSlipRate":dbl)
            n1270 = Multiply(x=w2353, y=1000.0) -> (x*y=→"PowerLimiter Approx":dbl)
            n1271 = Number To Boolean Array(number=w2372) -> (Boolean array=w2371:bool[])
            n1272 = And(x=w2372, y=u8 240) -> (x .and. y?=w2383:u8)
            n1273 = To Double Precision Float(number=w2383) -> (double precision float=w2382:dbl)
            n1274 = Divide(x=w2382, y=16.0) -> (x/y=→"Characteristics Approx":dbl)
            n1275 = Index Array(array=w2371, index #1=3 ("index"), index #2=2 ("index"), index #3=1 ("index")) -> (element #1=→"AMK_AV":bool, element #2=→"Torque 2":bool, element #3=→"Hardcoremode ON":bool)
          }
          frame 1154 {
            n1276 = Index Array(array=w2520, index=4) -> (element=w2513:u8)
            n1277 = Index Array(array=w2520, index=5) -> (element=w2478:u8)
            n1278 = Index Array(array=w2520, index=2) -> (element=w2517:u8)
            n1279 = Index Array(array=w2520, index=3) -> (element=w2495:u8)
            n1280 = Index Array(array=w2520, index=6) -> (element=w2417:u8)
            n1281 = Index Array(array=w2520, index=7) -> (element=w2461:u8)
            n1282 = Index Array(array=w2520, index=8) -> (element=w2434:u8)
            n1283 = Index Array(array=w2520, index=9) -> (element=w2446:u8)
            n1284 = To Unsigned Byte Integer(number=w2517) -> (unsigned 8bit integer=w2519:u8)
            n1285 = To Unsigned Byte Integer(number=w2513) -> (unsigned 8bit integer=w2515:u8)
            n1286 = Equal?(x=u8 1, y=w2519) -> (x = y?=→"Message Arrived":bool)
            n1287 = Equal?(x=u8 2, y=w2515) -> (x = y?=→"Message Arrived 2":bool)
            n1288 = Number To Boolean Array(number=w2495) -> (Boolean array=w2511:bool[])
            n1289 = Number To Boolean Array(number=w2478) -> (Boolean array=w2494:bool[])
            n1290 = Number To Boolean Array(number=w2434) -> (Boolean array=w2437:bool[])
            n1291 = Index Array(array=w2511, index #1=7 ("index"), index #2=6 ("index"), index #3=5 ("index"), index #4=4 ("index"), index #5=3 ("index"), index #6=2 ("index"), index #7=1 ("index"), index #8=0 ("index")) -> (element #2=→"Error_ThrottleValidity_1_raw 2":bool, element #3=→"Error_ThrottleValidity_2_raw 2":bool, element #4=→"Error Throttle Position 1":bool, element #5=→"Error Throttle Position 2":bool, element #6=→"Error Throttle Validity 1":bool, element #7=→"Error Throttle Validity 2":bool, element #8=→"Error Throttle Plausability":bool)  [unwired: 1 out]
            n1292 = Index Array(array=w2437, index #1=7 ("index"), index #2=6 ("index"), index #3=5 ("index"), index #4=4 ("index"), index #5=3 ("index"), index #6=2 ("index"), index #7=1 ("index"), index #8=0 ("index")) -> (element #7=→"Error_LVCellVoltage":bool, element #8=→"Error_LVCellTemperature":bool)  [unwired: 6 out]
            n1293 = Index Array(array=w2494, index #1=7 ("index"), index #2=6 ("index"), index #3=5 ("index"), index #4=4 ("index"), index #5=3 ("index"), index #6=2 ("index"), index #7=1 ("index"), index #8=0 ("index")) -> (element #2=→"Error_BrakeValidity_1_raw  2":bool, element #3=→"Error_BrakeValidity_2_raw 2":bool, element #4=→"Error Brake Position 1":bool, element #5=→"Error Brake Position 2":bool, element #6=→"Error Brake Validity  1":bool, element #7=→"Error Brake Validity 2":bool, element #8=→"Error Brake Plausability":bool)  [unwired: 1 out]
            n1294 = Number To Boolean Array(number=w2417) -> (Boolean array=w2419:bool[])
            n1295 = Index Array(array=w2419, index #1=7 ("index"), index #2=6 ("index"), index #3=5 ("index"), index #4=4 ("index"), index #5=3 ("index"), index #6=2 ("index"), index #7=1 ("index"), index #8=0 ("index")) -> (element #1=→"Error_BrakeValidity_1_raw":bool, element #2=→"Error_BrakeValidity_2_raw":bool, element #3=→"Error_ThrottleValidity_1_raw":bool, element #4=→"Error_ThrottleValidity_2_raw":bool, element #5=→"Error_SteeringAngleValidity_1_raw":bool, element #6=→"Error_SteeringAngleValidity_2_raw":bool, element #7=→"Error_Pedalbox_Heartbeat_raw":bool, element #8=→"Error_SteeringControl_Heartbeat_raw":bool)
            n1296 = Number To Boolean Array(number=w2461) -> (Boolean array=w2477:bool[])
            n1297 = Number To Boolean Array(number=w2446) -> (Boolean array=w2460:bool[])
            n1298 = Index Array(array=w2477, index #1=7 ("index"), index #2=6 ("index"), index #3=5 ("index"), index #4=4 ("index"), index #5=3 ("index"), index #6=2 ("index"), index #7=1 ("index"), index #8=0 ("index")) -> (element #2=→"Error_SteeringAngleValidity_1_raw 2":bool, element #3=→"Error_SteeringAngleValidity_2_raw 2":bool, element #4=→"Error Steering Angle 1":bool, element #5=→"Error Steering Angle 2":bool, element #6=→"Error Steering Validity 1":bool, element #7=→"Error Steering Validity 2":bool, element #8=→"Error Steering Plausability":bool)  [unwired: 1 out]
            n1299 = Index Array(array=w2460, index #1=7 ("index"), index #2=6 ("index"), index #3=5 ("index"), index #4=4 ("index"), index #5=3 ("index"), index #6=2 ("index"), index #7=1 ("index"), index #8=0 ("index")) -> (element #4=→"Error HV Accu. Voltage":bool, element #5=→"Error HV Accu. Current":bool, element #6=→"Error Cell Voltage":bool, element #7=→"Error Cell Voltage Sensor":bool, element #8=→"Error Cell Temperature":bool)  [unwired: 3 out]
          }
          frame 1155 {
            n1300 = Index Array(array=w2538, index=3) -> (element=w2612:u8)
            n1301 = Index Array(array=w2538, index=2) -> (element=w2551:u8)
            n1302 = Index Array(array=w2538, index=4) -> (element=w2547:u8)
            n1303 = Index Array(array=w2538, index=5) -> (element=w2601:u8)
            n1304 = Index Array(array=w2538, index=7) -> (element=w2590:u8)
            n1305 = To Unsigned Byte Integer(number=w2547) -> (unsigned 8bit integer=w2550:u8)
            n1306 = Number To Boolean Array(number=w2612) -> (Boolean array=w2621:bool[])
            n1307 = To Unsigned Byte Integer(number=w2551) -> (unsigned 8bit integer=w2554:u8)
            n1308 = Index Array(array=w2538, index=6) -> (element=w2543:u8)
            n1309 = Number To Boolean Array(number=w2601) -> (Boolean array=w2610:bool[])
            n1310 = Equal?(x=u8 14, y=w2550) -> (x = y?=→"Message Arrived 12":bool)
            n1311 = Number To Boolean Array(number=w2590) -> (Boolean array=w2599:bool[])
            n1312 = Equal?(x=u8 13, y=w2554) -> (x = y?=→"Message Arrived 11":bool)
            n1313 = To Unsigned Byte Integer(number=w2543) -> (unsigned 8bit integer=w2546:u8)
            n1314 = Equal?(x=u8 15, y=w2546) -> (x = y?=→"Message Arrived 13":bool)
            n1315 = Index Array(array=w2621, index #1=7 ("index"), index #2=6 ("index"), index #3=5 ("index"), index #4=4 ("index"), index #5=3 ("index"), index #6=2 ("index"), index #7=1 ("index"), index #8=0 ("index")) -> (element #3=→"FL TargetVelo OverTresh":bool, element #4=→"FL TargetVelo UnderTresh":bool, element #5=→"FL TorqueLimPos OverTresh":bool, element #6=→"FL TorqueLimPos UnderTresh":bool, element #7=→"FL TorqueLimNeg OverTresh":bool, element #8=→"FL TorqueLimNeg UnderTresh":bool)  [unwired: 2 out]
            n1316 = Index Array(array=w2610, index #1=7 ("index"), index #2=6 ("index"), index #3=5 ("index"), index #4=4 ("index"), index #5=3 ("index"), index #6=2 ("index"), index #7=1 ("index"), index #8=0 ("index")) -> (element #3=→"FR TargetVelo OverTresh":bool, element #4=→"FR TargetVelo UnderTresh":bool, element #5=→"FR TorqueLimPos OverTresh":bool, element #6=→"FR TorqueLimPos UnderTresh":bool, element #7=→"FR TorqueLimNeg OverTresh":bool, element #8=→"FR TorqueLimNeg UnderTresh":bool)  [unwired: 2 out]
            n1317 = Index Array(array=w2599, index #1=7 ("index"), index #2=6 ("index"), index #3=5 ("index"), index #4=4 ("index"), index #5=3 ("index"), index #6=2 ("index"), index #7=1 ("index"), index #8=0 ("index")) -> (element #3=→"RL TargetVelo OverTresh":bool, element #4=→"RL TargetVelo UnderTresh":bool, element #5=→"RL TorqueLimPos OverTresh":bool, element #6=→"RL TorqueLimPos UnderTresh":bool, element #7=→"RL TorqueLimNeg OverTresh":bool, element #8=→"RL TorqueLimNeg UnderTresh":bool)  [unwired: 2 out]
            n1318 = Index Array(array=w2538, index=8) -> (element=w2539:u8)
            n1319 = Index Array(array=w2538, index=9) -> (element=w2555:u8)
            n1320 = To Unsigned Byte Integer(number=w2539) -> (unsigned 8bit integer=w2542:u8)
            n1321 = Number To Boolean Array(number=w2555) -> (Boolean array=w2588:bool[])
            n1322 = Equal?(x=u8 16, y=w2542) -> (x = y?=→"Message Arrived 14":bool)
            n1323 = Index Array(array=w2588, index #1=7 ("index"), index #2=6 ("index"), index #3=5 ("index"), index #4=4 ("index"), index #5=3 ("index"), index #6=2 ("index"), index #7=1 ("index"), index #8=0 ("index")) -> (element #3=→"RR TargetVelo OverTresh":bool, element #4=→"RR TargetVelo UnderTresh":bool, element #5=→"RR TorqueLimPos OverTresh":bool, element #6=→"RR TorqueLimPos UnderTresh":bool, element #7=→"RR TorqueLimNeg OverTresh":bool, element #8=→"RR TorqueLimNeg UnderTresh":bool)  [unwired: 2 out]
          }
          frame 1156 {
            n1324 = Index Array(array=w2643, index=7) -> (element=w2693:u8)
            n1325 = Index Array(array=w2643, index=6) -> (element=w2697:u8)
            n1326 = Index Array(array=w2643, index=8) -> (element=w2694:u8)
            n1327 = Index Array(array=w2643, index=9) -> (element=w2642:u8)
            n1328 = To Unsigned Byte Integer(number=w2642) -> (unsigned 8bit integer=w2639:u8)
            n1329 = Number To Boolean Array(number=w2697) -> (Boolean array=w2738:bool[])
            n1330 = Number To Boolean Array(number=w2694) -> (Boolean array=w2715:bool[])
            n1331 = Number To Boolean Array(number=w2693) -> (Boolean array=w2724:bool[])
            n1332 = Equal?(x=17 ("index"), y=w2639) -> (x = y?=→"Other messages arrived":bool)
            n1333 = Index Array(array=w2738, index #1=7 ("index"), index #2=6 ("index"), index #3=5 ("index"), index #4=4 ("index"), index #5=3 ("index"), index #6=2 ("index"), index #7=1 ("index"), index #8=0 ("index")) -> (element #4=→"Error Rot Switch 1":bool, element #5=→"Error Rot Switch 2":bool, element #6=→"Error Rot Switch 3":bool, element #7=→"Error Rot Switch 4":bool, element #8=→"Error Rot Switch 5":bool)  [unwired: 3 out]
            n1334 = Index Array(array=w2715, index #1=7 ("index"), index #2=6 ("index"), index #3=5 ("index"), index #4=4 ("index"), index #5=3 ("index"), index #6=2 ("index"), index #7=1 ("index"), index #8=0 ("index")) -> (element #3=→"CriticalHVCell Heartbeat raw":bool, element #4=→"CriticalHVCell Heartbeat":bool, element #5=→"Error_Button_4":bool, element #6=→"Error_Button_3":bool, element #7=→"Error_Button_2":bool, element #8=→"Error_Button_1":bool)  [unwired: 2 out]
            n1335 = Index Array(array=w2724, index #1=7 ("index"), index #2=6 ("index"), index #3=5 ("index"), index #4=4 ("index"), index #5=3 ("index"), index #6=2 ("index"), index #7=1 ("index"), index #8=0 ("index")) -> (element #1=→"Error BrPressure Front Validity":bool, element #2=→"Error BrPressure Rear Validity":bool, element #3=→"Error BrPressure Front":bool, element #4=→"Error BrPressure Rear 2":bool, element #5=→"Error BrPressure Front Validity_raw":bool, element #6=→"Error BrPressure Rear Validity_raw":bool, element #7=→"Error Steering Heartbeat":bool, element #8=→"Error Pedalbox Heartbeat":bool)
            n1336 = Index Array(array=w2643, index=2) -> (element=w2645:u8)
            n1337 = Index Array(array=w2643, index=3) -> (element=w2646:u8)
            n1338 = Index Array(array=w2643, index=4) -> (element=w2647:u8)
            n1339 = Index Array(array=w2643, index=5) -> (element=w2648:u8)
            n1340 = Number To Boolean Array(number=w2645) -> (Boolean array=w2692:bool[])
            n1341 = Number To Boolean Array(number=w2646) -> (Boolean array=w2682:bool[])
            n1342 = Number To Boolean Array(number=w2647) -> (Boolean array=w2672:bool[])
            n1343 = Number To Boolean Array(number=w2648) -> (Boolean array=w2662:bool[])
            n1344 = Index Array(array=w2692, index #1=7 ("index"), index #2=6 ("index"), index #3=5 ("index"), index #4=4 ("index"), index #5=3 ("index"), index #6=2 ("index"), index #7=1 ("index"), index #8=0 ("index")) -> (element #8=→"Error Actual Velocity FL":bool)  [unwired: 7 out]
            n1345 = Index Array(array=w2682, index #1=7 ("index"), index #2=6 ("index"), index #3=5 ("index"), index #4=4 ("index"), index #5=3 ("index"), index #6=2 ("index"), index #7=1 ("index"), index #8=0 ("index")) -> (element #8=→"Error Actual Velocity FR":bool)  [unwired: 7 out]
            n1346 = Index Array(array=w2672, index #1=7 ("index"), index #2=6 ("index"), index #3=5 ("index"), index #4=4 ("index"), index #5=3 ("index"), index #6=2 ("index"), index #7=1 ("index"), index #8=0 ("index")) -> (element #8=→"Error Actual Velocity RL":bool)  [unwired: 7 out]
            n1347 = Index Array(array=w2662, index #1=7 ("index"), index #2=6 ("index"), index #3=5 ("index"), index #4=4 ("index"), index #5=3 ("index"), index #6=2 ("index"), index #7=1 ("index"), index #8=0 ("index")) -> (element #8=→"Error Actual Velocity RR":bool)  [unwired: 7 out]
          }
          frame 1157 {
            n1348 = Index Array(array=w2751, index=4) -> (element=w2771:u8)
            n1349 = Index Array(array=w2751, index=3) -> (element=w2772:u8)
            n1350 = Index Array(array=w2751, index=5) -> (element=w2768:u8)
            n1351 = Index Array(array=w2751, index=2) -> (element=w2747:u8)
            n1352 = Index Array(array=w2751, index=8) -> (element=w2756:u8)
            n1353 = Index Array(array=w2751, index=6) -> (element=w2764:u8)
            n1354 = Index Array(array=w2751, index=9) -> (element=w2752:u8)
            n1355 = Index Array(array=w2751, index=7) -> (element=w2760:u8)
            n1356 = To Double Precision Float(number=w2768) -> (double precision float=w2769:dbl)
            n1357 = To Double Precision Float(number=w2771) -> (double precision float=w2770:dbl)
            n1358 = To Long Integer(number=w2756) -> (32bit integer=w2757:i32)
            n1359 = To Long Integer(number=w2764) -> (32bit integer=w2765:i32)
            n1360 = To Long Integer(number=w2752) -> (32bit integer=w2753:i32)
            n1361 = Divide(x=w2769, y=100.0 ("index")) -> (x/y=→"Efficiency":dbl)
            n1362 = To Long Integer(number=w2760) -> (32bit integer=w2761:i32)
            n1363 = Divide(x=w2770, y=100.0 ("index")) -> (x/y=→"Tune":dbl)
            n1364 = Multiply(x=w2757, y=10 ("index")) -> (x*y=w2741:i32)
            "Fz_RL" <- w2741
            n1365 = Multiply(x=w2765, y=10 ("index")) -> (x*y=w2743:i32)
            "Fz_FL" <- w2743
            n1366 = Multiply(x=w2753, y=10 ("index")) -> (x*y=w2740:i32)
            "Fz_RR" <- w2740
            n1367 = Multiply(x=w2761, y=10 ("index")) -> (x*y=w2742:i32)
            "Fz_FR" <- w2742
            n1368 = To Long Integer(number=w2747) -> (32bit integer=w2746:i32)
            n1369 = To Double Precision Float(number=4 ("index")) -> (double precision float=w2824:dbl)
            n1370 = And(x=w2746, y=3 ("index")) -> (x .and. y?=→"YawControlSelector":i32)
            n1371 = To Double Precision Float(number=w2772) -> (double precision float=w2825:dbl)
            n1372 = To Double Precision Float(number=w2772) -> (double precision float=w2815:dbl)
            n1373 = To Double Precision Float(number=w2772) -> (double precision float=w2797:dbl)
            n1374 = To Double Precision Float(number=w2772) -> (double precision float=w2780:dbl)
            n1375 = To Double Precision Float(number=w2772) -> (double precision float=w2806:dbl)
            n1376 = To Double Precision Float(number=w2772) -> (double precision float=w2789:dbl)
            n1377 = Bundle(w2743, w2742, w2741, w2740) -> (→"Fz Estimation":cluster{i32, i32, i32, i32})  [unwired: 1 in]
            n1378 = To Long Integer(number=w2772) -> (32bit integer=w2826:i32)
            n1379 = Divide(x=w2825, y=w2824) -> (x/y=w2821:dbl)
            n1380 = To Long Integer(number=w2821) -> (32bit integer=w2822:i32)
            n1381 = To Double Precision Float(number=8 ("index")) -> (double precision float=w2814:dbl)
            n1382 = To Double Precision Float(number=32 ("index")) -> (double precision float=w2796:dbl)
            n1383 = To Double Precision Float(number=128 ("index")) -> (double precision float=w2779:dbl)
            n1384 = To Double Precision Float(number=16 ("index")) -> (double precision float=w2805:dbl)
            n1385 = To Double Precision Float(number=64 ("index")) -> (double precision float=w2788:dbl)
            n1386 = And(x=w2822, y=1 ("index")) -> (x .and. y?=w2818:i32)
            n1387 = Divide(x=w2815, y=w2814) -> (x/y=w2811:dbl)
            n1388 = Divide(x=w2797, y=w2796) -> (x/y=w2745:dbl)
            n1389 = Divide(x=w2780, y=w2779) -> (x/y=w2776:dbl)
            n1390 = Divide(x=w2806, y=w2805) -> (x/y=w2802:dbl)
            n1391 = Divide(x=w2789, y=w2788) -> (x/y=w2785:dbl)
            n1392 = And(x=w2826, y=3 ("index")) -> (x .and. y?=→"Weight":i32)
            n1393 = To Long Integer(number=w2811) -> (32bit integer=w2812:i32)
            n1394 = To Long Integer(number=w2776) -> (32bit integer=w2777:i32)
            n1395 = To Long Integer(number=w2802) -> (32bit integer=w2803:i32)
            n1396 = To Long Integer(number=w2785) -> (32bit integer=w2786:i32)
            n1397 = Round Toward -Infinity(1:w2745) -> (0:w2744:dbl)
            n1398 = And(x=w2812, y=1 ("index")) -> (x .and. y?=w2809:i32)
            n1399 = To Long Integer(number=w2744) -> (32bit integer=w2794:i32)
            n1400 = And(x=w2777, y=1 ("index")) -> (x .and. y?=w2774:i32)
            n1401 = And(x=w2803, y=1 ("index")) -> (x .and. y?=w2800:i32)
            n1402 = And(x=w2786, y=1 ("index")) -> (x .and. y?=w2783:i32)
            n1403 = Equal?(x=w2818, y=1 ("index")) -> (x = y?=→"Eff_PowLim":bool)
            n1404 = And(x=w2794, y=1 ("index")) -> (x .and. y?=w2792:i32)
            n1405 = Equal?(x=w2809, y=1 ("index")) -> (x = y?=→"Fx_Divide_ON":bool)
            n1406 = Equal?(x=w2792, y=1 ("index")) -> (x = y?=→"Sensorbox_Plausibility_Check":bool)
            n1407 = Equal?(x=w2774, y=1 ("index")) -> (x = y?=→"SensorBox_Front_RangeCheck":bool)
            n1408 = Equal?(x=w2800, y=1 ("index")) -> (x = y?=→"Yaw_Control_ON":bool)
            n1409 = Equal?(x=w2783, y=1 ("index")) -> (x = y?=→"SensorBox_Rear_RangeCheck":bool)
            "Array" <- w2751
          }
          frame 1184 {
            # "Charger Status"
            n1410 = Index Array(array=w2849, index=3) -> (element=w2850:u8)
            n1411 = Number To Boolean Array(number=w2850) -> (Boolean array=w2848:bool[])
            n1412 = Index Array(array=w2848, index #1=7 ("index"), index #2=6 ("index"), index #3=5 ("index"), index #4=4 ("index"), index #5=3 ("index"), index #6=2 ("index"), index #7=1 ("index")) -> ()  [unwired: 7 out]
          }
          frame 1185 {
            # "Charger Status 2"
            n1413 = Index Array(array=w2873, index=8) -> (element=w2875:u8)
            n1414 = Index Array(array=w2873, index=9) -> (element=w2874:u8)
            n1415 = Index Array(array=w2873, index=2) -> (element=w2892:u8)
            n1416 = Index Array(array=w2873, index=3) -> (element=w2891:u8)
            n1417 = Index Array(array=w2873, index=6) -> (element=w2879:u8)
            n1418 = Index Array(array=w2873, index=7) -> (element=w2878:u8)
            n1419 = Index Array(array=w2873, index=4) -> (element=w2883:u8)
            n1420 = Index Array(array=w2873, index=5) -> (element=w2882:u8)
            n1421 = Join Numbers(hi=w2875, lo=w2874) -> ((hi.lo)=w2861:u16)
            n1422 = Join Numbers(hi=w2892, lo=w2891) -> ((hi.lo)=w2870:u16)
            n1423 = Join Numbers(hi=w2879, lo=w2878) -> ((hi.lo)=w2864:u16)
            n1424 = Join Numbers(hi=w2883, lo=w2882) -> ((hi.lo)=w2867:u16)
            n1425 = To Double Precision Float(number=w2861) -> (double precision float=w2862:dbl)
            n1426 = To Double Precision Float(number=w2870) -> (double precision float=w2871:dbl)
            n1427 = To Double Precision Float(number=w2864) -> (double precision float=w2865:dbl)
            n1428 = To Double Precision Float(number=w2867) -> (double precision float=w2868:dbl)
            n1429 = Divide(x=w2862, y=10.0) -> (x/y=→"Voltage Limit":dbl)
            n1430 = Divide(x=w2865, y=10.0) -> (x/y=→"Charge Voltage":dbl)
            n1431 = Divide(x=w2871, y=100.0) -> (x/y=→"Charge Curr":dbl)
            n1432 = Divide(x=w2868, y=100.0) -> (x/y=→"Current Limit":dbl)
          }
        }
      }
      n1433 = And(x=w79, y=w75) -> (x .and. y?=w80:bool)
      n1434 = Not(x=w75) -> (.not. x?=w76:bool)
      n1435 = And(x=w77, y=w76) -> (x .and. y?=w78:bool)
      n1436 = case shown="True" "Log Enable" {
        tunnel: w88 -> [_ w186]
        tunnel: w81 -> [_ w185]
        frame False {
        }
        frame True {
          n1437 = for {
            tunnel: w185 -> [w193] mode=indexing
            tunnel: [w191] -> w184 mode=indexing
            n1438 = Get Date/Time In Seconds() -> (seconds since 1Jan1904=w189:timestamp)
            n1439 = Format Date/Time String(time format string (%c)="%Y.%m.%d. %H:%M:%S%3u", seconds (now)=w189) -> (date/time string=w192:string)  [unwired: 1 in]
            n1440 = Number To Decimal String(number=w193) -> (decimal integer string=w190:string[])  [unwired: 1 in]
            n1441 = Build Array (concatenate)(w192, w190) -> (w191:string[])
          }
          n1442 = call-poly <vilib>:"Write To Spreadsheet File.vi"("delimiter (\\t)"=";" ("delimiter (\\t)"), "append to file? (new file:F)"=TRUE, "2D data"=w184, "file path (dialog if empty)"=w186) -> ()  [unwired: 4 in, 1 out]
        }
      }
      n1443 = case shown="True" w80 {
        frame False {
        }
        frame True {
          n1444 = property on="Tab Control" class="TabCtl (strict)"("FG Color"=u32 16711680 ("Colors:FG Color")) -> ()  [unwired: 2 in, 2 out]
        }
      }
      n1445 = case shown="True" w78 {
        frame False {
        }
        frame True {
          n1446 = property on="Tab Control" class="TabCtl (strict)"("FG Color"=u32 11776947 ("Colors:FG Color")) -> ()  [unwired: 2 in, 2 out]
        }
      }
      n1447 = flat-sequence {
        tunnel: w90 -> [w194]
        tunnel: w81 -> [w195]
        frame #0 {
          "CAN ID" <- w194
          "CAN Message" <- w195
          "CAN ID 2" <- w194
          "CAN Message 2" <- w195
          "CAN ID 3" <- w194
          "CAN Message 3" <- w195
        }
      }
      n1448 = Compound Arithmetic op=OR("stop", "Exit") -> (w70:bool)
    }
    n1449 = local read "Exit"() -> (w2:bool)
  }
